vi "Main_V4.4.vi"() -> ()   [LabVIEW 2024]
uses:
  Facility_control_labview/Main_V3.0 Folder/Main_V3.0 Folder/C/Users/alexa/NewOrbit Dropbox/Alexander Schwertheim/PC (2)/Documents/Lab_hardware/Facility_control/Facility_control_labview/Controls/Turbo_Control_Mode.ctl
  Facility_control_labview/Main_V3.0 Folder/Main_V3.0 Folder/C/Users/alexa/NewOrbit Dropbox/Alexander Schwertheim/PC (2)/Documents/Lab_hardware/Facility_control/Facility_control_labview/Controls/Current_Facility_State.ctl
  Facility_control_labview/Main_V3.0 Folder/Main_V3.0 Folder/C/Users/alexa/NewOrbit Dropbox/Alexander Schwertheim/PC (2)/Documents/Lab_hardware/Facility_control/Facility_control_labview/Controls/Facility_State.ctl
  Facility_control_labview/Main_V3.0 Folder/Main_V3.0 Folder/C/Program Files/National Instruments/LabVIEW 2023/instr.lib/Pfeiffer Vacuum/Public/Turbopumps/PV Operating adjustment - Cluster.ctl
  Facility_control_labview/Main_V3.0 Folder/Main_V3.0 Folder/C/Program Files/National Instruments/LabVIEW 2023/instr.lib/Pfeiffer Vacuum/Public/Turbopumps/PV Miscellaneous - Cluster.ctl
  <vilib>/DAQmx/read.llb/DAQmx Read (Analog Wfm 1Chan 1Samp).vi
  <vilib>/DAQmx/read.llb/DAQmx Read (Digital Bool 1Line 1Point).vi
  <vilib>/DAQmx/read.llb/DAQmx Read (Analog 1D Wfm NChan NSamp).vi
  <vilib>/Analysis/baseanly.llb/Mean (DBL).vi
  <vilib>/DAQmx/read.llb/DAQmx Read (Digital 1D Bool NChan 1Samp 1Line).vi
  8e44a3b5-8466-4d68-80f5-cecf70b24b4a.vi
  <vilib>/DAQmx/write.llb/DAQmx Write (Digital Bool 1Line 1Point).vi
  <vilib>/DAQmx/write.llb/DAQmx Write (Digital 1D Bool NChan 1Samp 1Line).vi
  Program Files/National Instruments/LabVIEW 2023/instr.lib/U1250 Series Multimeter Device Driver/Public/Configure/Low Level/DC Voltage Configuration.vi
  <vilib>/DAQmx/create/channels.llb/DAQmx Create Channel (AI-Voltage-Basic).vi
  <vilib>/DAQmx/miscellaneous.llb/DAQmx Fill In Error Info.vi
  <vilib>/DAQmx/create/channels.llb/DAQmx Create Channel (DO-Digital Output).vi
  <vilib>/DAQmx/create/channels.llb/DAQmx Create Channel (DI-Digital Input).vi
  <vilib>/DAQmx/configure/timing.llb/DAQmx Timing (Sample Clock).vi
  Program Files/National Instruments/LabVIEW 2023/instr.lib/U1250 Series Multimeter Device Driver/Controls/Voltage Range.ctl
  Facility_control_labview/Main_V3.0 Folder/Main_V3.0 Folder/C/Program Files/National Instruments/LabVIEW 2023/instr.lib/Pfeiffer Vacuum/Pfeiffer Vacuum.lvlib
  <resource>/objmgr/daqmx.rc
  <vilib>/Analysis/NI_AALBase.lvlib
  Program Files/National Instruments/LabVIEW 2023/instr.lib/U1250 Series Multimeter Device Driver/U1250 Series Digital Multimeter.lvlib
panel:
  in  "Change to Auto":bool
  out "Turbo_Standby_Sys_Cmd":bool
  out "Measurement":dbl format="%#_8f"
  in  "ON/OFF":bool
  in  "DMM VISA resource name COM4":refnum<visa-resource-name>="COM4"
  in  "use DMM?":bool
  in  "samples per channel":i32=200
  in  "rate":dbl=1000.0 format="%#_13g"
  out "Com Potential (V)":dbl
  in  "Turbo on Threshold (torr) 2":dbl=0.25 format="%#_13g"
  out "Current Time/date":string
  out "String 3":string
  out "Vent Time (s) 2":dbl caption="Elapsed Time (s)"
  out "Numeric":dbl
  out "Elapsed Time (s)":dbl
  out "Turbo on Threshold (torr)":dbl=0.08
  out "Turbo Convectron":dbl=627.9033934565941 format="%_3e"
  out "Still Spinning?":bool
  out "Turbo Error Aknowleged 2":bool
  in  "Valve_Gate_User_Cmd":bool
  out "Tubro_Control_Mode":T1
  out "String":string
  out "Gate Valve Error?":bool
  out "Gate Valve":bool
  out "Valve_Gate_Sys_Cmd":bool
  out "Turbo Speed":string="0"
  out "Turbo bottom Temp":string="20"
  out "Turbo bearing Temp":string="21"
  out "Turbo Motor Temp":string="20"
  in  "Valve_Vent_User_Cmd":bool
  out "Vent Valve Error?":bool
  in  "Turbo_Error_Acknowlege_Cmd 2":bool
  in  "Valve_Bypass_User_Cmd":bool
  in  "Primary_User_Cmd":bool
  out "Primary Status":u32(colorbox)=12632256
  out "Bypass Valve Error?":bool
  in  "Turbo_Motor_User_Cmd":bool
  in  "Chiller_User_Cmd":bool
  out "Bypass Valve":bool
  out "Vent Valve":bool
  out "Primary Pump Status":string="Primary Pump is Off"
  out "Wide Range Gauge Pressure (Torr)":dbl=nan format="%_3e"
  out "Foreline Convectron":dbl=627.9033934565941 format="%_3e"
  out "Chiller Status":string="Chiller is Off"
  out "Turbo Status":string="Turbo Off"
  out "Turbo Error Aknowleged":bool
  out "Chiller Status 2":u32(colorbox)=12632256
  out "Turbo Status Color":u32(colorbox)=12632256
  in  "stop":bool
  out "error out":errorcluster
  out "Control Level":enum32{"Admin", "Debug", "Automatic"}(tab)=enum."Automatic"
  in  "Fake_Chiller_Read":bool
  in  "Fake_Convec_2_Pressure_Torr":dbl=0.0001 format="%_3e"
  in  "Fake_Primary_Pump_Read":bool
  in  "Fake_Valve_Turbo_Read":bool
  in  "Fake_Valve_Bypass_Read":bool
  in  "Fake_Valve_Vent_Read":bool
  in  "Use fake values?":bool=TRUE
  in  "Fake_Convec_1_Pressure_Torr":dbl=0.001 format="%_3e"
  in  "Fake Turbo Motor Read":bool
  in  "Fake Turbo Speed Read (%)":dbl=0.0001 format="%#.3f"
  in  "Fake Turbo Error Read":bool
  in  "Fake_Valve_Gate_Read":bool
  in  "Fake_WRG_Pressure_Torr":dbl=1e-05 format="%_3e"
  in  "Turbo Engage time":timestamp=timestamp(3765222000 s since 1904-01-01)
  out "Current Facility State":T2=enum."Pumping to Rough"
  out "Target Facility State":T2=enum."Pumping to Rough"
  out "Tab Control":T3(tab)
  in  "Pump to High Vac":bool
  in  "Pump to Rough":bool
  in  "Overnight Pump":bool
  in  "Vent":bool
  in  "Skip Primary Warm":bool
  in  "Vent 2":bool
  in  "Shut Off":bool
  in  "Overnight Pump 3":bool
  in  "Pump to Rough Only":bool
  in  "Pump to High":bool
  in  "Vent 4":bool
  in  "Pump to Rough 3":bool
  in  "Pump to High Vac 3":bool
  in  "Vent 5":bool
  in  "Shutdown":bool
  in  "Pump to Rough 4":bool
  in  "Overnight Pump 2":bool
  in  "Vent and shutdonw":bool
  in  "Shut Off":bool
  in  "Pump to Hi vac":bool
  in  "Overnight Pump 5":bool
  in  "Pump to Rough 5":bool
  in  "Pump to High Vac 2":bool
  in  "change_to_admin_mode":bool
  in  "Clear error?":bool
  out "Running":bool
  out "Waveform Chart 2":waveform(dbl)[](graph)=[{"t0"=timestamp(3754409348.7178025 s since 1904-01-01), "dt"=0.1, "Y"=array[1789 elements]}, {"t0"=timestamp(3754409348.7178025 s since 1904-01-01), "dt"=0.1, "Y"=array[1789 elements]}, {"t0"=timestamp(3754409348.7178025 s since 1904-01-01), "dt"=0.1, "Y"=array[1789 elements]}, {"t0"=timestamp(3754409348.7178025 s since 1904-01-01), "dt"=0.1, "Y"=array[1789 elements]}, {"t0"=timestamp(3754409348.7178025 s since 1904-01-01), "dt"=0.1, "Y"=array[1789 elements]}, {"t0"=timestamp(3754409348.7178025 s since 1904-01-01), "dt"=0.1, "Y"=array[1789 elements]}, {"t0"=timestamp(3754409348.7178025 s since 1904-01-01), "dt"=0.1, "Y"=array[1789 elements]}, {"t0"=timestamp(3754409348.7178025 s since 1904-01-01), "dt"=0.1, "Y"=array[1789 elements]}]
  out "Turbo Motor Read":bool
  out "Primary_Pump_Read":bool
  in  "Valve_Turbo_User_Cmd":bool
  out "Turbo Valve Error?":bool
  out "Turbo_Error_Acknowlege_Cmd":bool
  out "Turbo_Motor_Sys_Cmd":bool
  out "HP2300 RS485\nAddress":u16=2 min=1 max=999 step=1
  out "Chiller_Sys_Cmd":bool
  out "Valve_Vent_Sys_Cmd":bool
  out "Valve_Bypass_Sys_Cmd":bool
  out "Valve_Turbo_Sys_Cmd":bool
  out "Use_real_Values?":bool=TRUE
  out "Primary_Sys_Cmd":bool
  out "DAQ_Name":string="cDAQ1"
  out "Turbo Valve":bool
  out "String 4":string
  # "Torr"
  # "Pressure (Torr)"
  # "Speed (%):"
  # "Torr"
  # "On"
  # "Status"
  # "Torr"
  # "Off"
  # "Admin Mode Enabled"
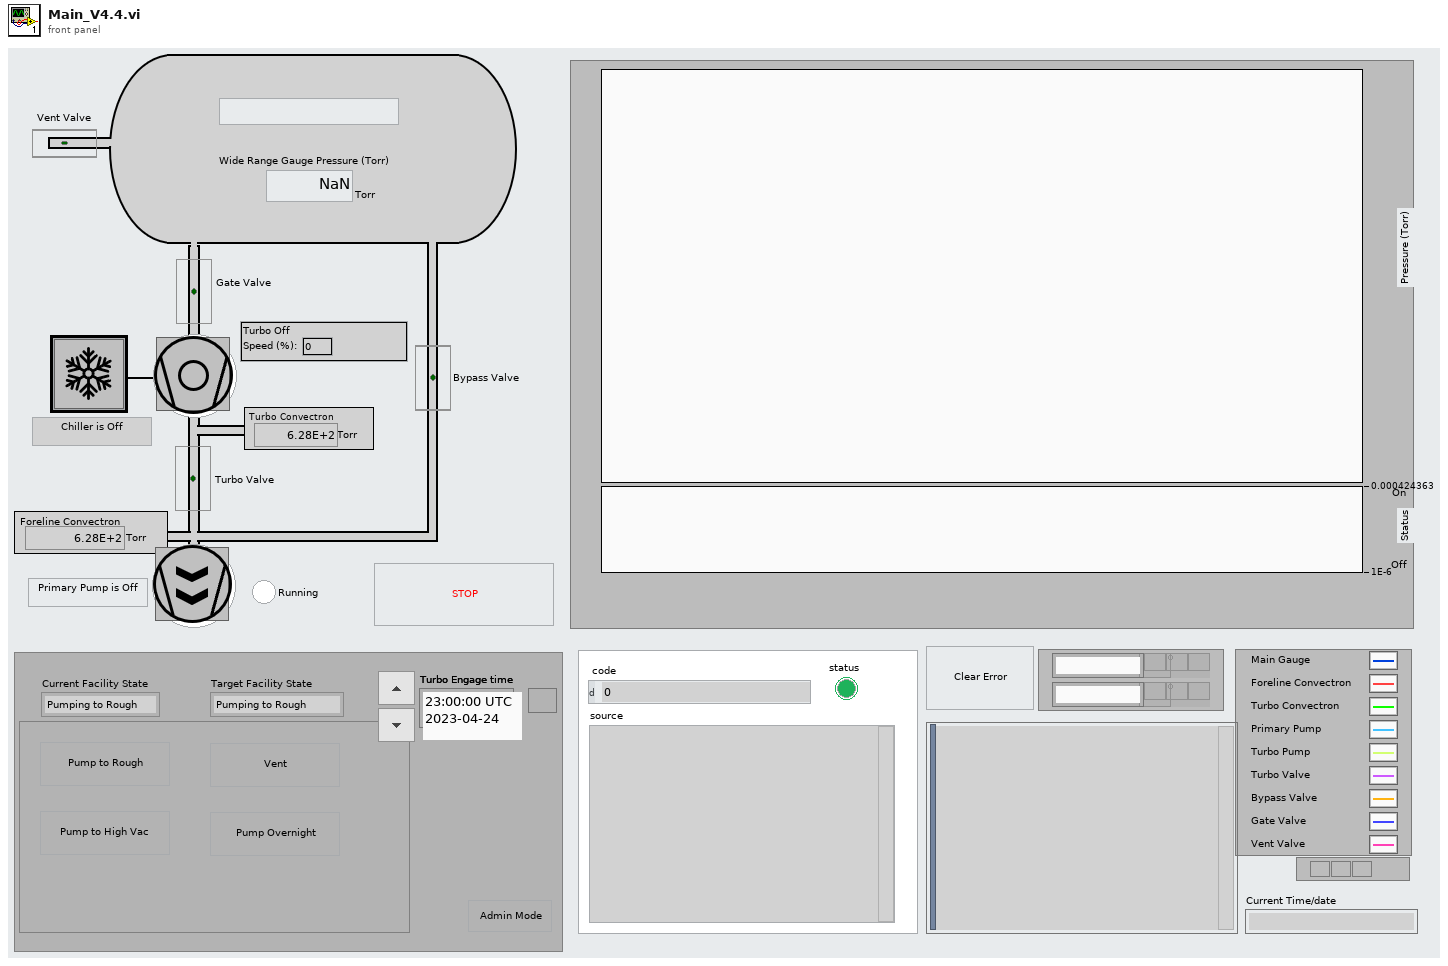
[diagram p1: front panel]
types:
  T1 = typedef "Turbo_Control_Mode.ctl" = enum16{"HP700_Turbo_DSUB25_Control", "HP700_Turbo_RS485_Control", "BigRed_Turbo_DSUB_15_Control", "BigRed_Turbo_RS485_Control", ""}
  T2 = typedef "Current_Facility_State.ctl" = enum16{"Facility Off", "Pumping to Rough", "Overnight Pump", "Engage Turbo", "Pumping to High Vac", "Disengage Turbo", "Vent and Shutdown", "Turbo slowing", "Venting"}
  T3 = enum32{"Facility Off", "Pumping to Rough", "Holding at Rough", "Overnight Pump", "Engaging Turbo", "Pumping to Hig Vac", "Closing Gate", "Venting", "Turbo Slowing"}
  T4 = typedef "Facility_State.ctl" = enum16{"Intialize", "Admin", "Manual", "Auto"}
  T5 = typedef "U1250 Series Digital Multimeter.lvlib/Voltage Range.ctl" = enum16{"5V", "50V", "500V", "1000V", "Auto"}
  T6 = typedef "Pfeiffer Vacuum.lvlib/PV Operating adjustment - Cluster.ctl" = cluster{"Parameter":u16, "Parameter\nread only<->describe":bool, "off<->on":bool, "Rotation speed set value\nin rot. speed setting\noperations [%]":dbl, "Preset rotation Speed\nat Standby mode (%)":dbl, "maximum power\nsetpoint [%]":i32, "Gas mode":u16}
  T7 = enum16{"temperature inverter [°C] (324)", "temperature electronic [°C] (326)", "temperature pump bottom [°C] (330)", "temperature bearing [°C] (342)", "temperature motor [°C] (346)", "temperature rotor [°C] (384)"}
  T8 = typedef "Pfeiffer Vacuum.lvlib/PV Miscellaneous - Cluster.ctl" = cluster{"Parameter":enum16{" Preselection brake", " Remote operations mode", " Actual error code (read only)", " Software version electronic drive unit  (read only)", " Software version display and control unit  (read only)", " Parameter set", " Contens of service line (TCM 1601 only)", " Unit adress", " Unit type electronic drive unit", " Error acknowledgement (write only)", " Keyboard interlock (008)", " Seal gas enable (050)"}, "Parameter\nread only<->describe":bool, "off<->on   ":bool, "Unit adress":i16, "Contens of service\nline; # of the 2nd\n parameter":i16}
  T9 = enum16{"Off", "Spinning Up", "Speed Reached", "Spinning Down", "Turbo in Standby", "Error"}
  T10 = enum16{"Off", "Spinning Up", "Speed Reached", "Spinning Down", "Turbo In Standby", "Error"}
  T11 = enum16{"Left Button", "Center Button", "Right Button", "Window Close"}
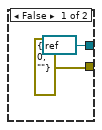
[diagram p3: hidden frame]
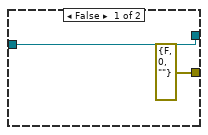
[diagram p4: hidden frame]
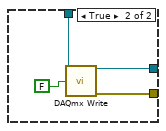
[diagram p5: hidden frame]
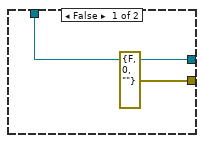
[diagram p6: hidden frame]
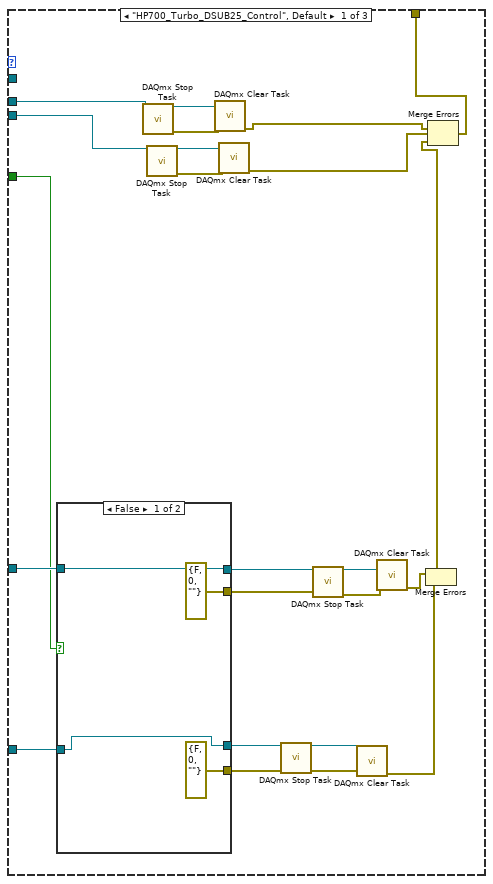
[diagram p7: hidden frame]
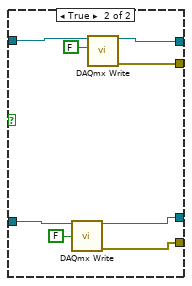
[diagram p8: hidden frame]
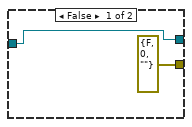
[diagram p9: hidden frame]
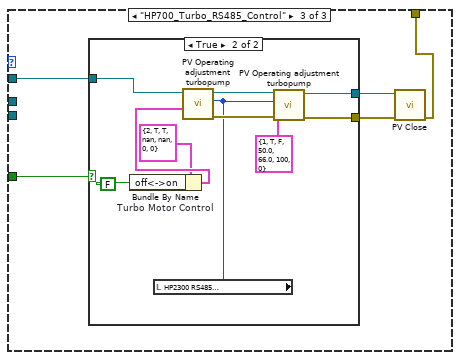
[diagram p10: hidden frame]
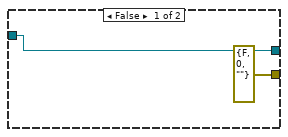
[diagram p11: hidden frame]
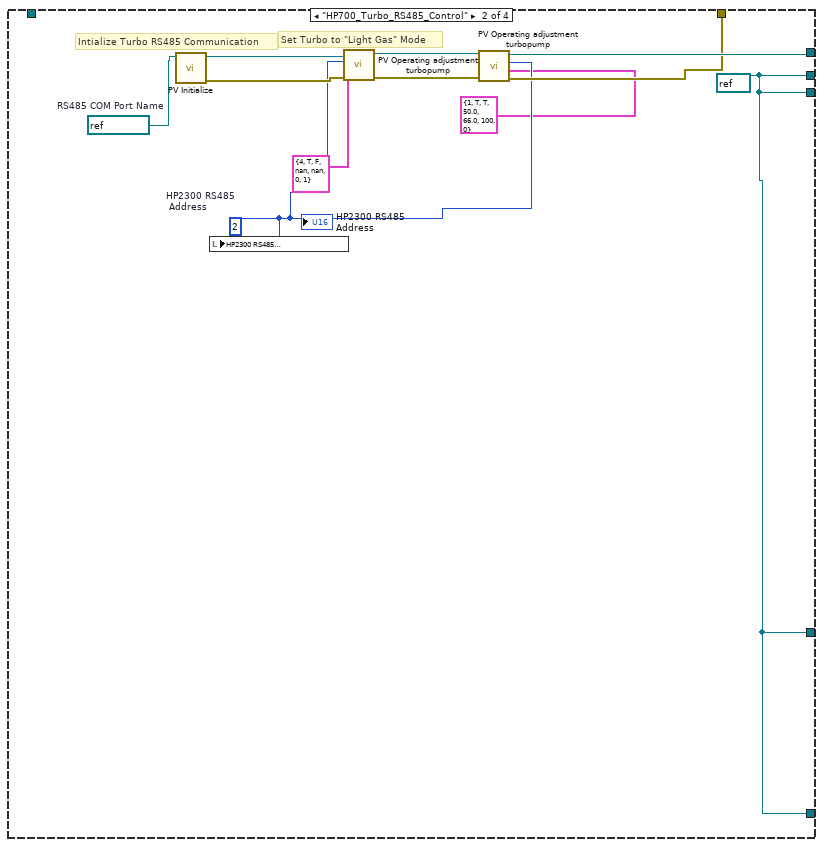
[diagram p12: hidden frame]
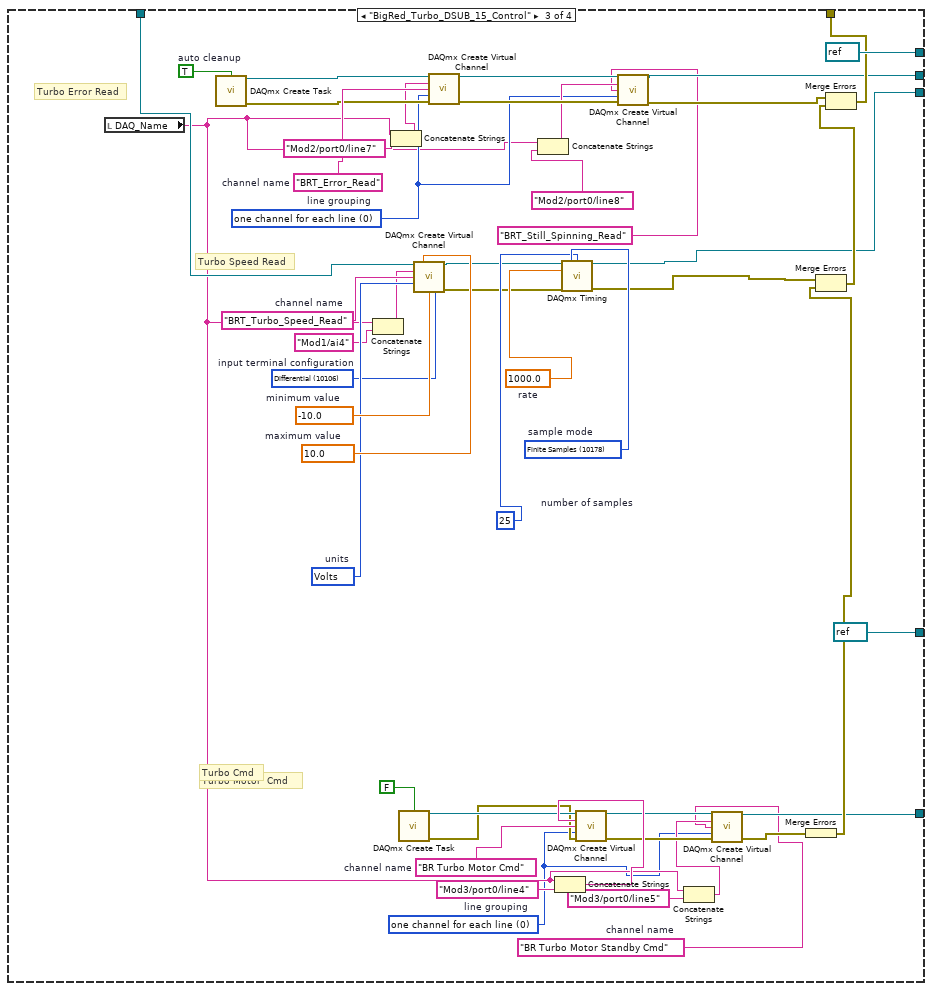
[diagram p13: hidden frame]
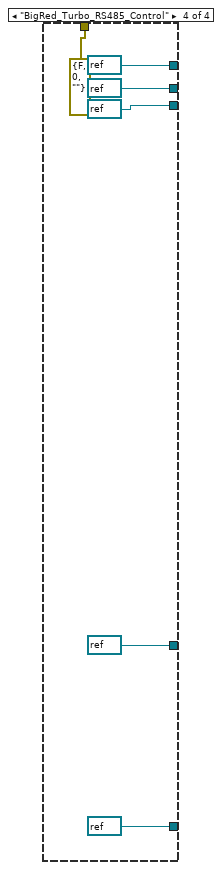
[diagram p14: hidden frame]
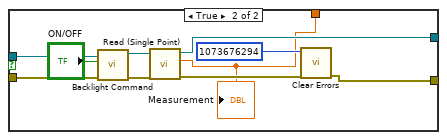
[diagram p15: hidden frame]
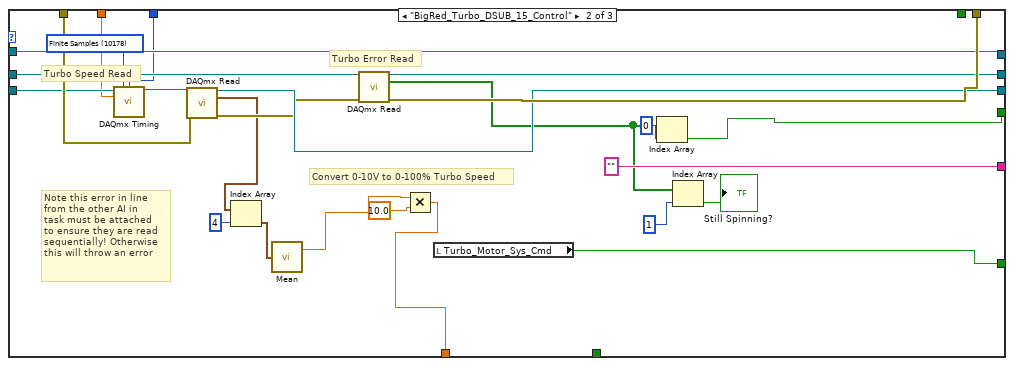
[diagram p16: hidden frame]
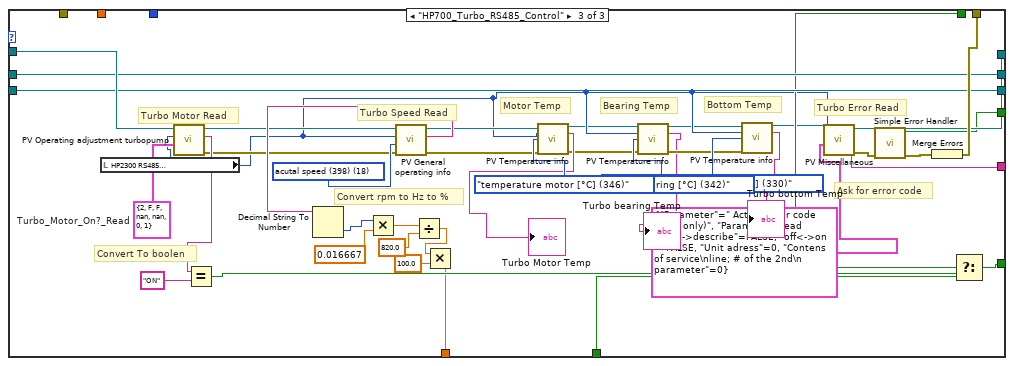
[diagram p17: hidden frame]
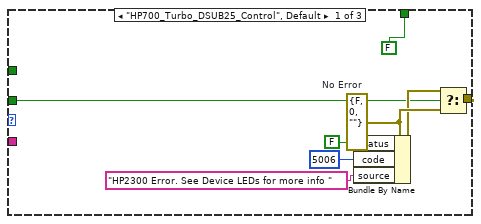
[diagram p18: hidden frame]
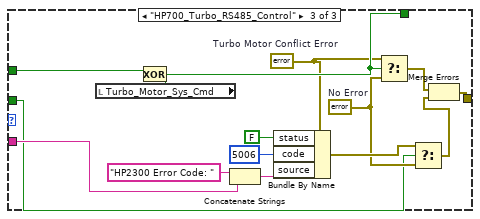
[diagram p19: hidden frame]
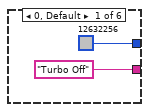
[diagram p20: hidden frame]
diagram:
  w3 = "cDAQ2Mod1/ai7"  # physical channel
  w12 = 10106 items=["Default"=-1, "RSE"=10083, "NRSE"=10078, "Differential"=10106, "Pseudodifferential"=12529] ("input terminal configuration")
  w13 = FALSE
  w21 = 4 items=["verify"=2, "reserve"=4, "commit"=3, "unreserve"=5, "abort"=6] ("action")
  w25 = 10178 items=["Finite Samples"=10178, "Continuous Samples"=10123, "Hardware Timed Single Point"=12522] ("sample mode")
  w37 = "Com Potential"  # channel name
  w38 = "Mod1/ai6"  # physical channel
  w39 = FALSE ("stop")
  w40 = 0  # Sub_state_iteration
  w41 = Current_Facility_State."Facility Off"  # Target Facility State
  w42 = Current_Facility_State."Facility Off"  # Current Facility State
  w47 = "Valve_Gate_Read"  # channel name
  w55 = Turbo_Control_Mode."BigRed_Turbo_DSUB_15_Control" ("Tubro_Control_Mode")
  w58 = "Valve_Gate_Cmd"  # channel name
  w66 = TRUE
  w5 = FALSE ("stop")
  w67 = 10.0  # Sample Freq (Hz)
  w73 = FALSE  # invert line
  w57 = FALSE
  (unwired) Facility_State."Intialize"
  w112 = 0 items=["one channel for each line", "one channel for all lines"]  # line grouping
  w107 = "Chiller_Cmd"  # channel name
  w110 = TRUE  # auto cleanup
  w120 = 0 items=["one channel for each line", "one channel for all lines"]  # line grouping
  w119 = "Chiller_Read"  # channel name
  w122 = TRUE  # auto cleanup
  w151 = "Convectron_2_Read"  # channel name
  w136 = "Mod1/ai2"  # physical channel
  w149 = "Convectron_1_Read"  # channel name
  w137 = "Mod1/ai1"  # physical channel
  w34 = 10106 items=["default"=-1, "RSE"=10083, "NRSE"=10078, "Differential"=10106, "Pseudodifferential"=12529]  # input terminal configuration
  w32 = 10348 items=["Volts"=10348, "From Custom Scale"=10065]  # units
  w146 = "Wide Range_Gauge_Read"  # channel name
  w35 = 0.0  # minimum value
  w33 = 10.0  # maximum value
  w140 = "Mod1/ai5"  # physical channel
  w143 = TRUE  # auto cleanup
  w182 = "Valve_Vent_Cmd"  # channel name
  w179 = "Valve_Bypass_Cmd"  # channel name
  w141 = 0 items=["one channel for each line", "one channel for all lines"]  # line grouping
  w176 = "Valve_Turbo_Cmd"  # channel name
  w174 = TRUE  # auto cleanup
  w203 = "Valve_Vent_Read"  # channel name
  w200 = "Valve_Bypass_Read"  # channel name
  w46 = 0 items=["one channel for each line", "one channel for all lines"]  # line grouping
  w197 = "Valve_Turbo_Read"  # channel name
  w195 = TRUE  # auto cleanup
  w204 = FALSE  # auto cleanup
  w217 = 0 items=["one channel for each line", "one channel for all lines"]  # line grouping
  w70 = "Primary_Pump_Read"  # channel name
  w215 = TRUE  # auto cleanup
  w223 = TRUE  # Real_DAQ?
  # "Turbo Standby ctrl"
  # "Force Stop on exit?"
  # "Init Chiller Cmd"
  # "Init Chiller Read"
  # "Init Gauge Read"
  # "Init Primary Pump Cmd"
  # "Init Valve Cmd"
  # "Init Valve Read"
  # "Init Primary Pump Read"
  n1 = Select(t="cDAQ1", s=w223, f="cDAQ2") -> (s? t:f=w224:string)
  "DAQ_Name" <- w224
  n2 = local write "Skip Primary Warm"(w5) -> ()
  n3 = local write "Valve_Turbo_Sys_Cmd"(w39) -> ()
  n4 = local write "Valve_Bypass_Sys_Cmd"(w39) -> ()
  n5 = local write "Valve_Vent_Sys_Cmd"(w39) -> ()
  n6 = local write "Valve_Gate_Sys_Cmd"(w39) -> ()
  n7 = local write "Primary_Sys_Cmd"(w39) -> ()
  n8 = local write "Chiller_Sys_Cmd"(w39) -> ()
  n9 = local write "Turbo_Motor_Sys_Cmd"(w39) -> ()
  n10 = local write "DAQ_Name"(w224) -> ()
  n11 = local write "stop"(w5) -> ()
  n12 = local write "Use_real_Values?"("Use fake values?") -> ()
  n13 = call <vilib>:"Clear Errors.vi"() -> ("error out"=w85:errorcluster)  [unwired: 6 in, 1 out]
  n14 = case shown="True" w13 {
    tunnel: [refnum<visa-resource-name> refnum ("VISA resource name out") w231] -> w17
    tunnel: [errorcluster {"status"=FALSE, "code"=0, "source"=""} ("error out") w230] -> w16
    frame False {
    }
    frame True {
      n15 = call "Initialize.vi"("Reset (True)"=TRUE, "ID Query (True)"=TRUE, "VISA resource name"="DMM VISA resource name COM4") -> ("error out"=w237:errorcluster, "VISA resource name out"=w239:refnum<visa-resource-name>)  [unwired: 7 in]
      n16 = call-poly "Measurement Configuration.vi"("error in (no error)"=w237, "Voltage Range"=Voltage_Range."50V", "VISA resource name"=w239) -> ("error out"=w234:errorcluster, "VISA resource name out"=w235:refnum<visa-resource-name>)  [unwired: 7 in]
      n17 = call "Backlight Command.vi"("error in (no error)"=w234, "ON/OFF"=TRUE, "VISA resource name"=w235) -> ("error out"=w230:errorcluster, "VISA resource name out"=w231:refnum<visa-resource-name>)  [unwired: 7 in]
    }
  }
  n18 = call <vilib>:"DAQmx Create Task.vi"("auto cleanup"=w174) -> ("task out"=w175:refnum<k21>, "error out"=w173:errorcluster)  [unwired: 13 in]
  n19 = call <vilib>:"DAQmx Create Task.vi"("auto cleanup"=w195, "error in"=w85) -> ("task out"=w196:refnum<k21>, "error out"=w194:errorcluster)  [unwired: 12 in]
  n20 = local read "DAQ_Name"() -> (w45:string)
  n21 = call <vilib>:"DAQmx Create Task.vi"("auto cleanup"=w143) -> ("task out"=w144:refnum<k21>, "error out"=w142:errorcluster)  [unwired: 13 in]
  n22 = local read "DAQ_Name"() -> (w60:string)
  n23 = local read "DAQ_Name"() -> (w31:string)
  n24 = Concatenate Strings(w60, "Mod4/port0/line0" ("lines")) -> (w166:string)
  n25 = Concatenate Strings(w45, "Mod2/port0/line2" ("lines")) -> (w192:string)
  n26 = Concatenate Strings(w31, w140) -> (w139:string)
  n27 = call-poly <vilib>:"DAQmx Create Virtual Channel.vi"("task in"=w196, "lines"=w192, "name to assign"=w197, "line grouping"=w46, "error in"=w194) -> ("task out"=w199:refnum<k21>, "error out"=w198:errorcluster)  [unwired: 9 in]
  n28 = call-poly <vilib>:"DAQmx Create Virtual Channel.vi"("task in"=w175, "lines"=w166, "name to assign"=w176, "line grouping"=w141, "error in"=w173) -> ("task out"=w178:refnum<k21>, "error out"=w177:errorcluster)  [unwired: 9 in]
  n29 = call-poly <vilib>:"DAQmx Create Virtual Channel.vi"("task in"=w144, "maximum value"=w33, "minimum value"=w35, "input terminal configuration"=w34, "physical channels"=w139, "name to assign"=w146, "units"=w32, "error in"=w142) -> ("task out"=w147:refnum<k21>, "error out"=w145:errorcluster)  [unwired: 6 in]
  n30 = Concatenate Strings(w45, "Mod2/port0/line3" ("lines")) -> (w189:string)
  n31 = Concatenate Strings(w60, "Mod4/port0/line1" ("lines")) -> (w168:string)
  n32 = call-poly <vilib>:"DAQmx Create Virtual Channel.vi"("task in"=w199, "lines"=w189, "name to assign"=w200, "line grouping"=w46, "error in"=w198) -> ("task out"=w202:refnum<k21>, "error out"=w201:errorcluster)  [unwired: 9 in]
  n33 = Concatenate Strings(w31, w137) -> (w138:string)
  n34 = call-poly <vilib>:"DAQmx Create Virtual Channel.vi"("task in"=w178, "lines"=w168, "name to assign"=w179, "line grouping"=w141, "error in"=w177) -> ("task out"=w181:refnum<k21>, "error out"=w180:errorcluster)  [unwired: 9 in]
  n35 = local write "Tubro_Control_Mode"(w55) -> ()
  n36 = call-poly <vilib>:"DAQmx Create Virtual Channel.vi"("task in"=w147, "maximum value"=w33, "minimum value"=w35, "input terminal configuration"=w34, "physical channels"=w138, "name to assign"=w149, "units"=w32, "error in"=w145) -> ("task out"=w150:refnum<k21>, "error out"=w148:errorcluster)  [unwired: 6 in]
  n37 = Concatenate Strings(w45, "Mod2/port0/line4" ("lines")) -> (w188:string)
  n38 = Concatenate Strings(w60, "Mod4/port0/line2" ("lines")) -> (w169:string)
  n39 = call <vilib>:"DAQmx Create Task.vi"("auto cleanup"=w215) -> ("task out"=w216:refnum<k21>, "error out"=w214:errorcluster)  [unwired: 13 in]
  n40 = Concatenate Strings(w31, w136) -> (w135:string)
  n41 = call <vilib>:"DAQmx Create Task.vi"("auto cleanup"=w122) -> ("task out"=w121:refnum<k21>, "error out"=w123:errorcluster)  [unwired: 13 in]
  n42 = call-poly <vilib>:"DAQmx Create Virtual Channel.vi"("task in"=w202, "lines"=w188, "name to assign"=w203, "line grouping"=w46, "error in"=w201) -> ("task out"=w52:refnum<k21>, "error out"=w50:errorcluster)  [unwired: 9 in]
  n43 = call <vilib>:"DAQmx Create Task.vi"("auto cleanup"=w110) -> ("task out"=w111:refnum<k21>, "error out"=w109:errorcluster)  [unwired: 13 in]
  n44 = call-poly <vilib>:"DAQmx Create Virtual Channel.vi"("task in"=w181, "lines"=w169, "name to assign"=w182, "line grouping"=w141, "error in"=w180) -> ("task out"=w64:refnum<k21>, "error out"=w62:errorcluster)  [unwired: 9 in]
  n45 = call <vilib>:"DAQmx Create Task.vi"("auto cleanup"=w204) -> ("task out"=w206:refnum<k21>, "error out"=w205:errorcluster)  [unwired: 13 in]
  n46 = call-poly <vilib>:"DAQmx Create Virtual Channel.vi"("task in"=w150, "maximum value"=w33, "minimum value"=w35, "input terminal configuration"=w34, "physical channels"=w135, "name to assign"=w151, "units"=w32, "error in"=w148) -> ("task out"=w36:refnum<k21>, "error out"=w29:errorcluster)  [unwired: 6 in]
  n47 = local read "DAQ_Name"() -> (w213:string)
  n48 = local read "DAQ_Name"() -> (w104:string)
  n49 = local read "DAQ_Name"() -> (w124:string)
  n50 = Concatenate Strings(w60, "Mod4/port0/line3" ("lines")) -> (w59:string)
  n51 = local read "DAQ_Name"() -> (w222:string)
  n52 = Concatenate Strings(w45, "Mod2/port0/line5" ("lines")) -> (w48:string)
  n53 = call-poly <vilib>:"DAQmx Create Virtual Channel.vi"("task in"=w64, "lines"=w59, "name to assign"=w58, "error in"=w62) -> ("task out"=w63:refnum<k21>, "error out"=w61:errorcluster)  [unwired: 10 in]
  n54 = Concatenate Strings(w213, "Mod2/port0/line0" ("lines")) -> (w211:string)
  n55 = call-poly <vilib>:"DAQmx Create Virtual Channel.vi"("task in"=w52, "lines"=w48, "name to assign"=w47, "line grouping"=w46, "error in"=w50) -> ("task out"=w51:refnum<k21>, "error out"=w49:errorcluster)  [unwired: 9 in]
  n56 = Concatenate Strings(w124, "Mod2/port0/line1" ("lines")) -> (w126:string)
  n57 = Concatenate Strings(w31, w38) -> (w30:string)
  n58 = Concatenate Strings(w104, "Mod3/port0/line1" ("lines")) -> (w105:string)
  n59 = Concatenate Strings(w222, "Mod3/port0/line0" ("lines")) -> (w220:string)
  n60 = call-poly <vilib>:"DAQmx Create Virtual Channel.vi"("task in"=w36, "maximum value"=w33, "minimum value"=w35, "input terminal configuration"=w34, "physical channels"=w30, "name to assign"=w37, "units"=w32, "error in"=w29) -> ("task out"=w28:refnum<k21>, "error out"=w27:errorcluster)  [unwired: 6 in]
  n61 = call-poly <vilib>:"DAQmx Create Virtual Channel.vi"("task in"=w216, "lines"=w211, "name to assign"=w70, "line grouping"=w217, "error in"=w214) -> ("task out"=w72:refnum<k21>, "error out"=w172:errorcluster)  [unwired: 9 in]
  n62 = property class="DAQmx Channel"(reference=w72, "Active Channels (if subset)"=w70, "Digital Input:Invert Lines"=w73) -> (reference out=w71:refnum<k21>)  [unwired: 1 in, 1 out]
  n63 = call-poly <vilib>:"DAQmx Create Virtual Channel.vi"("task in"=w121, "lines"=w126, "name to assign"=w119, "line grouping"=w120, "error in"=w123) -> ("task out"=w118:refnum<k21>, "error out"=w103:errorcluster)  [unwired: 9 in]
  n64 = call-poly <vilib>:"DAQmx Create Virtual Channel.vi"("task in"=w206, "lines"=w220, "name to assign"="Primary_Pump_Cmd", "error in"=w205) -> ("task out"=w219:refnum<k21>, "error out"=w134:errorcluster)  [unwired: 10 in]
  n65 = call-poly <vilib>:"DAQmx Create Virtual Channel.vi"("task in"=w111, "lines"=w105, "name to assign"=w107, "line grouping"=w112, "error in"=w109) -> ("task out"=w108:refnum<k21>, "error out"=w101:errorcluster)  [unwired: 9 in]
  n66 = call-poly <vilib>:"DAQmx Timing.vi"("task/channels in"=w28, "sample mode"=w25, "samples per channel"=25, "rate"=1000.0, "error in"=w27) -> ("task out"=w22:refnum<k21>, "error out"=w20:errorcluster)  [unwired: 9 in]
  n67 = call <vilib>:"DAQmx Control Task.vi"("task/channels in"=w22, "action"=w21, "error in"=w20) -> ("task out"=w18:refnum<k21>, "error out"=w19:errorcluster)  [unwired: 11 in]
  n68 = case shown="\"HP700_Turbo_DSUB25_Control\", Default" w55 {
    tunnel: [w277 w289 w339 errorcluster {"status"=FALSE, "code"=0, "source"=""} ("error out")] -> w97
    tunnel: [refnum<visa-resource-name> refnum ("dup VISA session") w291 refnum<visa-resource-name> refnum ("dup VISA session") refnum<visa-resource-name> refnum ("dup VISA session")] -> w84
    tunnel: [w280 w293 w314 refnum<k21> refnum ("task out")] -> w83
    tunnel: [w244 w293 w298 refnum<k21> refnum ("task out")] -> w4
    tunnel: [w249 w293 refnum<k21> refnum ("task out") refnum<k21> refnum ("task out")] -> w80
    tunnel: [w248 w293 w305 refnum<k21> refnum ("task out")] -> w78
    tunnel: w18 -> [w240 _ w307 _]
    frame "HP700_Turbo_DSUB25_Control", Default {
      w247 = 10178 items=["Finite Samples"=10178, "Continuous Samples"=10123, "Hardware Timed Single Point"=12522]  # sample mode
      w246 = 50  # number of samples
      w245 = 4000.0  # rate
      w260 = 1 items=["one channel for each line", "one channel for all lines"]  # line grouping
      w259 = "HP700 Motor Cmd"  # channel name
      w266 = "Turbo Error Acknowledged Cmd"  # channel name
      w272 = 10106 items=["default"=-1, "RSE"=10083, "NRSE"=10078, "Differential"=10106, "Pseudodifferential"=12529]  # input terminal configuration
      w273 = 10348 items=["Volts"=10348, "From Custom Scale"=10065]  # units
      w274 = "Turbo_Speed_Read"  # channel name
      w275 = 0.0  # minimum value
      w276 = 10.0  # maximum value
      w285 = 0 items=["one channel for each line", "one channel for all lines"]  # line grouping
      w286 = "HP700_Error_Read"  # channel name
      w267 = TRUE  # auto cleanup
      # "Turbo Motor  Cmd"
      # "Turbo Error Acknoledged  Cmd"
      # "Turbo Cmd"
      # "Turbo Speed Read"
      # "Turbo Error Read"
      n69 = local read "DAQ_Name"() -> (w256:string)
      n70 = Concatenate Strings(w256, "Mod1/ai3" ("physical channel")) -> (w270:string)
      n71 = call <vilib>:"DAQmx Create Task.vi"("auto cleanup"=w267) -> ("task out"=w284:refnum<k21>, "error out"=w283:errorcluster)  [unwired: 13 in]
      n72 = call <vilib>:"DAQmx Create Task.vi"("auto cleanup"=FALSE) -> ("task out"=w258:refnum<k21>, "error out"=w257:errorcluster)  [unwired: 13 in]
      n73 = call <vilib>:"DAQmx Create Task.vi"("auto cleanup"=FALSE) -> ("task out"=w254:refnum<k21>, "error out"=w253:errorcluster)  [unwired: 13 in]
      n74 = call-poly <vilib>:"DAQmx Create Virtual Channel.vi"("task in"=w240, "maximum value"=w276, "minimum value"=w275, "input terminal configuration"=w272, "physical channels"=w270, "name to assign"=w274, "units"=w273) -> ("task out"=w243:refnum<k21>, "error out"=w242:errorcluster)  [unwired: 7 in]
      n75 = Concatenate Strings(w256, "Mod2/port0/line6" ("lines")) -> (w281:string)
      n76 = Concatenate Strings(w256, "Mod3/port0/line2" ("lines")) -> (w262:string)
      n77 = Concatenate Strings(w256, "Mod3/port0/line3" ("lines")) -> (w265:string)
      n78 = call-poly <vilib>:"DAQmx Timing.vi"("task/channels in"=w243, "sample mode"=w247, "samples per channel"=w246, "rate"=w245, "error in"=w242) -> ("task out"=w244:refnum<k21>, "error out"=w241:errorcluster)  [unwired: 9 in]
      n79 = call-poly <vilib>:"DAQmx Create Virtual Channel.vi"("task in"=w258, "lines"=w262, "name to assign"=w259, "line grouping"=w260, "error in"=w257) -> ("task out"=w248:refnum<k21>, "error out"=w252:errorcluster)  [unwired: 9 in]
      n80 = call-poly <vilib>:"DAQmx Create Virtual Channel.vi"("task in"=w254, "lines"=w265, "name to assign"=w266, "error in"=w253) -> ("task out"=w249:refnum<k21>, "error out"=w251:errorcluster)  [unwired: 10 in]
      n81 = call-poly <vilib>:"DAQmx Create Virtual Channel.vi"("task in"=w284, "lines"=w281, "name to assign"=w286, "line grouping"=w285, "error in"=w283) -> ("task out"=w280:refnum<k21>, "error out"=w278:errorcluster)  [unwired: 9 in]
      n82 = Merge Errors(w252) -> (w250:errorcluster)
      n83 = Merge Errors(w251, w250) -> (w268:errorcluster)
      n84 = Merge Errors(w241, w268) -> (w269:errorcluster)
      n85 = Merge Errors(w278, w269) -> (w277:errorcluster)
    }
    frame "HP700_Turbo_RS485_Control" {
      w293 = refnum<k21> refnum ("task out")
      w288 = u16 2  # HP2300 RS485  Address
      w297 = refnum<visa-resource-name> "COM4"  # RS485 COM Port Name
      # "Intialize Turbo RS485 Communication"
      # "Set Turbo to \"Light Gas\" Mode"
      n86 = call "PV Initialize.vi"("VISA session in"=w297) -> ("error out"=w295:errorcluster, "VISA session out"=w296:refnum<visa-resource-name>)  [unwired: 9 in]
      n87 = local write "HP2300 RS485\nAddress"(w288) -> ()
      n88 = call "PV Operating adjustment turbopump.vi"("error in (no error)"=w295, "Operating adjustment - Cluster"=T6 {"Parameter"=4, "Parameter\nread only<->describe"=TRUE, "off<->on"=FALSE, "Rotation speed set value\nin rot. speed setting\noperations [%]"=nan, "Preset rotation Speed\nat Standby mode (%)"=nan, "maximum power\nsetpoint [%]"=0, "Gas mode"=1}, "Adress of unit"=w288, "VISA session"=w296) -> ("error out"=w290:errorcluster, "dup VISA session"=w292:refnum<visa-resource-name>)  [unwired: 5 in, 1 out]
      n89 = call "PV Operating adjustment turbopump.vi"("error in (no error)"=w290, "Operating adjustment - Cluster"=T6 {"Parameter"=1, "Parameter\nread only<->describe"=TRUE, "off<->on"=TRUE, "Rotation speed set value\nin rot. speed setting\noperations [%]"=50.0, "Preset rotation Speed\nat Standby mode (%)"=66.0, "maximum power\nsetpoint [%]"=100, "Gas mode"=0}, "Adress of unit"=w288, "VISA session"=w292) -> ("error out"=w289:errorcluster, "dup VISA session"=w291:refnum<visa-resource-name>)  [unwired: 5 in, 1 out]
      "HP2300 RS485\nAddress" <- w288
    }
    frame "BigRed_Turbo_DSUB_15_Control" {
      w301 = "BR Turbo Motor Standby Cmd"  # channel name
      w322 = 10178 items=["Finite Samples"=10178, "Continuous Samples"=10123, "Hardware Timed Single Point"=12522]  # sample mode
      w321 = 25  # number of samples
      w320 = 1000.0  # rate
      w300 = 0 items=["one channel for each line", "one channel for all lines"]  # line grouping
      w326 = "BR Turbo Motor Cmd"  # channel name
      w334 = 10106 items=["default"=-1, "RSE"=10083, "NRSE"=10078, "Differential"=10106, "Pseudodifferential"=12529]  # input terminal configuration
      w335 = 10348 items=["Volts"=10348, "From Custom Scale"=10065]  # units
      w336 = "BRT_Turbo_Speed_Read"  # channel name
      w337 = -10.0  # minimum value
      w338 = 10.0  # maximum value
      w310 = 0 items=["one channel for each line", "one channel for all lines"]  # line grouping
      w345 = "BRT_Error_Read"  # channel name
      w330 = TRUE  # auto cleanup
      # "Turbo Motor  Cmd"
      # "Turbo Cmd"
      # "Turbo Speed Read"
      # "Turbo Error Read"
      n90 = local read "DAQ_Name"() -> (w303:string)
      n91 = call <vilib>:"DAQmx Create Task.vi"("auto cleanup"=w330) -> ("task out"=w344:refnum<k21>, "error out"=w343:errorcluster)  [unwired: 13 in]
      n92 = Concatenate Strings(w303, "Mod1/ai4" ("physical channel")) -> (w332:string)
      n93 = Concatenate Strings(w303, "Mod2/port0/line7" ("lines")) -> (w341:string)
      n94 = call <vilib>:"DAQmx Create Task.vi"("auto cleanup"=FALSE) -> ("task out"=w325:refnum<k21>, "error out"=w324:errorcluster)  [unwired: 13 in]
      n95 = call-poly <vilib>:"DAQmx Create Virtual Channel.vi"("task in"=w307, "maximum value"=w338, "minimum value"=w337, "input terminal configuration"=w334, "physical channels"=w332, "name to assign"=w336, "units"=w335) -> ("task out"=w319:refnum<k21>, "error out"=w318:errorcluster)  [unwired: 7 in]
      n96 = call-poly <vilib>:"DAQmx Create Virtual Channel.vi"("task in"=w344, "lines"=w341, "name to assign"=w345, "line grouping"=w310, "error in"=w343) -> ("task out"=w315:refnum<k21>, "error out"=w312:errorcluster)  [unwired: 9 in]
      n97 = Concatenate Strings(w303, "Mod2/port0/line8" ("lines")) -> (w311:string)
      n98 = Concatenate Strings(w303, "Mod3/port0/line4" ("lines")) -> (w328:string)
      n99 = call-poly <vilib>:"DAQmx Timing.vi"("task/channels in"=w319, "sample mode"=w322, "samples per channel"=w321, "rate"=w320, "error in"=w318) -> ("task out"=w298:refnum<k21>, "error out"=w299:errorcluster)  [unwired: 9 in]
      n100 = call-poly <vilib>:"DAQmx Create Virtual Channel.vi"("task in"=w325, "lines"=w328, "name to assign"=w326, "line grouping"=w300, "error in"=w324) -> ("task out"=w306:refnum<k21>, "error out"=w323:errorcluster)  [unwired: 9 in]
      n101 = call-poly <vilib>:"DAQmx Create Virtual Channel.vi"("task in"=w315, "lines"=w311, "name to assign"="BRT_Still_Spinning_Read" ("string"), "line grouping"=w310, "error in"=w312) -> ("task out"=w314:refnum<k21>, "error out"=w313:errorcluster)  [unwired: 9 in]
      n102 = Concatenate Strings(w303, "Mod3/port0/line5" ("lines")) -> (w302:string)
      n103 = call-poly <vilib>:"DAQmx Create Virtual Channel.vi"("task in"=w306, "lines"=w302, "name to assign"=w301, "line grouping"=w300) -> ("task out"=w305:refnum<k21>)  [unwired: 10 in, 1 out]
      n104 = Merge Errors(w323) -> (w317:errorcluster)
      n105 = Merge Errors(w299, w317) -> (w331:errorcluster)
      n106 = Merge Errors(w313, w331) -> (w339:errorcluster)
    }
    frame "BigRed_Turbo_RS485_Control" {
    }
  }
  n107 = Merge Errors(w61, w172) -> (w171:errorcluster)
  n108 = Merge Errors(w49, w171) -> (w210:errorcluster)
  n109 = Merge Errors(w97) -> (w98:errorcluster)
  n110 = Merge Errors(w101, w98) -> (w100:errorcluster)
  n111 = Merge Errors(w103, w100) -> (w102:errorcluster)
  n112 = Merge Errors(w19, w102) -> (w23:errorcluster)
  n113 = Merge Errors(w134, w23) -> (w133:errorcluster)
  n114 = Merge Errors(w172, w133) -> ()  [unwired: 1 out]
  n115 = call-poly <vilib>:"DAQmx Create Virtual Channel.vi"("input terminal configuration"=w12, "physical channels"=w3, "name to assign"="Dummy Variable to get nice time data") -> ("task out"=w2:refnum<k21>, "error out"=w1:errorcluster)  [unwired: 11 in]
  n116 = Divide(x=1.0, y=w67) -> (x/y=w69:dbl)
  n117 = while {
    shift-right: [w580] -> _
    shift-left: w210 -> [w583]
    tunnel: w71 -> [w584]
    tunnel: w219 -> [w564]
    tunnel: [w574] -> w159
    tunnel: w51 -> [w573]
    tunnel: [w572] -> _
    tunnel: [w566] -> w185
    tunnel: [w556] -> w184
    tunnel: w63 -> [w555]
    tunnel: [w551] -> w162
    tunnel: w18 -> [w545]
    tunnel: [w537] -> w132
    tunnel: w118 -> [w535]
    tunnel: [w530] -> w115
    tunnel: w108 -> [w527]
    tunnel: [w517] -> w99
    tunnel: [w501] -> w96
    tunnel: w84 -> [w498]
    tunnel: w83 -> [w497]
    tunnel: [w491] -> w82
    tunnel: w4 -> [w490]
    tunnel: [w484] -> w81
    tunnel: w80 -> [w482]
    tunnel: [w478] -> w44
    shift-right: [w475] -> _
    shift-left: FALSE -> [w476]
    tunnel: w78 -> [w473]
    tunnel: [w468] -> w77
    shift-right: [w463] -> _
    shift-left: FALSE -> [w465]
    shift-right: [w457] -> _
    shift-left: FALSE -> [w459]
    shift-right: [w452] -> _
    shift-left: w57 -> [w454]
    shift-right: [w415] -> _
    shift-left: w57 -> [w443]
    shift-right: [w445] -> _
    shift-left: w57 -> [w444]
    shift-right: [w439] -> _
    shift-left: FALSE -> [w381]
    shift-right: [w414] -> _
    shift-left: w57 -> [w410]
    shift-right: [w407] -> _
    shift-left: "" -> [w406]
    shift-right: [w396] -> _
    shift-left: Facility_State."Intialize" -> [w399]
    shift-right: [w393] -> _
    shift-left: w42 -> [w391]
    shift-right: [w382] -> _
    shift-left: w41 -> [w392]
    shift-right: [w374] -> _
    shift-left: w40 -> [w380]
    tunnel: w13 -> [w373]
    tunnel: w17 -> [w372]
    tunnel: w16 -> [w371]
    tunnel: [w360] -> w15
    tunnel: [w359] -> w14
    shift-right: [w356] -> _
    shift-left: FALSE -> [w355]
    stop <- "stop" stop-if-true
    n118 = flat-sequence {
      tunnel: w584 -> [w687]
      tunnel: w583 -> [w686]
      tunnel: [w685] -> w579
      tunnel: [w625] -> w577
      tunnel: w573 -> [w683]
      tunnel: [w682] -> w572
      tunnel: [w679] -> w571
      tunnel: [w675] -> w570
      tunnel: [w674] -> w565
      tunnel: w564 -> [w674]
      tunnel: [w673] -> w560
      tunnel: w555 -> [w672]
      tunnel: [w672] -> w552
      tunnel: w545 -> [w608]
      tunnel: [w664] -> w544
      tunnel: [w661] -> w543
      tunnel: [w609] -> w541
      tunnel: [w667] -> w536
      tunnel: w535 -> [w657]
      tunnel: [w656] -> w533
      tunnel: [w652] -> w529
      tunnel: [w649] -> w528
      tunnel: w527 -> [w649]
      tunnel: [w643] -> w519
      tunnel: [w626] -> w514
      tunnel: [w646] -> w513
      tunnel: [w638] -> w512
      tunnel: [w645] -> w502
      tunnel: w498 -> [w644]
      tunnel: w497 -> [w642]
      tunnel: [w641] -> w496
      tunnel: w490 -> [w640]
      tunnel: [w639] -> w489
      tunnel: [w636] -> w483
      tunnel: w482 -> [w636]
      tunnel: [w635] -> w474
      tunnel: w473 -> [w635]
      tunnel: w465 -> [w634]
      tunnel: [w634] -> w466
      tunnel: [w633] -> w460
      tunnel: w459 -> [w633]
      tunnel: [w632] -> w455
      tunnel: w454 -> [w632]
      tunnel: [w631] -> w449
      tunnel: [w630] -> w448
      tunnel: w444 -> [w631]
      tunnel: w443 -> [w630]
      tunnel: [w629] -> w441
      tunnel: w381 -> [w629]
      tunnel: w410 -> [w621]
      tunnel: [w621] -> w411
      tunnel: w406 -> [w619]
      tunnel: [w619] -> w405
      tunnel: w392 -> [w614]
      tunnel: w391 -> [w615]
      tunnel: [w615] -> w390
      tunnel: [w614] -> w387
      tunnel: w380 -> [w613]
      tunnel: [w613] -> w379
      tunnel: w373 -> [w587]
      tunnel: w372 -> [w593]
      tunnel: w371 -> [w592]
      tunnel: [w591] -> w370
      tunnel: [w590] -> w369
      tunnel: w355 -> [w585]
      tunnel: [w585] -> w354
      tunnel: w579 -> [w900]
      tunnel: [w901] -> w578
      tunnel: w577 -> [w839]
      tunnel: w571 -> [w831]
      tunnel: w570 -> [w896]
      tunnel: [w896] -> w569
      tunnel: w565 -> [w895]
      tunnel: [w895] -> w563
      tunnel: w560 -> [w894]
      tunnel: [w894] -> w557
      tunnel: [w891] -> w553
      tunnel: w552 -> [w891]
      tunnel: w544 -> [w821]
      tunnel: w543 -> [w834]
      tunnel: [w877] -> w542
      tunnel: w541 -> [w877]
      tunnel: w536 -> [w795]
      tunnel: [w876] -> w534
      tunnel: w533 -> [w876]
      tunnel: w529 -> [w841]
      tunnel: w528 -> [w869]
      tunnel: [w869] -> w526
      tunnel: [w867] -> w520
      tunnel: w519 -> [w867]
      tunnel: w514 -> [w838]
      tunnel: w513 -> [w840]
      tunnel: w512 -> [w816]
      tunnel: w502 -> [w855]
      tunnel: w496 -> [w854]
      tunnel: [w854] -> w495
      tunnel: w489 -> [w853]
      tunnel: [w853] -> w488
      tunnel: w483 -> [w852]
      tunnel: [w852] -> w481
      tunnel: w474 -> [w849]
      tunnel: [w849] -> w472
      tunnel: [w848] -> w467
      tunnel: w466 -> [w848]
      tunnel: [w847] -> w461
      tunnel: w460 -> [w847]
      tunnel: [w846] -> w456
      tunnel: w455 -> [w846]
      tunnel: [w844] -> w451
      tunnel: [w845] -> w450
      tunnel: w449 -> [w845]
      tunnel: w448 -> [w844]
      tunnel: [w843] -> w442
      tunnel: w441 -> [w843]
      tunnel: [w837] -> w437
      tunnel: [w836] -> w436
      tunnel: [w835] -> w434
      tunnel: [w839] -> w432
      tunnel: [w795] -> w429
      tunnel: [w821] -> w427
      tunnel: [w834] -> w425
      tunnel: [w841] -> w423
      tunnel: [w840] -> w421
      tunnel: [w838] -> w420
      tunnel: [w832] -> w412
      tunnel: w411 -> [w832]
      tunnel: [w824] -> w409
      tunnel: w405 -> [w823]
      tunnel: [w823] -> w404
      tunnel: w390 -> [w820]
      tunnel: [w820] -> w389
      tunnel: w387 -> [w819]
      tunnel: [w819] -> w386
      tunnel: w379 -> [w814]
      tunnel: [w814] -> w378
      tunnel: w370 -> [w805]
      tunnel: w369 -> [w804]
      tunnel: [w805] -> w368
      tunnel: [w804] -> w367
      tunnel: w354 -> [w801]
      tunnel: [w801] -> w353
      tunnel: w578 -> [w973]
      tunnel: [w977] -> w582
      tunnel: [w972] -> w581
      tunnel: w569 -> [w1004]
      tunnel: [w1004] -> w568
      tunnel: w563 -> [w1003]
      tunnel: [w1003] -> w562
      tunnel: [w1002] -> w558
      tunnel: w557 -> [w1002]
      tunnel: [w1001] -> w554
      tunnel: w553 -> [w1001]
      tunnel: [w980] -> w550
      tunnel: [w978] -> w549
      tunnel: w542 -> [w1000]
      tunnel: [w1000] -> w539
      tunnel: w534 -> [w999]
      tunnel: [w999] -> w531
      tunnel: w526 -> [w998]
      tunnel: [w998] -> w525
      tunnel: [w976] -> w523
      tunnel: [w997] -> w521
      tunnel: w520 -> [w997]
      tunnel: [w975] -> w516
      tunnel: ["Turbo_Error_Acknowlege_Cmd 2"] -> w500
      tunnel: w495 -> [w995]
      tunnel: [w995] -> w494
      tunnel: w488 -> [w994]
      tunnel: [w994] -> w487
      tunnel: w481 -> [w993]
      tunnel: [w993] -> w480
      tunnel: w472 -> [w992]
      tunnel: [w992] -> w471
      tunnel: w467 -> [w977]
      tunnel: w461 -> [w976]
      tunnel: w456 -> [w980]
      tunnel: w451 -> [w978]
      tunnel: w450 -> [w979]
      tunnel: w442 -> [w975]
      tunnel: [w990] -> w438
      tunnel: w437 -> [w990]
      tunnel: w436 -> [w989]
      tunnel: [w989] -> w435
      tunnel: w434 -> [w988]
      tunnel: [w988] -> w433
      tunnel: w432 -> [w987]
      tunnel: [w987] -> w431
      tunnel: [w986] -> w430
      tunnel: w429 -> [w986]
      tunnel: [w985] -> w428
      tunnel: w427 -> [w985]
      tunnel: [w984] -> w426
      tunnel: w425 -> [w984]
      tunnel: [w983] -> w424
      tunnel: w423 -> [w983]
      tunnel: [w982] -> w422
      tunnel: w421 -> [w982]
      tunnel: w420 -> [w981]
      tunnel: [w981] -> w419
      tunnel: [w979] -> w418
      tunnel: [w971] -> w413
      tunnel: w412 -> [w971]
      tunnel: w409 -> [w970]
      tunnel: [w970] -> w408
      tunnel: w404 -> [w969]
      tunnel: [w969] -> w403
      tunnel: w389 -> [w968]
      tunnel: [w968] -> w388
      tunnel: w386 -> [w967]
      tunnel: [w967] -> w385
      tunnel: w378 -> [w966]
      tunnel: [w966] -> w377
      tunnel: w368 -> [w965]
      tunnel: w367 -> [w964]
      tunnel: [w965] -> w366
      tunnel: [w964] -> w365
      tunnel: w353 -> [w963]
      tunnel: [w963] -> w352
      tunnel: w582 -> [w1079]
      tunnel: w581 -> [w1078]
      tunnel: [w1077] -> w576
      tunnel: [w1076] -> w575
      tunnel: w568 -> [w1069]
      tunnel: [w1069] -> w567
      tunnel: w562 -> [w1070]
      tunnel: [w1070] -> w561
      tunnel: [w1068] -> w559
      tunnel: w558 -> [w1068]
      tunnel: w554 -> [w1071]
      tunnel: w550 -> [w1075]
      tunnel: w549 -> [w1073]
      tunnel: [w1032] -> w548
      tunnel: [w1072] -> w547
      tunnel: [w1031] -> w546
      tunnel: [w1071] -> w540
      tunnel: w539 -> [w1067]
      tunnel: [w1067] -> w538
      tunnel: [w1066] -> w532
      tunnel: w531 -> [w1066]
      tunnel: w525 -> [w1065]
      tunnel: [w1065] -> w524
      tunnel: w523 -> [w1064]
      tunnel: [w1063] -> w522
      tunnel: w521 -> [w1062]
      tunnel: [w1062] -> w518
      tunnel: w516 -> [w1061]
      tunnel: [w1033] -> w515
      tunnel: w500 -> [w1060]
      tunnel: [w1059] -> w499
      tunnel: w494 -> [w1058]
      tunnel: [w1058] -> w493
      tunnel: w487 -> [w1057]
      tunnel: [w1057] -> w486
      tunnel: w480 -> [w1056]
      tunnel: [w1056] -> w479
      tunnel: w471 -> [w1055]
      tunnel: [w1055] -> w470
      tunnel: w438 -> [w1054]
      tunnel: w435 -> [w1053]
      tunnel: w433 -> [w1052]
      tunnel: w431 -> [w1051]
      tunnel: w430 -> [w1050]
      tunnel: w428 -> [w1049]
      tunnel: w426 -> [w1036]
      tunnel: w424 -> [w1048]
      tunnel: w422 -> [w1047]
      tunnel: w419 -> [w1046]
      tunnel: w418 -> [w1074]
      tunnel: [w1045] -> w417
      tunnel: w413 -> [w1044]
      tunnel: w408 -> [w1043]
      tunnel: w403 -> [w1042]
      tunnel: [w1041] -> w402
      tunnel: w399 -> [w1014]
      tunnel: [w1027] -> w398
      tunnel: [w1040] -> w395
      tunnel: w388 -> [w1039]
      tunnel: w385 -> [w1038]
      tunnel: [w1037] -> w384
      tunnel: w377 -> [w1035]
      tunnel: [w1034] -> w376
      tunnel: w366 -> [w1012]
      tunnel: w365 -> [w1011]
      tunnel: [w1012] -> w364
      tunnel: [w1011] -> w363
      tunnel: [w1010] -> w358
      tunnel: w352 -> [w1009]
      tunnel: w576 -> [w2184]
      tunnel: w575 -> [w2244]
      tunnel: w567 -> [w2242]
      tunnel: w561 -> [w2241]
      tunnel: w559 -> [w2240]
      tunnel: w548 -> [w2202]
      tunnel: w547 -> [w2212]
      tunnel: w546 -> [w2213]
      tunnel: w540 -> [w2236]
      tunnel: w538 -> [w2235]
      tunnel: w532 -> [w2234]
      tunnel: w524 -> [w2233]
      tunnel: w522 -> [w2205]
      tunnel: w518 -> [w2227]
      tunnel: w515 -> [w2225]
      tunnel: [w2243] -> w511
      tunnel: [w2245] -> w510
      tunnel: [w2242] -> w509
      tunnel: [w2240] -> w508
      tunnel: [w2239] -> w507
      tunnel: [w2235] -> w506
      tunnel: [w2234] -> w505
      tunnel: [w2232] -> w504
      tunnel: [w2226] -> w503
      tunnel: w499 -> [w2224]
      tunnel: w493 -> [w2221]
      tunnel: [w2220] -> w492
      tunnel: w486 -> [w2219]
      tunnel: [w2218] -> w485
      tunnel: w479 -> [w2216]
      tunnel: [w2217] -> w477
      tunnel: w470 -> [w2215]
      tunnel: [w2214] -> w469
      tunnel: [w2184] -> w464
      tunnel: [w2205] -> w458
      tunnel: [w2202] -> w453
      tunnel: [w2213] -> w447
      tunnel: [w2212] -> w446
      tunnel: [w2211] -> w440
      tunnel: w417 -> [w2195]
      tunnel: [w2195] -> w416
      tunnel: w402 -> [w2203]
      tunnel: [w2203] -> w401
      tunnel: [w2202] -> w400
      tunnel: w398 -> [w2194]
      tunnel: [w2194] -> w397
      tunnel: w395 -> [w2193]
      tunnel: [w2193] -> w394
      tunnel: w384 -> [w2192]
      tunnel: [w2192] -> w383
      tunnel: w376 -> [w2191]
      tunnel: [w2191] -> w375
      tunnel: w364 -> [w2190]
      tunnel: w363 -> [w2189]
      tunnel: [w2190] -> w362
      tunnel: [w2189] -> w361
      tunnel: w358 -> [w2188]
      tunnel: [w2187] -> w357
      tunnel: [w2380] -> w517
      tunnel: [w2381] -> w501
      tunnel: [w2382] -> w530
      tunnel: [w2383] -> w537
      tunnel: [w2384] -> w551
      tunnel: [w2385] -> w556
      tunnel: [w2386] -> w566
      tunnel: [w2387] -> w574
      tunnel: [w2388] -> w580
      tunnel: w511 -> [w2388]
      tunnel: w510 -> [w2387]
      tunnel: w509 -> [w2386]
      tunnel: w508 -> [w2385]
      tunnel: w507 -> [w2384]
      tunnel: w506 -> [w2383]
      tunnel: w505 -> [w2382]
      tunnel: w504 -> [w2381]
      tunnel: w503 -> [w2380]
      tunnel: w492 -> [w2378]
      tunnel: [w2378] -> w491
      tunnel: w485 -> [w2377]
      tunnel: [w2377] -> w484
      tunnel: [w2376] -> w478
      tunnel: w477 -> [w2376]
      tunnel: w469 -> [w2375]
      tunnel: [w2375] -> w468
      tunnel: w464 -> [w2340]
      tunnel: [w2340] -> w463
      tunnel: w458 -> [w2334]
      tunnel: [w2334] -> w457
      tunnel: w453 -> [w2374]
      tunnel: [w2374] -> w452
      tunnel: [w2347] -> w415
      tunnel: w447 -> [w2347]
      tunnel: [w2370] -> w445
      tunnel: w446 -> [w2370]
      tunnel: w440 -> [w2328]
      tunnel: [w2328] -> w439
      tunnel: w416 -> [w2358]
      tunnel: [w2358] -> w414
      tunnel: [w2327] -> w407
      tunnel: w401 -> [w2346]
      tunnel: w400 -> [w2348]
      tunnel: w397 -> [w2323]
      tunnel: [w2323] -> w396
      tunnel: w394 -> [w2322]
      tunnel: [w2322] -> w393
      tunnel: w383 -> [w2321]
      tunnel: [w2321] -> w382
      tunnel: w375 -> [w2320]
      tunnel: [w2320] -> w374
      tunnel: w362 -> [w2318]
      tunnel: w361 -> [w2319]
      tunnel: [w2319] -> w360
      tunnel: [w2318] -> w359
      tunnel: w357 -> [w2317]
      tunnel: [w2317] -> w356
      frame #0 {
        w606 = 10178 items=["Finite Samples"=10178, "Continuous Samples"=10123, "Hardware Timed Single Point"=12522] ("sample mode")
        (unwired) 0.01 ("y")
        # "Turbo Read"
        # "Chiller Read"
        # "Gauge Read"
        # "Valve Read"
        # "Read Current Status"
        # "Primary Pump Read"
        n119 = call-poly <vilib>:"DAQmx Timing.vi"("task/channels in"=w608, "sample mode"=w606, "samples per channel"="samples per channel", "rate"="rate") -> ("task out"=w595:refnum<k21>, "error out"=w594:errorcluster)  [unwired: 10 in]
        n120 = call-poly <vilib>:"DAQmx Read.vi"("task/channels in"=w683) -> ("task out"=w673:refnum<k21>, "data"=w681:bool[], "error out"=w682:errorcluster)  [unwired: 12 in]
        n121 = call-poly <vilib>:"DAQmx Read.vi"("task/channels in"=w657) -> ("task out"=w656:refnum<k21>, "data"=w651:bool, "error out"=w654:errorcluster)  [unwired: 12 in]
        n122 = call-poly <vilib>:"DAQmx Read.vi"("task/channels in"=w687) -> ("task out"=w675:refnum<k21>, "data"=w671:bool, "error out"=w659:errorcluster)  [unwired: 12 in]
        n123 = case shown="False" w587 {
          tunnel: w593 -> [w690 w700]
          tunnel: w592 -> [w689 w699]
          tunnel: [w689 w693] -> w591
          tunnel: [w690 w692] -> w590
          tunnel: [0.0 ("Measurement") w691] -> w586
          frame False {
          }
          frame True {
            n124 = call "Backlight Command.vi"("error in (no error)"=w699, "ON/OFF"="ON/OFF", "VISA resource name"=w700) -> ("error out"=w696:errorcluster, "VISA resource name out"=w697:refnum<visa-resource-name>)  [unwired: 7 in]
            n125 = call "Read (Single Point).vi"("error in (no error)"=w696, "VISA resource name"=w697) -> ("error out"=w694:errorcluster, "Measurement"=w691:dbl, "VISA resource name out"=w692:refnum<visa-resource-name>)  [unwired: 7 in]
            "Measurement" <- w691
            n126 = call <vilib>:"Clear Errors.vi"("error in (no error)"=w694, "specific error code to clear (0: all)"=1073676294) -> ("error out"=w693:errorcluster)  [unwired: 4 in, 1 out]
          }
        }
        n127 = Build Array("Fake_Valve_Turbo_Read", "Fake_Valve_Bypass_Read", "Fake_Valve_Vent_Read", "Fake_Valve_Gate_Read") -> (w680:bool[])
        n128 = call-poly <vilib>:"DAQmx Read.vi"("task/channels in"=w595, "number of samples per channel"="samples per channel", "error in"=w594) -> ("task out"=w609:refnum<k21>, "data"=w612:waveform(dbl)[], "error out"=w610:errorcluster)  [unwired: 10 in]
        n129 = Index Array(array=w612, index=3) -> (element=w599:waveform(dbl))
        n130 = Index Array(array=w612, index=0) -> (element=w605:waveform(dbl))
        n131 = Index Array(array=w612, index=2) -> (element=w602:waveform(dbl))
        n132 = Index Array(array=w612, index=1) -> (element=w604:waveform(dbl))
        n133 = call-poly <vilib>:"Mean.vi"("X"=w599) -> ("mean"=→"Com Potential (V)":dbl)  [unwired: 1 out]
        n134 = call-poly <vilib>:"Mean.vi"("X"=w602) -> ("mean"=w601:dbl)  [unwired: 1 out]
        n135 = call-poly <vilib>:"Mean.vi"("X"=w605) -> ("mean"=w589:dbl)  [unwired: 1 out]
        n136 = Select(t=w586, s=w587, f=w589) -> (s? t:f=w588:dbl)
        n137 = call-poly <vilib>:"Mean.vi"("X"=w604) -> ("mean"=w603:dbl)  [unwired: 1 out]
        n138 = formula code="P_Conve_Torr = (10**V*1E-4);" "Convectron 2 Pressure calculation (Torr)"("V"=w601) -> ("P_Conve_Torr"=w663:dbl)
        n139 = formula code="P_Conve_Torr = (10**V*1E-4);" "Convectron 1 Pressure calculation (Torr)"("V"=w603) -> ("P_Conve_Torr"=w665:dbl)
        n140 = formula code="P_WRG_Torr = 10**(1.667*V-11.46);" "Ion gauge Pressure calculation (Torr)"("V"=w588) -> ("P_WRG_Torr"=w617:dbl)
        n141 = local read "Tubro_Control_Mode"() -> (w618:T1)
        n142 = local read "Use_real_Values?"() -> (w627:bool)
        n143 = case shown="\"HP700_Turbo_DSUB25_Control\", Default" w618 {
          tunnel: [w722 w747 w776] -> w648
          tunnel: [w715 w725 w750] -> w637
          tunnel: ["" ("response (data)") "" ("response (data)") w775] -> w645
          tunnel: w644 -> [w720 w745 w774]
          tunnel: [w720 w745 w773] -> w643
          tunnel: w642 -> [w723 w748 w772]
          tunnel: [w721 w746 w772] -> w641
          tunnel: w640 -> [w707 w732 w771]
          tunnel: [w718 w743 w771] -> w639
          tunnel: w610 -> [w706 w741 _]
          tunnel: "Fake Turbo Motor Read" -> [_ _ w770]
          tunnel: w627 -> [_ _ w769]
          tunnel: [w716 w740 w767] -> w626
          tunnel: [w709 w735 w751] -> w622
          tunnel: 4000.0 ("rate") -> [w703 w730 _]
          tunnel: 2000 ("samples per channel") -> [w701 w729 _]
          frame "HP700_Turbo_DSUB25_Control", Default {
            w702 = 10178 items=["Finite Samples"=10178, "Continuous Samples"=10123, "Hardware Timed Single Point"=12522] ("sample mode")
            # "Note this error in line\nfrom the other AI in \ntask must be attached\nto ensure they are read \nsequentially! Otherwise \nthis will throw an error"
            # "Convert 0-10V to 0-100% Turbo Speed"
            # "Turbo Speed Read"
            # "Turbo Error Read"
            n144 = call-poly <vilib>:"DAQmx Timing.vi"("task/channels in"=w707, "sample mode"=w702, "samples per channel"=w701, "rate"=w703, "error in"=w706) -> ("task out"=w704:refnum<k21>, "error out"=w705:errorcluster)  [unwired: 9 in]
            n145 = call-poly <vilib>:"DAQmx Read.vi"("task/channels in"=w704, "error in"=w705) -> ("task out"=w718:refnum<k21>, "data"=w711:waveform(dbl)[], "error out"=w717:errorcluster)  [unwired: 11 in]
            n146 = Index Array(array=w711, index=4) -> (element=w713:waveform(dbl))
            n147 = Unbundle By Name(w713) -> ("Y"=w712:dbl[])
            n148 = call-poly <vilib>:"Mean.vi"("X"=w712) -> ("mean"=w710:dbl)  [unwired: 1 out]
            n149 = call-poly <vilib>:"DAQmx Read.vi"("task/channels in"=w723, "error in"=w717) -> ("task out"=w721:refnum<k21>, "data"=w708:bool, "error out"=w722:errorcluster)  [unwired: 11 in]
            n150 = Multiply(x=w710, y=10.0) -> (x*y=w709:dbl)
            n151 = local read "Turbo_Motor_Sys_Cmd"() -> (w716:bool)
            n152 = Not(x=w708) -> (.not. x?=w715:bool)
          }
          frame "BigRed_Turbo_DSUB_15_Control" {
            w728 = 10178 items=["Finite Samples"=10178, "Continuous Samples"=10123, "Hardware Timed Single Point"=12522] ("sample mode")
            # "Note this error in line\nfrom the other AI in \ntask must be attached\nto ensure they are read \nsequentially! Otherwise \nthis will throw an error"
            # "Convert 0-10V to 0-100% Turbo Speed"
            # "Turbo Speed Read"
            # "Turbo Error Read"
            n153 = call-poly <vilib>:"DAQmx Timing.vi"("task/channels in"=w732, "sample mode"=w728, "samples per channel"=w729, "rate"=w730) -> ("task out"=w731:refnum<k21>)  [unwired: 10 in, 1 out]
            n154 = call-poly <vilib>:"DAQmx Read.vi"("task/channels in"=w731, "error in"=w741) -> ("task out"=w743:refnum<k21>, "data"=w734:waveform(dbl)[], "error out"=w742:errorcluster)  [unwired: 11 in]
            n155 = Index Array(array=w734, index=4) -> (element=w727:waveform(dbl))
            n156 = call-poly <vilib>:"Mean.vi"("X"=w727) -> ("mean"=w726:dbl)  [unwired: 1 out]
            n157 = call-poly <vilib>:"DAQmx Read.vi"("task/channels in"=w748, "error in"=w742) -> ("task out"=w746:refnum<k21>, "data"=w737:bool[], "error out"=w747:errorcluster)  [unwired: 11 in]
            n158 = Multiply(x=w726, y=10.0) -> (x*y=w735:dbl)
            n159 = local read "Turbo_Motor_Sys_Cmd"() -> (w740:bool)
            n160 = Index Array(array=w737, index=0) -> (element=w725:bool)
            n161 = Index Array(array=w737, index=1) -> (element=→"Still Spinning?":bool)
          }
          frame "HP700_Turbo_RS485_Control" {
            w789 = T6 {"Parameter"=2, "Parameter\nread only<->describe"=FALSE, "off<->on"=FALSE, "Rotation speed set value\nin rot. speed setting\noperations [%]"=nan, "Preset rotation Speed\nat Standby mode (%)"=nan, "maximum power\nsetpoint [%]"=0, "Gas mode"=1}  # Turbo_Motor_On?_Read
            w791 = u16 18 items=["nominal speed [Hz] (default) (315)", "intermediate circut current [A] (310)", "motor voltage [V] (313)", "actual power [W] (316)", "operating hours pump [h] (311)", "operating hours drive [h] (314)", "pump cycles (read only) (319)", "status oil sensor (read only) (301)", "speed switchpoint attained (read only) (302)", "overtemperature drive (read only) (304)", "overtemperature pump (read only) (305)", "target speed attained (read only) (306)", "pump accelerates (read only) (307) ", "controlled by remote (300)", "motor phase current [A] (317)", "acceleration / deceleration [rm/s] (336)", "hardware version controller (354)", "target speed (397)", "acutal speed (398)", "nominal speed (399)", "software version control unit (read only) (352)"] ("Parameter")
            # "Bottom Temp"
            # "Bearing Temp"
            # "Motor Temp"
            # "Ask for error code"
            # "Turbo Error Read"
            # "Convert To boolen"
            # "Turbo Motor Read"
            # "Turbo Speed Read"
            # "Convert rpm to Hz to %"
            n162 = local read "HP2300 RS485\nAddress"() -> (w759:u16)
            n163 = call "PV Operating adjustment turbopump.vi"("Operating adjustment - Cluster"=w789, "Adress of unit"=w759, "VISA session"=w774) -> ("error out"=w780:errorcluster, "response (data)"=w788:string, "dup VISA session"=w781:refnum<visa-resource-name>)  [unwired: 6 in]
            n164 = Equal?(x=w788, y="ON" ("Data")) -> (x = y?=w768:bool)
            n165 = call "PV General operating info.vi"("error in (no error)"=w780, "Parameter"=w791, "Adress of unit"=w759, "VISA session"=w781) -> ("error out"=w764:errorcluster, "response (data)"=w790:string, "dup VISA session"=w765:refnum<visa-resource-name>)  [unwired: 5 in]
            n166 = Decimal String To Number(string=w790) -> (number=w762:i32)  [unwired: 2 in, 1 out]
            n167 = Multiply(x=w762, y=0.016667) -> (x*y=w785:dbl)
            n168 = Divide(x=w785, y=820.0) -> (x/y=w783:dbl)
            n169 = Multiply(x=w783, y=100.0) -> (x*y=w751:dbl)
            n170 = call "PV Temperature info.vi"("VISA session"=w765, "Adress of unit"=w759, "Parameter"=T7."temperature motor [°C] (346)", "error in (no error)"=w764) -> ("dup VISA session"=w758:refnum<visa-resource-name>, "response (data)"=→"Turbo Motor Temp":string, "error out"=w755:errorcluster)  [unwired: 9 in]
            n171 = call "PV Temperature info.vi"("VISA session"=w758, "Adress of unit"=w759, "Parameter"=T7."temperature bearing [°C] (342)", "error in (no error)"=w755) -> ("dup VISA session"=w757:refnum<visa-resource-name>, "response (data)"=→"Turbo bearing Temp":string, "error out"=w754:errorcluster)  [unwired: 9 in]
            n172 = call "PV Temperature info.vi"("VISA session"=w757, "Adress of unit"=w759, "Parameter"=T7."temperature pump bottom [°C] (330)", "error in (no error)"=w754) -> ("dup VISA session"=w756:refnum<visa-resource-name>, "response (data)"=→"Turbo bottom Temp":string)  [unwired: 9 in, 1 out]
            n173 = call "PV Miscellaneous.vi"("PV Miscellaneous - Cluster"=T8 {"Parameter"=enum." Actual error code (read only)", "Parameter\nread only<->describe"=FALSE, "off<->on   "=FALSE, "Unit adress"=0, "Contens of service\nline; # of the 2nd\n parameter"=0}, "Adress of unit"=w759, "VISA session"=w756) -> ("error out"=w778:errorcluster, "response (data)"=w775:string, "dup VISA session"=w773:refnum<visa-resource-name>)  [unwired: 6 in]
            n174 = call <vilib>:"Simple Error Handler.vi"("error in (no error)"=w778) -> ("error?"=w750:bool, "error out"=w777:errorcluster)  [unwired: 4 in, 3 out]
            n175 = Merge Errors(w777) -> (w776:errorcluster)
            n176 = Select(t=w768, s=w769, f=w770) -> (s? t:f=w767:bool)
          }
        }
        "Numeric" <- w622
        n177 = Merge Errors(w654, w648) -> (w653:errorcluster)
        n178 = Number To Decimal String(number=w622, width (-)=i16 0) -> (decimal integer string=→"Turbo Speed":string)
        n179 = Merge Errors(w610, w653) -> (w655:errorcluster)
        n180 = Merge Errors(w659, w655) -> (w658:errorcluster)
        n181 = Select(t=w671, s=w627, f="Fake_Primary_Pump_Read") -> (s? t:f=w625:bool)
        n182 = Select(t=w651, s=w627, f="Fake_Chiller_Read") -> (s? t:f=w652:bool)
        n183 = Merge Errors(w686, w658) -> (w685:errorcluster)
        n184 = Select(t=w681, s=w627, f=w680) -> (s? t:f=w679:bool[])
        n185 = Select(t=w665, s=w627, f="Fake_Convec_1_Pressure_Torr") -> (s? t:f=w664:dbl)
        n186 = Select(t=w663, s=w627, f="Fake_Convec_2_Pressure_Torr") -> (s? t:f=w661:dbl)
        n187 = Select(t=w637, s=w627, f="Fake Turbo Error Read") -> (s? t:f=w638:bool)
        n188 = Select(t=w617, s=w627, f="Fake_WRG_Pressure_Torr") -> (s? t:f=w667:dbl)
        n189 = Select(t=w622, s=w627, f="Fake Turbo Speed Read (%)") -> (s? t:f=w646:dbl)
      }
      frame #1 {
        w793 = FALSE
        w825 = errorcluster {"status"=FALSE, "code"=5010, "source"="Conflict between Gate Valve command and read!"}  # Valve Gate Error
        w860 = 5.0  # Turbo Slow Speed  Threshold
        w859 = 95.0  # Turbo Speed Reached  Threshold
        w812 = errorcluster {"status"=FALSE, "code"=5004, "source"="Conflict between Chiller command and read!"}  # Chiller Error
        w810 = errorcluster {"status"=FALSE, "code"=0, "source"=""}  # No Error
        w881 = errorcluster {"status"=FALSE, "code"=5003, "source"="Conflict between Vent Valve command and read!"}  # Valve Vent Error
        w885 = errorcluster {"status"=FALSE, "code"=5002, "source"="Conflict between Bypass Valve command and read!"}  # Valve Bypass Error
        w826 = errorcluster {"status"=FALSE, "code"=0, "source"=""}  # No Error
        w889 = errorcluster {"status"=FALSE, "code"=5001, "source"="Conflict between turbo valve command and read!"}  # Valve Turbo Error
        w892 = errorcluster {"status"=FALSE, "code"=0, "source"=""}  # No Error
        w893 = errorcluster {"status"=FALSE, "code"=5000, "source"="Conflict between Primary pump command and read!"}  # Pump Error
        # "Ignore Turbo Error if chiller off"
        # "Check For Turbo Errors and Display Status"
        # "Check For Chiller Errors and Display Status"
        # "Display Gauge"
        # "Check For Primary Pump Errors and Display Status"
        # "Check For Valve Errors and Display Status"
        # "Check Status for error, and display status"
        n190 = local read "Chiller_Sys_Cmd"() -> (w817:bool)
        n191 = local write "Turbo Motor Read"(w838) -> ()
        n192 = Select(t=w816, s=w817, f=FALSE) -> (s? t:f=w818:bool)
        n193 = local read "Chiller_Sys_Cmd"() -> (w872:bool)
        n194 = local read "Primary_Sys_Cmd"() -> (w792:bool)
        n195 = local read "Valve_Gate_Sys_Cmd"() -> (w829:bool)
        n196 = local read "Valve_Bypass_Sys_Cmd"() -> (w884:bool)
        n197 = local read "Valve_Vent_Sys_Cmd"() -> (w883:bool)
        n198 = local read "Valve_Turbo_Sys_Cmd"() -> (w890:bool)
        n199 = Index Array(array=w831, index=1) -> (element=w836:bool)
        "Bypass Valve" <- w836
        n200 = Index Array(array=w831, index=3) -> (element=w824:bool)
        "Gate Valve" <- w824
        n201 = Index Array(array=w831, index=2) -> (element=w835:bool)
        "Vent Valve" <- w835
        n202 = Index Array(array=w831, index=0) -> (element=w837:bool)
        "Turbo Valve" <- w837
        n203 = Select(t=enum16{"Off", "On", "Error"}."On", s=w792, f=enum16{"Off", "On", "Error"}."Off") -> (s? t:f=w906:enum16{"Off", "On", "Error"})
        n204 = Greater?(x=w840, y=w859) -> (0:w863:bool)
        n205 = Select(t=enum16{"Off", "On", "Error"}."On", s=w841, f=enum16{"Off", "On", "Error"}."Off") -> (s? t:f=w871:enum16{"Off", "On", "Error"})
        n206 = Exclusive Or(1:w839, 2:w792) -> ()  [unwired: 1 out]
        n207 = Exclusive Or(1:w841, 2:w872) -> (0:w811:bool)
        n208 = local write "Vent Valve"(w835) -> ()
        n209 = local write "Bypass Valve"(w836) -> ()
        n210 = local write "Turbo Valve"(w837) -> ()
        n211 = Select(t=enum16{"Off", "On", "Error"}."Error", s=w793, f=w906) -> (s? t:f=w907:enum16{"Off", "On", "Error"})
        n212 = Select(t=enum16{"Off", "On", "Error"}."Error", s=w811, f=w871) -> (s? t:f=w870:enum16{"Off", "On", "Error"})
        n213 = local write "Gate Valve"(w824) -> ()
        n214 = Select(t=T10."Speed Reached", s=w863, f=T9."Spinning Up") -> (s? t:f=w803:u16)
        n215 = case shown="\"On\"" w870 {
          tunnel: [u32 12632256 ("Color") u32 6618880 ("Color") u32 16711680 ("Color")] -> w842
          tunnel: ["Chiller is Off" "Chiller is On" "Chiller error"] -> w856
          frame "Off", Default {
          }
          frame "On" {
          }
          frame "Error" {
          }
        }
        "Chiller Status" <- w856
        "Chiller Status 2" <- w842
        n216 = Greater?(x=w840, y=w860) -> (0:w864:bool)
        n217 = local read "Tubro_Control_Mode"() -> (w822:T1)
        n218 = case shown="\"BigRed_Turbo_DSUB_15_Control\"" w822 {
          tunnel: w855 -> [_ _ w935]
          tunnel: [FALSE FALSE w933] -> w851
          tunnel: w838 -> [_ _ w932]
          tunnel: [w911 w919 w925] -> w850
          tunnel: w818 -> [w908 w916 w924]
          frame "HP700_Turbo_DSUB25_Control", Default {
            w912 = errorcluster {"status"=FALSE, "code"=0, "source"=""}  # No Error
            n219 = Bundle By Name(cluster=w912, "status"=FALSE, "code"=5006, "source"="HP2300 Error. See Device LEDs for more info " ("string")) -> (w910:errorcluster)
            n220 = Select(t=w910, s=w908, f=w912) -> (s? t:f=w911:errorcluster)
          }
          frame "BigRed_Turbo_DSUB_15_Control" {
            w920 = errorcluster {"status"=FALSE, "code"=0, "source"=""}  # No Error
            n221 = Bundle By Name(cluster=w920, "status"=FALSE, "code"=5007, "source"="BRT Error. See Device LEDs for more info " ("string")) -> (w918:errorcluster)
            n222 = Select(t=w918, s=w916, f=w920) -> (s? t:f=w919:errorcluster)
          }
          frame "HP700_Turbo_RS485_Control" {
            w929 = errorcluster {"status"=FALSE, "code"=0, "source"=""}  # No Error
            w928 = errorcluster {"status"=TRUE, "code"=5005, "source"="Conflict between Turbo Motor command and read!"}  # Turbo Motor Conflict Error
            n223 = local read "Turbo_Motor_Sys_Cmd"() -> (w931:bool)
            n224 = Exclusive Or(1:w931, 2:w932) -> (0:w933:bool)
            n225 = Concatenate Strings("HP2300 Error Code: " ("string"), w935) -> (w934:string)
            n226 = Bundle By Name(cluster=w928, "status"=FALSE, "code"=5006, "source"=w934) -> (w930:errorcluster)
            n227 = Select(t=w928, s=w933, f=w929) -> (s? t:f=w927:errorcluster)
            n228 = Select(t=w930, s=w924, f=w929) -> (s? t:f=w926:errorcluster)
            n229 = Merge Errors(w927, w926) -> (w925:errorcluster)
          }
        }
        n230 = Select(t=T10."Turbo In Standby", s=w801, f=w803) -> (s? t:f=w802:u16)
        n231 = Select(t=w812, s=w811, f=w810) -> (s? t:f=w813:errorcluster)
        n232 = Exclusive Or(1:w829, 2:w824) -> (0:w806:bool)
        "Gate Valve Error?" <- w806
        n233 = Exclusive Or(1:w884, 2:w836) -> (0:w808:bool)
        "Bypass Valve Error?" <- w808
        n234 = Select(t=T9."Spinning Down", s=w864, f=T9."Off") -> (s? t:f=w865:T9)
        n235 = Exclusive Or(1:w883, 2:w835) -> (0:w807:bool)
        "Vent Valve Error?" <- w807
        n236 = Exclusive Or(1:w890, 2:w837) -> (0:w809:bool)
        "Turbo Valve Error?" <- w809
        n237 = case shown="\"Off\", Default" w907 {
          tunnel: [u32 12632256 ("Color") u32 6618880 ("Color") u32 16711680 ("Color")] -> w905
          tunnel: ["is Off" "is On" "Error"] -> w879
          frame "Off", Default {
          }
          frame "On" {
          }
          frame "Error" {
          }
        }
        "Primary Status" <- w905
        n238 = Select(t=w802, s=w838, f=w865) -> (s? t:f=w866:u16)
        n239 = Select(t=w889, s=w809, f=w826) -> (s? t:f=w888:errorcluster)
        n240 = Select(t=T10."Error", s=w818, f=w866) -> (s? t:f=w862:u16)
        n241 = Or(x=w818, y=w851) -> ()  [unwired: 1 out]
        n242 = case shown="4" w862 {
          tunnel: [u32 12632256 ("Color") u32 3381759 ("Color") u32 6618880 ("Color") u32 10650795 ("Color") u32 16757266 ("Color") u32 16711680 ("Color")] -> w861
          tunnel: ["Turbo Off" "Turbo Spinning Up" "Turbo Speed Reached" "Turbo Spinning Down" "Turbo In Standby" "Turbo Error"] -> w833
          frame 0, Default {
          }
          frame 1 {
          }
          frame 2 {
          }
          frame 3 {
          }
          frame 4 {
          }
          frame 5 {
          }
        }
        "Turbo Status Color" <- w861
        "Turbo Status" <- w833
        n243 = Select(t=w825, s=w806, f=w826) -> (s? t:f=w827:errorcluster)
        n244 = Select(t=w881, s=w807, f=w826) -> (s? t:f=w882:errorcluster)
        n245 = Select(t=w885, s=w808, f=w826) -> (s? t:f=w886:errorcluster)
        n246 = Select(t=w893, s=w793, f=w892) -> (s? t:f=w868:errorcluster)
        n247 = Concatenate Strings("Primary Pump " ("string"), w879) -> (→"Primary Pump Status":string)
        n248 = Merge Errors(w850) -> (w857:errorcluster)
        n249 = Merge Errors(w813, w857) -> (w794:errorcluster)
        n250 = Merge Errors(w868, w794) -> (w828:errorcluster)
        n251 = Merge Errors(w888, w886, w882, w827, w828) -> (w887:errorcluster)
        n252 = Merge Errors(w900, w887) -> (w901:errorcluster)
        "error out" <- w900
        "Wide Range Gauge Pressure (Torr)" <- w795
        "Foreline Convectron" <- w834
        "Primary_Pump_Read" <- w839
        "Turbo Motor Read" <- w838
        "Turbo Convectron" <- w821
      }
      frame #2 {
        # "Clear Errors?"
        # "Poll User Turbo Commands"
        # "Poll User Chiller Commands"
        # "Poll User Primary Pump Commands"
        # "Poll User Valve Commands"
        n253 = case shown="False" "Clear error?" {
          tunnel: [w1005 w1006] -> w972
          tunnel: w973 -> [w1005 _]
          frame False {
          }
          frame True {
            n254 = call <vilib>:"Clear Errors.vi"() -> ("error out"=w1006:errorcluster)  [unwired: 6 in, 1 out]
          }
        }
        n255 = Wait (ms)(milliseconds to wait=u32 10) -> ()  [unwired: 1 out]
      }
      frame #3 {
        # "Turbo Standby"
        # "Turbo Standby\ncmd"
        # "Gate Valve\nRead"
        # "Turbo Motor\nRead"
        # "Turbo Speed\n(%)"
        # "Turbo Motor\nCmd"
        # "Turbo Error\nAckn Cmd"
        # "Chiller \nCmd"
        # "Chiller \nRead"
        # "Foreline\nConvectron\n(Torr)"
        # "Turbo\nConvectron\n(Torr)"
        # "WRG Pressure (Torr)"
        # "Primary Pump\nCmd"
        # "Primary Pump\nRead"
        # "Vent Valve\nCmd"
        # "Bypass Valve\nCmd"
        # "Turbo_Valve\nCmd"
        # "Vent Valve\nRead"
        # "Bypass Valve\nRead"
        # "Turbo_Valve\nRead"
        # "Asses User Demands"
        n256 = Select(t=Facility_State."Admin", s="change_to_admin_mode", f=w1014) -> (s? t:f=w1015:T4)
        n257 = case shown="\"Auto\"" w1015 {
          selector: w1015 -> [w1100 w1431 _ w1684]
          tunnel: [w1098 w1440 FALSE ("Primary_User_Cmd") w1667] -> w1077
          tunnel: w1079 -> [w1114 w1454 _ w1675]
          tunnel: w1078 -> [w1108 w1444 _ w1645]
          tunnel: [w1108 w1444 errorcluster {"status"=FALSE, "code"=0, "source"=""} ("error out") w1645] -> w1076
          tunnel: w1075 -> [w1121 w1456 _ w1680]
          tunnel: w1074 -> [w1119 w1455 _ w1679]
          tunnel: w1073 -> [w1117 w1452 _ w1678]
          tunnel: [w1099 w1443 FALSE ("Valve_Turbo_User_Cmd") w1671] -> w1032
          tunnel: [w1080 w1442 FALSE ("Valve_Bypass_User_Cmd") w1670] -> w1072
          tunnel: [w1092 w1441 FALSE ("Valve_Vent_User_Cmd") w1669] -> w1031
          tunnel: w1064 -> [w1112 w1451 _ w1673]
          tunnel: [w1111 w1439 FALSE ("Chiller_User_Cmd") w1666] -> w1063
          tunnel: w1061 -> [w1109 w1445 _ w1664]
          tunnel: [w1097 w1438 FALSE ("Turbo_Motor_User_Cmd") w1653] -> w1033
          tunnel: w1060 -> [w1122 w1437 _ _]
          tunnel: [w1122 w1437 FALSE ("Turbo_Error_Acknowlege_Cmd") FALSE ("Turbo_Error_Acknowlege_Cmd")] -> w1059
          tunnel: w1054 -> [_ w1447 _ w1632]
          tunnel: w1053 -> [_ w1449 _ w1683]
          tunnel: w1052 -> [_ w1450 _ w1682]
          tunnel: w1051 -> [_ w1448 _ w1676]
          tunnel: w1050 -> [_ _ _ w1661]
          tunnel: w1049 -> [_ w1436 _ w1662]
          tunnel: w1048 -> [_ w1446 _ w1674]
          tunnel: w1047 -> [w1096 w1453 _ w1665]
          tunnel: w1046 -> [_ w1435 _ w1672]
          tunnel: [TRUE ("Visible") FALSE ("Visible") FALSE ("Visible") FALSE ("Visible")] -> w1008
          tunnel: [w1093 FALSE ("T button?") FALSE ("T button?") w1668] -> w1045
          tunnel: w1044 -> [w1105 _ _ w1677]
          tunnel: w1043 -> [_ _ _ w1681]
          tunnel: w1042 -> [w1104 w1432 w1620 w1647]
          tunnel: [w1104 w1432 w1620 w1636] -> w1041
          tunnel: [w1082 w1431 w1619 w1684] -> w1027
          tunnel: [w1085 Current_Facility_State."Pumping to Rough" Current_Facility_State."Facility Off" w1659] -> w1040
          tunnel: w1039 -> [_ _ _ w1652]
          tunnel: w1038 -> [_ _ _ w1650]
          tunnel: [w1087 Current_Facility_State."Pumping to Rough" ("Facility Target State") Current_Facility_State."Facility Off" ("Facility Target State") w1658] -> w1037
          tunnel: w1036 -> [_ w1428 _ w1660]
          tunnel: w1035 -> [_ _ _ w1657]
          tunnel: [w1090 0 ("f") 0 ("f") w1656] -> w1034
          tunnel: [w1103 FALSE ("Turbo_Error_Acknowlege_Cmd") FALSE w1635] -> w1010
          tunnel: w1009 -> [w1102 _ _ w1634]
          frame "Admin" {
            # "Turbo on?"
            # "go right into substate 2, if and only if you are going\n to primary pump down and bypass is open"
            # "Bypass"
            # "Turbo Valve"
            # "Vent"
            # "Gate"
            # "Enable Switches?"
            # "Read User Commands"
            n258 = Greater?(x=w1096, y=15.0) -> (0:w1094:bool)
            n259 = case shown="True" "Turbo_Motor_User_Cmd" {
              tunnel: [w1323 w1327] -> w1097
              tunnel: w1109 -> [w1323 w1326]
              tunnel: [w1322 w1325] -> w1103
              tunnel: w1102 -> [w1322 w1324]
              frame False {
              }
              frame True {
                n260 = case shown="False" w1326 {
                  tunnel: [w1332 w1335] -> w1327
                  tunnel: [FALSE w1334] -> w1325
                  tunnel: w1324 -> [_ w1333]
                  frame False {
                    n261 = Two Button Dialog(message="Start Turbo Pump?", 1:"No" ("F button name (\"Cancel\")"), 2:"Yes" ("T button name (\"OK\")")) -> (T button?=w1332:bool)
                  }
                  frame True {
                    n262 = case shown="True" w1333 {
                      tunnel: [w1337 w1352] -> w1335
                      tunnel: [w1336 w1351] -> w1334
                      frame False {
                        n263 = call <vilib>:"Three Button Dialog.vi"("Right Button Text (\"Cancel\")"=" Activate Standby" ("Right Button Text (\"Cancel\")"), "Center Button Text (\"No\")"="No" ("Center Button Text (\"No\")"), "Left Button Text (\"Yes\")"="Yes" ("Left Button Text (\"Yes\")"), "message"="Stop Turbo Pump?") -> ("Which Button?"=w1338:T11)  [unwired: 7 in]
                        n264 = case shown="\"Window Close\"" w1338 {
                          tunnel: [FALSE TRUE TRUE TRUE] -> w1337
                          tunnel: [FALSE FALSE TRUE FALSE] -> w1336
                          frame "Left Button" {
                          }
                          frame "Center Button", Default {
                          }
                          frame "Right Button" {
                          }
                          frame "Window Close" {
                          }
                        }
                      }
                      frame True {
                        n265 = call <vilib>:"Three Button Dialog.vi"("Right Button Text (\"Cancel\")"=" Yes, Spin Down" ("Right Button Text (\"Cancel\")"), "Center Button Text (\"No\")"="No" ("Center Button Text (\"No\")"), "Left Button Text (\"Yes\")"="Yes, Spin Up" ("Left Button Text (\"Yes\")"), "message"=" Exit Turbo Standby Mode?") -> ("Which Button?"=w1353:T11)  [unwired: 7 in]
                        n266 = case shown="\"Window Close\"" w1353 {
                          tunnel: [TRUE TRUE FALSE TRUE] -> w1352
                          tunnel: [FALSE TRUE FALSE TRUE] -> w1351
                          frame "Left Button" {
                          }
                          frame "Center Button", Default {
                          }
                          frame "Right Button" {
                          }
                          frame "Window Close" {
                          }
                        }
                      }
                    }
                  }
                }
              }
            }
            n267 = case shown="True" "Valve_Bypass_User_Cmd" {
              tunnel: [w1402 w1404] -> w1080
              tunnel: w1119 -> [w1402 w1403]
              frame False {
              }
              frame True {
                n268 = case shown="False" w1403 {
                  tunnel: [w1408 w1409] -> w1404
                  frame False {
                    n269 = Two Button Dialog(message="Open Bypass Valve?", 1:"No" ("F button name (\"Cancel\")"), 2:"Yes" ("T button name (\"OK\")")) -> (T button?=w1408:bool)
                  }
                  frame True {
                    n270 = Two Button Dialog(message="Close Bypass Valve?", 1:"No" ("F button name (\"Cancel\")"), 2:"Yes" ("T button name (\"OK\")")) -> (T button?=w1410:bool)
                    n271 = Not(x=w1410) -> (.not. x?=w1409:bool)
                  }
                }
              }
            }
            n272 = case shown="True" "Valve_Vent_User_Cmd" {
              tunnel: [w1390 w1392] -> w1092
              tunnel: w1117 -> [w1390 w1391]
              frame False {
              }
              frame True {
                n273 = case shown="False" w1391 {
                  tunnel: [w1396 w1397] -> w1392
                  frame False {
                    n274 = Two Button Dialog(message="Open Vent Valve?", 1:"No" ("F button name (\"Cancel\")"), 2:"Yes" ("T button name (\"OK\")")) -> (T button?=w1396:bool)
                  }
                  frame True {
                    n275 = Two Button Dialog(message="Close Vent Valve?", 1:"No" ("F button name (\"Cancel\")"), 2:"Yes" ("T button name (\"OK\")")) -> (T button?=w1398:bool)
                    n276 = Not(x=w1398) -> (.not. x?=w1397:bool)
                  }
                }
              }
            }
            n277 = case shown="True" "Valve_Gate_User_Cmd" {
              tunnel: [w1310 w1312] -> w1093
              tunnel: w1105 -> [w1310 w1311]
              frame False {
              }
              frame True {
                n278 = case shown="True" w1311 {
                  tunnel: [w1316 w1317] -> w1312
                  frame False {
                    n279 = Two Button Dialog(message="Open Gate Valve?", 1:"No" ("F button name (\"Cancel\")"), 2:"Yes" ("T button name (\"OK\")")) -> (T button?=w1316:bool)
                  }
                  frame True {
                    n280 = Two Button Dialog(message="Close Gate Valve?", 1:"No" ("F button name (\"Cancel\")"), 2:"Yes" ("T button name (\"OK\")")) -> (T button?=w1318:bool)
                    n281 = Not(x=w1318) -> (.not. x?=w1317:bool)
                  }
                }
              }
            }
            n282 = case shown="True" "Valve_Turbo_User_Cmd" {
              tunnel: [w1414 w1416] -> w1099
              tunnel: w1121 -> [w1414 w1415]
              frame False {
              }
              frame True {
                n283 = case shown="False" w1415 {
                  tunnel: [w1420 w1421] -> w1416
                  frame False {
                    n284 = Two Button Dialog(message="Open Turbo Valve?", 1:"No" ("F button name (\"Cancel\")"), 2:"Yes" ("T button name (\"OK\")")) -> (T button?=w1420:bool)
                  }
                  frame True {
                    n285 = Two Button Dialog(message="Close Turbo Valve?", 1:"No" ("F button name (\"Cancel\")"), 2:"Yes" ("T button name (\"OK\")")) -> (T button?=w1422:bool)
                    n286 = Not(x=w1422) -> (.not. x?=w1421:bool)
                  }
                }
              }
            }
            n287 = case shown="True" "Primary_User_Cmd" {
              tunnel: [w1378 w1380] -> w1098
              tunnel: w1114 -> [w1378 w1379]
              frame False {
              }
              frame True {
                n288 = case shown="True" w1379 {
                  tunnel: [w1384 w1385] -> w1380
                  frame False {
                    n289 = Two Button Dialog(message="Turn on Primary Pump?", 1:"No" ("F button name (\"Cancel\")"), 2:"Yes" ("T button name (\"OK\")")) -> (T button?=w1384:bool)
                  }
                  frame True {
                    n290 = Two Button Dialog(message="Turn Off Primary Pump?", 1:"No" ("F button name (\"Cancel\")"), 2:"Yes" ("T button name (\"OK\")")) -> (T button?=w1386:bool)
                    n291 = Not(x=w1386) -> (.not. x?=w1385:bool)
                  }
                }
              }
            }
            n292 = case shown="True" "Chiller_User_Cmd" {
              tunnel: [w1366 w1368] -> w1111
              tunnel: w1112 -> [w1366 w1367]
              frame False {
              }
              frame True {
                n293 = case shown="True" w1367 {
                  tunnel: [w1372 w1373] -> w1368
                  frame False {
                    n294 = Two Button Dialog(message="Turn on Chiller?", 1:"No" ("F button name (\"Cancel\")"), 2:"Yes" ("T button name (\"OK\")")) -> (T button?=w1372:bool)
                  }
                  frame True {
                    n295 = Two Button Dialog(message="Turn Off Chiller?", 1:"No" ("F button name (\"Cancel\")"), 2:"Yes" ("T button name (\"OK\")")) -> (T button?=w1374:bool)
                    n296 = Not(x=w1374) -> (.not. x?=w1373:bool)
                  }
                }
              }
            }
            n297 = case shown="True" "Change to Auto" {
              tunnel: w1098 -> [_ w1145]
              tunnel: w1100 -> [w1125 _]
              tunnel: [w1125 w1134] -> w1082
              tunnel: [Current_Facility_State."Facility Off" w1136] -> w1085
              tunnel: [Current_Facility_State."Facility Off" w1138] -> w1087
              tunnel: w1097 -> [_ w1144]
              tunnel: w1094 -> [_ w1143]
              tunnel: w1099 -> [_ w1142]
              tunnel: w1093 -> [_ w1141]
              tunnel: w1092 -> [_ w1140]
              tunnel: w1080 -> [_ w1128]
              frame False {
                (unwired) FALSE ("Keep Primary On While venting?")
              }
              frame True {
                # "Ask to Switch?"
                # "Primary on?"
                n298 = case shown="True" w1145 {
                  tunnel: w1144 -> [w1186 w1208]
                  tunnel: w1143 -> [_ _]
                  tunnel: [w1199 w1215] -> w1137
                  tunnel: [w1198 w1214] -> w1127
                  tunnel: [w1197 w1213] -> w1139
                  tunnel: w1142 -> [w1196 w1210]
                  tunnel: w1141 -> [w1194 w1216]
                  tunnel: w1140 -> [w1193 w1212]
                  tunnel: [w1195 w1211] -> w1129
                  tunnel: w1128 -> [w1192 w1209]
                  frame False {
                    # "Must be facility off, lets check"
                    n299 = Not(x=w1196) -> (.not. x?=w1191:bool)
                    n300 = Not(x=w1193) -> (.not. x?=w1189:bool)
                    n301 = Not(x=w1194) -> (.not. x?=w1190:bool)
                    n302 = Not(x=w1192) -> (.not. x?=w1188:bool)
                    n303 = Not(x=w1186) -> (.not. x?=w1185:bool)
                    n304 = Compound Arithmetic op=AND(w1185, w1191, w1190, w1189, w1188) -> (w1187:bool)
                    n305 = case shown="True" w1187 {
                      tunnel: [Current_Facility_State."Facility Off" Current_Facility_State."Facility Off"] -> w1199
                      tunnel: [Current_Facility_State."Facility Off" Current_Facility_State."Facility Off"] -> w1198
                      tunnel: ["" "Facility off"] -> w1197
                      tunnel: [FALSE TRUE] -> w1195
                      frame False {
                      }
                      frame True {
                      }
                    }
                  }
                  frame True {
                    # "Gate open?"
                    n306 = case shown="False" w1216 {
                      selector: w1216 -> [w1220 w1295]
                      tunnel: [w1225 w1301] -> w1215
                      tunnel: [w1224 w1300] -> w1214
                      tunnel: [w1223 w1299] -> w1213
                      tunnel: w1212 -> [w1217 w1294]
                      tunnel: [w1222 w1298] -> w1211
                      tunnel: w1210 -> [w1221 w1296]
                      tunnel: w1209 -> [w1219 w1292]
                      tunnel: w1208 -> [w1218 _]
                      frame False {
                        # "Turbo On?"
                        n307 = case shown="False" w1218 {
                          selector: w1218 -> [w1229 _]
                          tunnel: [w1236 w1252] -> w1225
                          tunnel: [w1235 w1251] -> w1224
                          tunnel: [w1234 w1250] -> w1223
                          tunnel: [w1233 w1249] -> w1222
                          tunnel: w1221 -> [w1227 w1247]
                          tunnel: w1220 -> [w1231 w1246]
                          tunnel: w1219 -> [_ w1248]
                          tunnel: w1217 -> [_ w1245]
                          frame False {
                            # "Must be Pumping to rough,\nlets check:"
                            n308 = Not(x=w1229) -> (.not. x?=w1228:bool)
                            n309 = Not(x=w1231) -> (.not. x?=w1230:bool)
                            n310 = Not(x=w1227) -> (.not. x?=w1226:bool)
                            n311 = Compound Arithmetic op=AND(w1226, w1230, w1228) -> (w1232:bool)
                            n312 = case shown="True" w1232 {
                              tunnel: [Current_Facility_State."Facility Off" Current_Facility_State."Pumping to Rough"] -> w1236
                              tunnel: [Current_Facility_State."Facility Off" Current_Facility_State."Pumping to High Vac"] -> w1235
                              tunnel: ["" "Pumping to Rough"] -> w1234
                              tunnel: [FALSE ("Keep Primary On While venting?") TRUE ("Keep Primary On While venting?")] -> w1233
                              frame False {
                              }
                              frame True {
                                # "If bypass open, skip warm up"
                              }
                            }
                          }
                          frame True {
                            # "Is the bypass open?"
                            n313 = case shown="True" w1248 {
                              selector: w1248 -> [w1255 w1273]
                              tunnel: [w1262 w1282] -> w1252
                              tunnel: [w1261 w1281] -> w1251
                              tunnel: [w1260 w1280] -> w1250
                              tunnel: [w1259 w1279] -> w1249
                              tunnel: w1247 -> [w1258 w1272]
                              tunnel: w1246 -> [w1257 w1277]
                              tunnel: w1245 -> [_ w1275]
                              frame False {
                                # "Must be venting, Lets Check:"
                                n314 = Not(x=w1257) -> (.not. x?=w1254:bool)
                                n315 = Not(x=w1255) -> (.not. x?=w1253:bool)
                                n316 = Compound Arithmetic op=AND(w1258, w1254, w1253) -> (w1256:bool)
                                n317 = case shown="True" w1256 {
                                tunnel: [Current_Facility_State."Facility Off" Current_Facility_State."Venting"] -> w1262
                                tunnel: [Current_Facility_State."Facility Off" Current_Facility_State."Venting"] -> w1261
                                tunnel: ["0" "Venting"] -> w1260
                                tunnel: [FALSE ("Keep Primary On While venting?") TRUE ("Keep Primary On While venting?")] -> w1259
                                frame False {
                                }
                                frame True {
                                }
                                }
                              }
                              frame True {
                                # "Must be pumping to Rough,\n Lets check:"
                                n318 = Not(x=w1277) -> (.not. x?=w1276:bool)
                                n319 = Not(x=w1272) -> (.not. x?=w1271:bool)
                                n320 = Not(x=w1275) -> (.not. x?=w1274:bool)
                                n321 = Compound Arithmetic op=AND(w1271, w1276, w1274, w1273) -> (w1278:bool)
                                n322 = case shown="False" w1278 {
                                tunnel: [Current_Facility_State."Facility Off" Current_Facility_State."Pumping to Rough"] -> w1282
                                tunnel: [Current_Facility_State."Facility Off" Current_Facility_State."Pumping to High Vac"] -> w1281
                                tunnel: ["" "Pumping to Rough"] -> w1280
                                tunnel: [FALSE ("Keep Primary On While venting?") TRUE ("Keep Primary On While venting?")] -> w1279
                                frame False {
                                }
                                frame True {
                                }
                                }
                              }
                            }
                          }
                        }
                      }
                      frame True {
                        # "Must be Hi Vac, lets check:"
                        n323 = Not(x=w1294) -> (.not. x?=w1293:bool)
                        n324 = Not(x=w1292) -> (.not. x?=w1291:bool)
                        n325 = Compound Arithmetic op=AND(w1296, w1295, w1293, w1291) -> (w1297:bool)
                        n326 = case shown="False" w1297 {
                          tunnel: [Current_Facility_State."Facility Off" Current_Facility_State."Pumping to High Vac"] -> w1301
                          tunnel: [Current_Facility_State."Facility Off" Current_Facility_State."Pumping to High Vac"] -> w1300
                          tunnel: ["" "Pumping to High Vac"] -> w1299
                          tunnel: [FALSE ("Keep Primary On While venting?") TRUE ("Keep Primary On While venting?")] -> w1298
                          frame False {
                          }
                          frame True {
                          }
                        }
                      }
                    }
                  }
                }
                n327 = case shown="True" w1129 {
                  tunnel: w1139 -> [_ w1150]
                  tunnel: [Current_Facility_State."Facility Off" ("f") Current_Facility_State."Facility Off" ("f")] -> w1131
                  tunnel: [FALSE ("T button?") w1155] -> w1130
                  tunnel: w1127 -> [w1146 w1152]
                  tunnel: [w1146 w1151] -> w1126
                  frame False {
                    n328 = call "Display Message to User"("Message"="Target State Not Recognised! " ("string")) -> ()  [unwired: 9 in, 2 out]
                  }
                  frame True {
                    n329 = Equal?(x=w1150, y="Pumping to Rough") -> (x = y?=w1153:bool)
                    n330 = case shown="True" w1153 {
                      tunnel: [w1159 w1168] -> w1155
                      tunnel: w1152 -> [w1158 _]
                      tunnel: [w1158 w1169] -> w1151
                      tunnel: w1150 -> [w1157 w1175]
                      frame False {
                        n331 = Concatenate Strings("Go to State: " ("string"), "\r", "\"" ("string"), w1157, "\"?" ("string")) -> (w1166:string)
                        n332 = Two Button Dialog(message=w1166, 1:"No" ("F button name (\"Cancel\")"), 2:"Yes" ("T button name (\"OK\")")) -> (T button?=w1159:bool)
                      }
                      frame True {
                        n333 = Concatenate Strings("Go to State: " ("string"), "\r", "\"" ("string"), w1175, "\"?" ("string")) -> (w1174:string)
                        n334 = call <vilib>:"Three Button Dialog.vi"("Right Button Text (\"Cancel\")"="No" ("Right Button Text (\"Cancel\")"), "Center Button Text (\"No\")"="Yes, Target Low Vac" ("Center Button Text (\"No\")"), "Left Button Text (\"Yes\")"="Yes, Target High Vac" ("Left Button Text (\"Yes\")"), "message"=w1174) -> ("Which Button?"=w1173:T11)  [unwired: 7 in]
                        n335 = case shown="\"Right Button\"" w1173 {
                          tunnel: [Current_Facility_State."Pumping to High Vac" Current_Facility_State."Pumping to Rough" Current_Facility_State."Facility Off"] -> w1169
                          tunnel: [TRUE ("T button?") TRUE ("T button?") FALSE ("T button?")] -> w1168
                          frame "Left Button", Default {
                          }
                          frame "Center Button" {
                          }
                          frame "Right Button" {
                          }
                        }
                      }
                    }
                  }
                }
                n336 = Select(t=w1137, s=w1130, f=Current_Facility_State."Facility Off") -> (s? t:f=w1136:T2)
                n337 = Select(t=w1126, s=w1130, f=w1131) -> (s? t:f=w1138:T2)
                n338 = Select(t=Facility_State."Auto", s=w1130, f=Facility_State."Admin") -> (s? t:f=w1134:T4)
              }
            }
            n339 = Equal?(x=w1085, y=Current_Facility_State."Pumping to Rough") -> (x = y?=w1084:bool)
            n340 = Equal?(x=w1082, y=Facility_State."Auto") -> (x = y?=w1083:bool)
            n341 = Compound Arithmetic op=AND(w1083, w1084, w1080) -> (w1088:bool)
            n342 = Select(t=2, s=w1088, f=0) -> (s? t:f=w1090:i32)
          }
          frame "Manual" {
            # "Enable Switches?"
            # "Turn On Turbo Motor?"
            # "Turn On Chiller?"
            # "Open Vent Valve?"
            # "Turn on Primary Pump?"
            # "Open Bypass Valve?"
            # "Open Turbo Valve?"
            n343 = case shown="True" w1452 {
              tunnel: [FALSE w1524] -> w1441
              tunnel: w1449 -> [_ w1523]
              tunnel: w1447 -> [_ w1521]
              tunnel: w1453 -> [_ w1519]
              tunnel: w1448 -> [_ w1522]
              tunnel: w1435 -> [_ w1520]
              frame False {
              }
              frame True {
                # "Primary Pump On?"
                n344 = case shown="False" w1522 {
                  tunnel: [w1528 FALSE] -> w1524
                  tunnel: w1523 -> [w1529 _]
                  tunnel: w1521 -> [w1527 _]
                  tunnel: w1520 -> [w1526 _]
                  tunnel: w1519 -> [w1525 _]
                  frame False {
                    # "Bypass Valve Open?"
                    n345 = case shown="False" w1529 {
                      tunnel: [w1532 FALSE] -> w1528
                      tunnel: w1527 -> [w1533 _]
                      tunnel: w1526 -> [w1531 _]
                      tunnel: w1525 -> [w1530 _]
                      frame False {
                        # "Turbo Valve Open?"
                        n346 = case shown="False" w1533 {
                          tunnel: [w1535 FALSE] -> w1532
                          tunnel: w1531 -> [w1536 _]
                          tunnel: w1530 -> [w1534 _]
                          frame False {
                            # "Turbo Motor On?"
                            n347 = case shown="False" w1536 {
                              tunnel: [w1537 FALSE] -> w1535
                              tunnel: w1534 -> [w1539 _]
                              frame False {
                                # "Turbo Still Spinning?"
                                n348 = Greater?(x=w1539, y=5.0) -> (0:w1538:bool)
                                n349 = case shown="False" w1538 {
                                tunnel: [TRUE FALSE] -> w1537
                                frame False {
                                # "Ok, open vent valve"
                                }
                                frame True {
                                n350 = One Button Dialog(message="Please wait for Turbo to slow down first") -> ()  [unwired: 1 in, 1 out]
                                }
                                }
                              }
                              frame True {
                                n351 = One Button Dialog(message="Please Turn Turbo off First") -> ()  [unwired: 1 in, 1 out]
                              }
                            }
                          }
                          frame True {
                            n352 = One Button Dialog(message="Please Close Turbo Valve First") -> ()  [unwired: 1 in, 1 out]
                          }
                        }
                      }
                      frame True {
                        n353 = One Button Dialog(message="Please Close Bypass Valve first") -> ()  [unwired: 1 in, 1 out]
                      }
                    }
                  }
                  frame True {
                    n354 = One Button Dialog(message="Please Stop Primary Pump First") -> ()  [unwired: 1 in, 1 out]
                  }
                }
              }
            }
            n355 = case shown="True" w1456 {
              tunnel: w1450 -> [_ w1602]
              tunnel: [w1589 w1601] -> w1443
              tunnel: w1449 -> [_ w1600]
              tunnel: w1435 -> [w1590 _]
              tunnel: w1453 -> [w1588 _]
              frame False {
                # "Turbo Motor On?"
                n356 = case shown="False" w1590 {
                  tunnel: [w1592 TRUE] -> w1589
                  tunnel: w1588 -> [w1591 _]
                  frame False {
                    # "Turbo Still Spinning?"
                    n357 = Greater?(x=w1591, y=5.0) -> (0:w1594:bool)
                    n358 = case shown="False" w1594 {
                      tunnel: [FALSE TRUE] -> w1592
                      frame False {
                        # "Ok, close tubro Valve"
                      }
                      frame True {
                        n359 = One Button Dialog(message="Please wait for Turbo to slow down first") -> ()  [unwired: 1 in, 1 out]
                      }
                    }
                  }
                  frame True {
                    n360 = One Button Dialog(message="Please Turn Turbo Off First") -> ()  [unwired: 1 in, 1 out]
                  }
                }
              }
              frame True {
                # "Vent Valve Open?"
                n361 = case shown="False" w1602 {
                  tunnel: [w1603 FALSE] -> w1601
                  tunnel: w1600 -> [w1604 _]
                  frame False {
                    # "Bypass Valve Open?"
                    n362 = case shown="True" w1604 {
                      tunnel: [TRUE FALSE] -> w1603
                      frame False {
                        # "Yes, Open Turbo Valve"
                      }
                      frame True {
                        n363 = One Button Dialog(message="Please Close Bypass Valve first") -> ()  [unwired: 1 in, 1 out]
                      }
                    }
                  }
                  frame True {
                    n364 = One Button Dialog(message="Please Close Vent Valve first") -> ()  [unwired: 1 in, 1 out]
                  }
                }
              }
            }
            n365 = case shown="True" w1445 {
              tunnel: [FALSE w1464] -> w1438
              tunnel: w1450 -> [_ w1465]
              tunnel: w1449 -> [_ w1463]
              tunnel: w1448 -> [_ w1462]
              tunnel: w1447 -> [_ w1461]
              tunnel: w1446 -> [_ w1460]
              tunnel: w1436 -> [_ w1459]
              tunnel: w1428 -> [_ w1458]
              frame False {
              }
              frame True {
                # "Vent Valve Open?"
                n366 = case shown="False" w1465 {
                  tunnel: [w1471 FALSE] -> w1464
                  tunnel: w1463 -> [w1472 _]
                  tunnel: w1462 -> [w1470 _]
                  tunnel: w1461 -> [w1469 _]
                  tunnel: w1460 -> [w1468 _]
                  tunnel: w1459 -> [w1467 _]
                  tunnel: w1458 -> [w1466 _]
                  frame False {
                    # "Primary Pump On?"
                    n367 = case shown="True" w1470 {
                      tunnel: w1472 -> [_ w1480]
                      tunnel: [FALSE w1479] -> w1471
                      tunnel: w1469 -> [_ w1478]
                      tunnel: w1468 -> [_ w1477]
                      tunnel: w1467 -> [_ w1476]
                      tunnel: w1466 -> [_ w1475]
                      frame False {
                        n368 = One Button Dialog(message="Please Turn Primary Pump On first") -> ()  [unwired: 1 in, 1 out]
                      }
                      frame True {
                        # "Bypass Valve Open?"
                        n369 = case shown="False" w1480 {
                          tunnel: [w1484 FALSE] -> w1479
                          tunnel: w1478 -> [w1485 _]
                          tunnel: w1477 -> [w1483 _]
                          tunnel: w1476 -> [w1482 _]
                          tunnel: w1475 -> [w1481 _]
                          frame False {
                            # "Turbo Valve Open?"
                            n370 = case shown="True" w1485 {
                              tunnel: [FALSE w1490] -> w1484
                              tunnel: w1483 -> [_ w1491]
                              tunnel: w1482 -> [_ w1489]
                              tunnel: w1481 -> [_ w1488]
                              frame False {
                                n371 = One Button Dialog(message="Please Open Turbo Valve first") -> ()  [unwired: 1 in, 1 out]
                              }
                              frame True {
                                # "Chiller On?"
                                n372 = case shown="True" w1491 {
                                tunnel: [FALSE w1496] -> w1490
                                tunnel: w1489 -> [_ w1495]
                                tunnel: w1488 -> [_ w1494]
                                frame False {
                                n373 = One Button Dialog(message="Please Turn Chiller On First") -> ()  [unwired: 1 in, 1 out]
                                }
                                frame True {
                                # "Main Facility Pressure Low Enough?"
                                n374 = Less?(x=w1495, y=0.01) -> (x < y?=w1497:bool)
                                n375 = case shown="True" w1497 {
                                tunnel: [FALSE w1502] -> w1496
                                tunnel: w1494 -> [_ w1501]
                                frame False {
                                n376 = One Button Dialog(message="Main Facility Pressure Too High") -> ()  [unwired: 1 in, 1 out]
                                }
                                frame True {
                                # "Foreline Pressure Low Enough?"
                                n377 = Less?(x=w1501, y=1.6) -> (x < y?=w1503:bool)
                                n378 = case shown="True" w1503 {
                                tunnel: [FALSE TRUE] -> w1502
                                frame False {
                                n379 = One Button Dialog(message="Foreline Pressure Too High") -> ()  [unwired: 1 in, 1 out]
                                }
                                frame True {
                                # "Ok. Turn on Turbo"
                                }
                                }
                                }
                                }
                                }
                                }
                              }
                            }
                          }
                          frame True {
                            n380 = One Button Dialog(message="Please Close Bypass Valve first") -> ()  [unwired: 1 in, 1 out]
                          }
                        }
                      }
                    }
                  }
                  frame True {
                    n381 = One Button Dialog(message="Please Close Vent Valve first") -> ()  [unwired: 1 in, 1 out]
                  }
                }
              }
            }
            n382 = case shown="False" w1451 {
              tunnel: [w1512 TRUE ("Chiller_User_Cmd")] -> w1439
              tunnel: w1435 -> [w1513 _]
              frame False {
                # "Turbo Motor On?"
                n383 = case shown="True" w1513 {
                  tunnel: [FALSE TRUE] -> w1512
                  frame False {
                    # "Ok, Turn Chiller Off."
                  }
                  frame True {
                    n384 = One Button Dialog(message="Please Turn Turbo Pump Off First") -> ()  [unwired: 1 in, 1 out]
                  }
                }
              }
              frame True {
              }
            }
            n385 = case shown="True" w1455 {
              tunnel: [FALSE w1573] -> w1442
              tunnel: w1450 -> [_ w1572]
              tunnel: w1435 -> [_ w1571]
              tunnel: w1453 -> [_ w1570]
              frame False {
              }
              frame True {
                # "Vent Valve Open?"
                n386 = case shown="True" w1572 {
                  tunnel: [w1575 FALSE] -> w1573
                  tunnel: w1571 -> [w1576 _]
                  tunnel: w1570 -> [w1574 _]
                  frame False {
                    # "Turbo Motor On?"
                    n387 = case shown="False" w1576 {
                      tunnel: [w1577 FALSE] -> w1575
                      tunnel: w1574 -> [w1578 _]
                      frame False {
                        # "Turbo Still Spinning?"
                        n388 = Greater?(x=w1578, y=5.0) -> (0:w1579:bool)
                        n389 = case shown="True" w1579 {
                          tunnel: [TRUE FALSE] -> w1577
                          frame False {
                            # "Ok. Open bypass valve"
                          }
                          frame True {
                            n390 = One Button Dialog(message="Please wait for Turbo to slow down first") -> ()  [unwired: 1 in, 1 out]
                          }
                        }
                      }
                      frame True {
                        n391 = One Button Dialog(message="Please Turn Turbo off First") -> ()  [unwired: 1 in, 1 out]
                      }
                    }
                  }
                  frame True {
                    n392 = One Button Dialog(message="Please Close Vent Valve first") -> ()  [unwired: 1 in, 1 out]
                  }
                }
              }
            }
            n393 = case shown="False" w1454 {
              tunnel: w1454 -> [_ _]
              tunnel: [w1553 w1564] -> w1440
              tunnel: w1450 -> [_ w1565]
              tunnel: w1435 -> [w1554 _]
              tunnel: w1453 -> [w1552 _]
              frame False {
                # "Turbo Motor On?"
                n394 = case shown="True" w1554 {
                  tunnel: [w1555 TRUE] -> w1553
                  tunnel: w1552 -> [w1557 _]
                  frame False {
                    # "Turbo Still Spinning?"
                    n395 = Greater?(x=w1557, y=5.0) -> (0:w1558:bool)
                    n396 = case shown="False" w1558 {
                      tunnel: [FALSE TRUE] -> w1555
                      frame False {
                        # "Ok, turn off Primary"
                      }
                      frame True {
                        n397 = One Button Dialog(message="Please wait for Turbo to slow down first") -> ()  [unwired: 1 in, 1 out]
                      }
                    }
                  }
                  frame True {
                    n398 = One Button Dialog(message="Please Turn Turbo Pump Off First") -> ()  [unwired: 1 in, 1 out]
                  }
                }
              }
              frame True {
                # "Is Vent Valve Open?"
                n399 = case shown="False" w1565 {
                  tunnel: [TRUE FALSE] -> w1564
                  frame False {
                    # "Ok, Turn On Primary"
                  }
                  frame True {
                    n400 = One Button Dialog(message="Please Close Vent Valve First") -> ()  [unwired: 1 in, 1 out]
                  }
                }
              }
            }
          }
          frame "Intialize" {
            # "Enable Switches?"
            n401 = Two Button Dialog(message="Select Control Mode", 1:"Admin" ("Center Button Text (\"No\")"), 2:"Auto" ("Right Button Text (\"Cancel\")")) -> (T button?=w1613:bool)
            n402 = case shown="True" w1613 {
              tunnel: [Facility_State."Admin" Facility_State."Auto"] -> w1619
              frame False {
              }
              frame True {
              }
            }
          }
          frame "Auto" {
            w1648 = Current_Facility_State."Facility Off" ("t")
            # "Sub_state_iteration"
            # "Turbo valve control"
            # "Bypass control"
            # "Vent control"
            # "Gate control"
            # "Command Primary"
            # "Command Turbo"
            # "Command Chiller"
            # "Enable Switches?"
            n403 = call <vilib>:"Simple Error Handler.vi"("error in (no error)"=w1645) -> ("code out"=w1642:i32)  [unwired: 4 in, 4 out]
            n404 = Greater Or Equal?(x=w1642, y=5000) -> (x >= y?=w1643:bool)
            n405 = Less Or Equal?(x=w1642, y=5010) -> (x <= y?=w1640:bool)
            n406 = And(x=w1643, y=w1640) -> (x .and. y?=w1639:bool)
            n407 = call <vilib>:"Simple Error Handler.vi"("error in (no error)"=w1645) -> ("error?"=w1638:bool)  [unwired: 4 in, 4 out]
            n408 = Or(x=w1639, y=w1638) -> (x .or. y?=w1633:bool)
            n409 = case shown="True" w1633 {
              tunnel: w1647 -> [w1686 w1692]
              tunnel: [w1686 w1691] -> w1646
              frame False {
              }
              frame True {
                n410 = Get Date/Time String(want seconds? (F)=TRUE) -> (time string=w1687:string)  [unwired: 2 in, 1 out]
                n411 = Concatenate Strings(w1692, "\r", "Shutt down due to error at " ("string"), w1687) -> (w1691:string)
              }
            }
            n412 = Select(t=w1648, s=w1633, f=w1650) -> (s? t:f=w1649:T2)
            n413 = Select(t=w1648, s=w1633, f=w1652) -> (s? t:f=w1651:T2)
            n414 = case shown="\"Pumping to Rough\"" w1651 {
              tunnel: w1632 -> [_ _ _ _ _ _ _ _]
              tunnel: w1683 -> [_ _ _ _ _ _ _ _]
              tunnel: w1682 -> [_ _ _ _ _ _ _ _]
              tunnel: w1681 -> [_ _ _ _ _ _ _ _]
              tunnel: w1680 -> [_ w1754 _ _ _ _ _ _]
              tunnel: w1679 -> [_ w1766 _ _ _ _ _ _]
              tunnel: w1678 -> [_ _ _ _ _ _ _ w2158]
              tunnel: w1677 -> [_ _ _ _ _ _ _ _]
              tunnel: w1676 -> [_ w1756 _ _ _ _ _ _]
              tunnel: w1675 -> [_ _ _ _ _ _ _ _]
              tunnel: w1674 -> [_ _ _ _ _ _ _ _]
              tunnel: w1673 -> [_ _ _ _ _ _ _ _]
              tunnel: w1672 -> [_ _ _ _ _ _ _ _]
              tunnel: [FALSE ("Valve_Turbo_User_Cmd") w1747 FALSE ("Valve_Turbo_User_Cmd") TRUE ("Valve_Turbo_User_Cmd") TRUE ("Valve_Turbo_User_Cmd") w2027 w2104 w2162] -> w1671
              tunnel: [FALSE ("Valve_Bypass_User_Cmd") w1751 FALSE ("Valve_Bypass_User_Cmd") w1902 FALSE ("Valve_Bypass_User_Cmd") w2022 FALSE ("Valve_Bypass_User_Cmd") FALSE ("Valve_Bypass_User_Cmd")] -> w1670
              tunnel: [FALSE ("Valve_Vent_User_Cmd") FALSE ("Valve_Vent_User_Cmd") FALSE ("Valve_Vent_User_Cmd") FALSE ("Valve_Vent_User_Cmd") FALSE ("Valve_Vent_User_Cmd") FALSE ("Valve_Vent_User_Cmd") w2115 w2156] -> w1669
              tunnel: [FALSE ("T button?") FALSE ("T button?") FALSE ("T button?") w1900 TRUE ("T button?") w2028 FALSE ("T button?") FALSE ("T button?")] -> w1668
              tunnel: [FALSE ("Primary_User_Cmd") TRUE ("Primary_User_Cmd") FALSE ("Primary_User_Cmd") TRUE ("Primary_User_Cmd") TRUE ("Primary_User_Cmd") TRUE ("Primary_User_Cmd") w2091 TRUE ("Primary_User_Cmd")] -> w1667
              tunnel: [FALSE ("Chiller_User_Cmd") w1799 w1841 TRUE ("Chiller_User_Cmd") TRUE ("Chiller_User_Cmd") TRUE ("Chiller_User_Cmd") w2091 TRUE ("Chiller_User_Cmd")] -> w1666
              tunnel: [w1715 w1771 w1868 w1896 w1985 w2025 w2118 w2169] -> w1659
              tunnel: w1649 -> [w1727 w1762 w1856 _ w2005 w2024 w2130 _]
              tunnel: [w1709 w1773 w1863 w1889 w1987 w2023 w2124 w2167] -> w1658
              tunnel: w1665 -> [_ w1801 w1846 w1888 _ _ w2144 w2183]
              tunnel: w1664 -> [_ w1798 _ w1887 _ w2034 w2145 _]
              tunnel: [FALSE ("Turbo_Error_Acknowlege_Cmd") w1798 FALSE ("Turbo_Error_Acknowlege_Cmd") w1897 w1990 w2020 w2145 w2160] -> w1654
              tunnel: w1662 -> [_ w1764 _ w1894 _ _ _ _]
              tunnel: w1661 -> [_ w1765 _ w1895 _ _ _ _]
              tunnel: w1660 -> [_ _ _ w1893 _ _ _ _]
              tunnel: w1657 -> [_ w1780 _ w1903 _ w2030 w2101 _]
              tunnel: [0 ("Sub_state_iteration") w1769 0 ("Sub_state_iteration") w1892 0 ("f") w2029 w2120 0 ("Sub_state_iteration")] -> w1656
              tunnel: w1646 -> [w1712 w1787 w1851 w1891 w2011 w2026 w2135 w2173]
              tunnel: [w1712 w1787 w1850 w1890 w2011 w2026 w2135 w2173] -> w1637
              tunnel: [T3."Facility Off" ("Tab Control") T3."Pumping to Rough" ("Tab Control") T3."Overnight Pump" ("Tab Control") T3."Engaging Turbo" ("Tab Control") T3."Pumping to Hig Vac" ("Tab Control") T3."Closing Gate" ("Tab Control") T3."Venting" ("Tab Control") T3."Turbo Slowing" ("Tab Control")] -> w1655
              tunnel: [FALSE w1768 FALSE ("Turbo_Error_Acknowlege_Cmd") FALSE ("Turbo_Error_Acknowlege_Cmd") w1979 w2018 w2105 FALSE ("Turbo_Error_Acknowlege_Cmd")] -> w1635
              tunnel: w1634 -> [_ w1768 _ _ w1979 w2019 w2105 _]
              frame "Facility Off", Default {
                n415 = Select(t=Current_Facility_State."Pumping to Rough", s="Pump to Rough", f=w1727) -> (s? t:f=w1724:T2)
                n416 = Select(t=Current_Facility_State."Pumping to High Vac", s="Pump to High Vac", f=w1724) -> (s? t:f=w1719:T2)
                n417 = Select(t=Current_Facility_State."Overnight Pump", s="Overnight Pump", f=w1719) -> (s? t:f=w1710:T2)
                n418 = Compound Arithmetic op=OR("Pump to Rough", "Pump to High Vac", "Overnight Pump") -> (w1728:bool)
                n419 = Select(t=Current_Facility_State."Pumping to Rough", s=w1728, f=Current_Facility_State."Facility Off") -> (s? t:f=w1716:T2)
                n420 = Select(t=Current_Facility_State."Venting", s="Vent", f=w1716) -> (s? t:f=w1715:T2)
                n421 = Select(t=Current_Facility_State."Vent and Shutdown", s="Vent", f=w1710) -> (s? t:f=w1709:T2)
              }
              frame "Pumping to Rough" {
                # "Time long enough"
                # "Open if lower, then keep open"
                # "For 10 mins"
                # "Turbo spinning?"
                # "Turn on Chiller?"
                n422 = Greater?(x=w1801, y=15.0) -> (0:w1763:bool)
                n423 = Equal?(x=0, y=w1780) -> (x = y?=w1757:bool)
                n424 = Multiply(x=60.0, y=1.0) -> (x*y=w1779:dbl)
                n425 = Equal?(x=Current_Facility_State."Overnight Pump", y=w1762) -> (x = y?=w1795:bool)
                n426 = Compound Arithmetic op=OR(w1763, w1757) -> (w1774:bool)
                n427 = call "Elapsed Time"("Time Target (s)"=w1779, "Reset"=w1757, "Auto Reset"=FALSE) -> ("Time has Elapsed"=w1759:bool)  [unwired: 9 in, 7 out]
                n428 = And(x=w1757, y=w1756) -> (x .and. y?=w1755:bool)
                n429 = Compound Arithmetic op=OR(w1759, TRUE, w1755) -> (w1758:bool)
                n430 = case shown="1" w1780 {
                  tunnel: [1 ("Sub_state_iteration") w1817 2] -> w1770
                  tunnel: w1758 -> [_ w1814 _]
                  tunnel: [w1807 w1814 TRUE] -> w1750
                  tunnel: w1765 -> [_ _ w1818]
                  tunnel: [FALSE ("Time has Elapsed") FALSE ("Time has Elapsed") w1826] -> w1752
                  tunnel: w1755 -> [w1810 _ _]
                  frame 0, Default {
                    n431 = Select(t=TRUE ("Skip Primary Warm"), s=w1810, f=FALSE ("Skip Primary Warm")) -> (s? t:f=w1807:bool)
                    n432 = local write "Skip Primary Warm"(w1807) -> ()
                  }
                  frame 1 {
                    n433 = Select(t=2, s=w1814, f=1 ("Sub_state_iteration")) -> (s? t:f=w1817:i32)
                  }
                  frame 2 {
                    w1819 = 1e-08  # Gauge Error Threshold
                    w1827 = 30.0  # Min time below threshhold (s)
                    # "And turbo valve open"
                    # "Drop below threshold long enough"
                    # "Foreline Pressure Reached?"
                    # "WRG Pressure reached?"
                    n434 = Greater?(x=w1818, y=w1819) -> (0:w1820:bool)
                    n435 = Less?(x=w1818, y="Turbo on Threshold (torr) 2") -> (x < y?=w1821:bool)
                    n436 = And(x=w1821, y=w1820) -> (x .and. y?=w1822:bool)
                    n437 = local write "Skip Primary Warm"(FALSE ("Skip Primary Warm")) -> ()
                    n438 = call "Is Value Changed.vim"("value"=w1822) -> ("changed or first call?"=w1829:bool)
                    n439 = case shown="True" w1822 {
                      tunnel: w1829 -> [_ w1837]
                      tunnel: [FALSE ("Time has Elapsed") w1835] -> w1826
                      tunnel: [0.0 ("Elapsed Time (s)") w1833] -> w1828
                      tunnel: w1827 -> [_ w1834]
                      frame False {
                      }
                      frame True {
                        n440 = call "Elapsed Time3"("Time Target (s)"=w1834, "Reset"=w1837, "Auto Reset"=FALSE) -> ("Elapsed Time (s)"=w1833:dbl, "Time has Elapsed"=w1835:bool)  [unwired: 9 in, 6 out]
                      }
                    }
                    "Elapsed Time (s)" <- w1828
                    "Turbo on Threshold (torr)" <- "Turbo on Threshold (torr) 2"
                  }
                }
                n441 = And(x=w1752, y=w1795) -> (x .and. y?=w1794:bool)
                n442 = Select(t=Current_Facility_State."Overnight Pump" ("x"), s=w1794, f=Current_Facility_State."Pumping to Rough") -> (s? t:f=w1790:T2)
                n443 = Equal?(x=Current_Facility_State."Pumping to High Vac" ("y"), y=w1762) -> (x = y?=w1775:bool)
                n444 = Or(x=w1775, y=w1774) -> (x .or. y?=w1799:bool)
                n445 = And(x=w1752, y=w1775) -> (x .and. y?=w1791:bool)
                n446 = Select(t=Current_Facility_State."Engage Turbo" ("x"), s=w1791, f=w1790) -> (s? t:f=w1784:T2)
                n447 = Select(t=Current_Facility_State."Overnight Pump", s="Overnight Pump 3", f=w1762) -> (s? t:f=w1744:T2)
                n448 = Select(t=Current_Facility_State."Pumping to Rough", s="Pump to Rough Only", f=w1744) -> (s? t:f=w1741:T2)
                n449 = Select(t=Current_Facility_State."Pumping to High Vac", s="Pump to High", f=w1741) -> (s? t:f=w1740:T2)
                n450 = Select(t=Current_Facility_State."Facility Off", s="Shut Off", f=w1784) -> (s? t:f=w1796:T2)
                n451 = Select(t=Current_Facility_State."Venting", s="Vent 2", f=w1740) -> (s? t:f=w1773:T2)
                n452 = Less?(x=w1765, y=w1764) -> (x < y?=w1767:bool)
                n453 = And(x=w1767, y=w1766) -> ()  [unwired: 1 out]
                n454 = Select(t=Current_Facility_State."Venting", s="Vent 2", f=w1796) -> (s? t:f=w1771:T2)
                n455 = Not Equal?(x=w1771, y=Current_Facility_State."Pumping to Rough") -> (x != y?=w1781:bool)
                n456 = case shown="False" w1781 {
                  tunnel: w1770 -> [w1838 _]
                  tunnel: [w1838 0 ("t")] -> w1769
                  frame False {
                  }
                  frame True {
                    n457 = local write "Skip Primary Warm"(FALSE ("Skip Primary Warm")) -> ()
                  }
                }
                n458 = Not Equal?(x=w1740, y=Current_Facility_State."Pumping to Rough") -> (x != y?=w1745:bool)
                n459 = Select(t=FALSE, s="Vent 2", f=w1750) -> (s? t:f=w1751:bool)
                n460 = Compound Arithmetic op=OR(FALSE, w1754, w1752) -> (w1753:bool)
                n461 = And(x=w1753, y=w1745) -> (x .and. y?=w1747:bool)
              }
              frame "Overnight Pump" {
                w1861 = Current_Facility_State."Pumping to Rough" ("t")
                w1866 = Current_Facility_State."Venting" ("t")
                # "Turbo spinning?"
                n462 = Greater?(x=w1846, y=10.0) -> (0:w1841:bool)
                n463 = Get Date/Time In Seconds() -> (seconds since 1Jan1904=w1849:timestamp)
                n464 = Greater?(x=w1849, y="Turbo Engage time") -> (0:w1844:bool)
                n465 = Select(t=Current_Facility_State."Pumping to High Vac", s=w1844, f=w1856) -> (s? t:f=w1855:T2)
                n466 = case shown="True" w1844 {
                  tunnel: w1851 -> [w1877 w1882]
                  tunnel: [w1877 w1881] -> w1850
                  frame False {
                  }
                  frame True {
                    n467 = Get Date/Time String(want seconds? (F)=TRUE) -> (time string=w1878:string)  [unwired: 2 in, 1 out]
                    n468 = Concatenate Strings(w1882, "\r", "Timestamp reached, turning on pumps at " ("string"), w1878) -> (w1881:string)
                  }
                }
                n469 = Select(t=Current_Facility_State."Pumping to Rough", s=w1844, f=Current_Facility_State."Overnight Pump") -> (s? t:f=w1853:T2)
                n470 = Select(t=w1866, s="Vent 4", f=w1853) -> (s? t:f=w1870:T2)
                n471 = Select(t=w1866, s="Vent 4", f=w1855) -> (s? t:f=w1865:T2)
                n472 = Select(t=w1861, s="Pump to Rough 3", f=w1870) -> (s? t:f=w1869:T2)
                n473 = Select(t=w1861, s="Pump to Rough 3", f=w1865) -> (s? t:f=w1864:T2)
                n474 = Select(t=Current_Facility_State."Pumping to High Vac", s="Pump to High Vac 3", f=w1864) -> (s? t:f=w1863:T2)
                n475 = Select(t=Current_Facility_State."Pumping to Rough", s="Pump to High Vac 3", f=w1869) -> (s? t:f=w1868:T2)
              }
              frame "Engage Turbo" {
                n476 = case shown="1" w1903 {
                  tunnel: [TRUE ("Valve_Bypass_User_Cmd") TRUE ("Valve_Bypass_User_Cmd") TRUE ("Valve_Bypass_User_Cmd") FALSE ("Valve_Bypass_User_Cmd") FALSE ("Valve_Bypass_User_Cmd") FALSE ("Valve_Bypass_User_Cmd")] -> w1902
                  tunnel: [FALSE ("T button?") FALSE ("T button?") FALSE ("T button?") FALSE ("T button?") TRUE ("T button?") TRUE ("T button?")] -> w1900
                  tunnel: [w1904 w1920 w1951 w1958 w1965 TRUE ("Turbo_Error_Acknowlege_Cmd")] -> w1897
                  tunnel: [Current_Facility_State."Engage Turbo" ("f") w1933 Current_Facility_State."Engage Turbo" ("f") Current_Facility_State."Engage Turbo" ("f") Current_Facility_State."Engage Turbo" ("f") Current_Facility_State."Pumping to High Vac" ("f")] -> w1896
                  tunnel: w1895 -> [_ w1913 _ _ _ _]
                  tunnel: w1894 -> [_ _ _ _ _ _]
                  tunnel: w1893 -> [_ w1936 _ _ _ _]
                  tunnel: [1 ("Sub_state_iteration") w1931 3 ("Sub_state_iteration") 4 ("f") 5 ("f") 0 ("f")] -> w1892
                  tunnel: w1891 -> [w1905 w1928 w1954 w1962 w1969 w1976]
                  tunnel: [w1905 w1927 w1954 w1962 w1969 w1976] -> w1890
                  tunnel: [Current_Facility_State."Pumping to High Vac" ("f") Current_Facility_State."Pumping to High Vac" ("Target Facility State") Current_Facility_State."Pumping to High Vac" ("f") Current_Facility_State."Pumping to High Vac" ("f") Current_Facility_State."Pumping to High Vac" ("f") Current_Facility_State."Pumping to High Vac" ("f")] -> w1889
                  tunnel: w1888 -> [_ w1922 _ _ _ _]
                  tunnel: w1887 -> [w1904 w1920 w1951 w1958 w1965 _]
                  frame 0, Default {
                    # "Init"
                  }
                  frame 1 {
                    w1912 = 1e-09  # WRG_Error_threshold
                    w1918 = 5.0  # Threshold_wiggle_room_multiplier
                    # "Foreline Pressuse"
                    # "WRG Pressuse"
                    # "Check safe to turn on turbo/open gate"
                    n477 = local read "Turbo on Threshold (torr)"() -> (w1919:dbl)
                    n478 = Multiply(x=w1919, y=w1918) -> (x*y=w1914:dbl)
                    n479 = Greater?(x=w1913, y=w1912) -> (0:w1911:bool)
                    n480 = Less?(x=w1913, y=w1914) -> (x < y?=w1916:bool)
                    n481 = Less?(x=w1936, y=w1914) -> (x < y?=w1935:bool)
                    n482 = And(x=w1911, y=w1916) -> (x .and. y?=w1915:bool)
                    n483 = Greater?(x=w1922, y=2.0) -> (0:w1921:bool)
                    n484 = And(x=w1915, y=w1935) -> (x .and. y?=w1924:bool)
                    n485 = Select(t=Current_Facility_State."Engage Turbo" ("f"), s=w1924, f=Current_Facility_State."Pumping to Rough") -> (s? t:f=w1933:T2)
                    n486 = Select(t=2, s=w1924, f=0 ("Sub_state_iteration")) -> (s? t:f=w1931:i32)
                    n487 = case shown="True" w1924 {
                      tunnel: w1928 -> [w1941 w1948]
                      tunnel: [w1942 w1949] -> w1927
                      tunnel: w1921 -> [w1940 w1947]
                      frame False {
                        n488 = Select(t="Pressure NOT low enough to open gate!" ("string"), s=w1940, f="Pressure NOT low enough to turn on turbo!" ("string")) -> (s? t:f=w1938:string)
                        n489 = Concatenate Strings(w1941, "\r", w1938) -> (w1942:string)
                      }
                      frame True {
                        n490 = Select(t="Pressure low enough to open gate" ("string"), s=w1947, f="Pressure low enough to turn on turbo" ("string")) -> (s? t:f=w1944:string)
                        n491 = Concatenate Strings(w1948, "\r", w1944) -> (w1949:string)
                      }
                    }
                  }
                  frame 2 {
                    # "Open turbo Valve"
                  }
                  frame 3 {
                    # "Close Bypass"
                  }
                  frame 4 {
                    # "Open Gate"
                  }
                  frame 5 {
                    # "Turn on Turbo"
                  }
                }
              }
              frame "Pumping to High Vac" {
                # "Keep Primary on?"
                # "Turn off Turbo?"
                n492 = Select(t=Current_Facility_State."Disengage Turbo", s="Shutdown", f=Current_Facility_State."Pumping to High Vac") -> (s? t:f=w2009:T2)
                n493 = Select(t=Current_Facility_State."Facility Off", s="Shutdown", f=w2005) -> (s? t:f=w2004:T2)
                n494 = Select(t=Current_Facility_State."Pumping to Rough", s="Pump to Rough 4", f=w2004) -> (s? t:f=w2003:T2)
                n495 = Select(t=Current_Facility_State."Disengage Turbo", s="Pump to Rough 4", f=w2009) -> (s? t:f=w2008:T2)
                n496 = Select(t=Current_Facility_State."Overnight Pump" ("f"), s="Overnight Pump 2", f=w2003) -> (s? t:f=w2002:T2)
                n497 = Select(t=Current_Facility_State."Disengage Turbo", s="Overnight Pump 2", f=w2008) -> (s? t:f=w2007:T2)
                n498 = Select(t=Current_Facility_State."Vent and Shutdown", s="Vent and shutdonw", f=w2002) -> (s? t:f=w1988:T2)
                n499 = Select(t=Current_Facility_State."Disengage Turbo", s="Vent and shutdonw", f=w2007) -> (s? t:f=w1986:T2)
                n500 = Compound Arithmetic op=OR("Shutdown", "Pump to Rough 4", "Overnight Pump 2", "Vent and shutdonw") -> (w1991:bool)
                n501 = Not(x=w1991) -> (.not. x?=w1990:bool)
                n502 = Select(t=Current_Facility_State."Disengage Turbo", s="Vent 5", f=w1986) -> (s? t:f=w1985:T2)
                n503 = Select(t=Current_Facility_State."Venting", s="Vent 5", f=w1988) -> (s? t:f=w1987:T2)
              }
              frame "Disengage Turbo" {
                n504 = case shown="2" w2030 {
                  tunnel: w2034 -> [w2041 w2055 w2082]
                  tunnel: [w2041 w2055 w2082] -> w2020
                  tunnel: [1 ("f") w2049 0 ("f")] -> w2029
                  tunnel: [FALSE ("T button?") FALSE ("T button?") FALSE ("T button?")] -> w2028
                  tunnel: [TRUE ("Valve_Turbo_User_Cmd") TRUE ("Valve_Turbo_User_Cmd") w2057] -> w2027
                  tunnel: [Current_Facility_State."Disengage Turbo" ("f") Current_Facility_State."Disengage Turbo" ("f") w2061] -> w2025
                  tunnel: w2024 -> [w2037 w2045 w2065]
                  tunnel: [w2037 w2045 w2065] -> w2023
                  tunnel: [FALSE FALSE w2071] -> w2022
                  tunnel: w2019 -> [w2035 w2043 w2060]
                  tunnel: [w2035 w2043 w2060] -> w2018
                  frame 0, Default {
                    # "Close gate"
                  }
                  frame 1 {
                    # "Wait 3 secs"
                    n505 = call "Elapsed Time2"("Time Target (s)"=1.0, "Auto Reset"=TRUE) -> ("Time has Elapsed"=w2051:bool)  [unwired: 10 in, 7 out]
                    n506 = Select(t=2 ("Sub_state_iteration"), s=w2051, f=1) -> (s? t:f=w2049:i32)
                  }
                  frame 2 {
                    # "Overnight pump"
                    # "Slowing down"
                    # "Close Turbo Valve"
                    n507 = Equal?(x=w2065, y=Current_Facility_State."Pumping to Rough" ("t")) -> (x = y?=w2071:bool)
                    n508 = Select(t=Current_Facility_State."Pumping to Rough", s=w2071, f=Current_Facility_State."Turbo slowing" ("y")) -> (s? t:f=w2067:T2)
                    n509 = Equal?(x=w2065, y=Current_Facility_State."Overnight Pump") -> (x = y?=w2069:bool)
                    n510 = Select(t=Current_Facility_State."Overnight Pump", s=w2069, f=w2067) -> (s? t:f=w2066:T2)
                    n511 = Equal?(x=w2065, y=Current_Facility_State."Vent and Shutdown") -> (x = y?=w2076:bool)
                    n512 = Equal?(x=w2065, y=Current_Facility_State."Venting") -> (x = y?=w2059:bool)
                    n513 = Or(x=w2076, y=w2059) -> (x .or. y?=w2075:bool)
                    n514 = Select(t=Current_Facility_State."Venting", s=w2075, f=w2066) -> (s? t:f=w2063:T2)
                    n515 = Equal?(x=w2065, y=Current_Facility_State."Facility Off") -> (x = y?=w2062:bool)
                    n516 = Select(t=Current_Facility_State."Turbo slowing", s=w2062, f=w2063) -> (s? t:f=w2061:T2)
                    n517 = Select(t=TRUE ("T button?"), s=w2059, f=FALSE ("T button?")) -> (s? t:f=w2057:bool)
                  }
                }
              }
              frame "Venting" {
                # "Close Turbo Vavle when \nventing is complete"
                # "For 10 mins"
                # "Open Vent valve"
                n518 = Greater?(x=w2144, y=15.0) -> (0:w2091:bool)
                n519 = Select(t=Current_Facility_State."Turbo slowing" ("y"), s=w2091, f=Current_Facility_State."Facility Off") -> (s? t:f=w2126:T2)
                n520 = Equal?(x=w2130, y=Current_Facility_State."Facility Off" ("t")) -> (x = y?=w2132:bool)
                n521 = Equal?(x=w2130, y=Current_Facility_State."Vent and Shutdown") -> (x = y?=w2114:bool)
                n522 = Or(x=w2114, y=w2132) -> (x .or. y?=w2131:bool)
                n523 = Select(t=w2126, s=w2131, f=Current_Facility_State."Venting") -> (s? t:f=w2137:T2)
                n524 = Equal?(x=w2101, y=0) -> (x = y?=w2106:bool)
                n525 = Select(t=Current_Facility_State."Facility Off", s=w2131, f=w2130) -> (s? t:f=w2097:T2)
                n526 = Multiply(x=10.0, y=60.0) -> (x*y=w2113:dbl)
                n527 = call "Elapsed Time4"("Time Target (s)"=w2113, "Reset"=w2106, "Auto Reset"=TRUE) -> ("Elapsed Time (s)"=→"Vent Time (s) 2":dbl, "Time has Elapsed"=w2108:bool)  [unwired: 9 in, 6 out]
                n528 = case shown="2" w2101 {
                  tunnel: [TRUE TRUE FALSE] -> w2116
                  tunnel: [1 ("Sub_state_iteration") w2151 2 ("Sub_state_iteration")] -> w2121
                  tunnel: w2108 -> [_ w2149 _]
                  frame 0, Default {
                  }
                  frame 1 {
                    n529 = Select(t=2, s=w2149, f=1 ("Sub_state_iteration")) -> (s? t:f=w2151:i32)
                  }
                  frame 2 {
                  }
                }
                n530 = Select(t=Current_Facility_State."Venting" ("f"), s=w2116, f=w2137) -> (s? t:f=w2100:T2)
                n531 = Select(t=Current_Facility_State."Pumping to Rough", s="Overnight Pump 5", f=w2100) -> (s? t:f=w2099:T2)
                n532 = Select(t=Current_Facility_State."Overnight Pump", s="Overnight Pump 5", f=w2097) -> (s? t:f=w2085:T2)
                n533 = Select(t=Current_Facility_State."Turbo slowing", s=w2091, f=Current_Facility_State."Facility Off") -> (s? t:f=w2092:T2)
                n534 = Select(t=w2092, s="Shut Off", f=w2099) -> (s? t:f=w2087:T2)
                n535 = Or(x=w2114, y=w2116) -> (x .or. y?=w2115:bool)
                n536 = Select(t=Current_Facility_State."Pumping to Rough", s="Pump to Rough 5", f=w2087) -> (s? t:f=w2086:T2)
                n537 = Select(t=Current_Facility_State."Pumping to Rough", s="Pump to Rough 5", f=w2085) -> (s? t:f=w2084:T2)
                n538 = Select(t=Current_Facility_State."Pumping to Rough", s="Pump to Hi vac", f=w2086) -> (s? t:f=w2118:T2)
                n539 = Select(t=Current_Facility_State."Pumping to High Vac", s="Pump to Hi vac", f=w2084) -> (s? t:f=w2124:T2)
                n540 = Not Equal?(x=w2118, y=Current_Facility_State."Venting") -> (x != y?=w2103:bool)
                n541 = Select(t=0, s=w2103, f=w2121) -> (s? t:f=w2120:i32)
                n542 = Select(t=FALSE, s=w2103, f=w2091) -> (s? t:f=w2104:bool)
              }
              frame "Turbo slowing" {
                n543 = Greater?(x=w2183, y=15.0) -> (0:w2181:bool)
                n544 = Select(t=Current_Facility_State."Turbo slowing" ("f"), s=w2181, f=Current_Facility_State."Facility Off") -> (s? t:f=w2170:T2)
                n545 = Select(t=Current_Facility_State."Pumping to Rough", s="Pump to High Vac 2", f=w2170) -> (s? t:f=w2169:T2)
                n546 = Select(t=Current_Facility_State."Pumping to High Vac", s="Pump to High Vac 2", f=Current_Facility_State."Facility Off" ("Target Facility State")) -> (s? t:f=w2167:T2)
                n547 = Select(t=TRUE, s="Pump to High Vac 2", f=FALSE ("Turbo_Error_Acknowlege_Cmd")) -> (s? t:f=w2160:bool)
                n548 = Select(t=FALSE, s="Pump to High Vac 2", f=TRUE ("Valve_Turbo_User_Cmd")) -> (s? t:f=w2162:bool)
                n549 = Select(t=FALSE, s="Pump to High Vac 2", f=w2158) -> (s? t:f=w2156:bool)
              }
            }
            "Tab Control" <- w1655
            n550 = case shown="True" w1654 {
              tunnel: [FALSE ("Turbo_Motor_User_Cmd") w1695] -> w1653
              tunnel: w1637 -> [w1693 w1697]
              tunnel: [w1693 w1696] -> w1636
              frame False {
              }
              frame True {
                n551 = local read "Turbo Convectron"() -> (w1699:dbl)
                n552 = Less?(x=w1699, y=5.0) -> (x < y?=w1695:bool)
                n553 = case shown="False" w1695 {
                  tunnel: w1697 -> [w1704 w1705]
                  tunnel: [w1703 w1705] -> w1696
                  frame False {
                    n554 = Get Date/Time String(want seconds? (F)=TRUE) -> (time string=w1701:string)  [unwired: 2 in, 1 out]
                    n555 = Concatenate Strings(w1704, "High pressure turbo shuttoff triggered at" ("string"), w1701) -> (w1703:string)
                  }
                  frame True {
                  }
                }
              }
            }
          }
        }
        n556 = Get Date/Time String(want seconds? (F)=TRUE) -> (date string=w1017:string, time string=w1018:string)  [unwired: 2 in]
        n557 = Concatenate Strings(w1018, "       " ("string"), w1017) -> (→"Current Time/date":string)
        n558 = Equal?(x=Facility_State."Auto", y=w1027) -> (x = y?=w1021:bool)
        n559 = Select(t="Auto Control Mode", s=w1021, f="Admin Control Mode") -> (s? t:f=→"String 3":string)
        n560 = Select(t=enum32{"Admin", "Debug", "Automatic"}."Automatic" ("Control Level"), s=w1021, f=enum32{"Admin", "Debug", "Automatic"}."Admin" ("Control Level")) -> (s? t:f=→"Control Level":enum32{"Admin", "Debug", "Automatic"})
        n561 = property on="Valve_Turbo_User_Cmd" class="Bool"("Visible"=w1008) -> ()  [unwired: 2 in, 2 out]
        n562 = property on="Turbo_Motor_User_Cmd" class="Bool"("Visible"=w1008) -> ()  [unwired: 2 in, 2 out]
        n563 = property on="Valve_Bypass_User_Cmd" class="Bool"("Visible"=w1008) -> ()  [unwired: 2 in, 2 out]
        n564 = property on="Valve_Gate_User_Cmd" class="Bool"("Visible"=w1008) -> ()  [unwired: 2 in, 2 out]
        n565 = property on="Valve_Vent_User_Cmd" class="Bool"("Visible"=w1008) -> ()  [unwired: 2 in, 2 out]
        n566 = property on="Chiller_User_Cmd" class="Bool"("Visible"=w1008) -> ()  [unwired: 2 in, 2 out]
        n567 = property on="Primary_User_Cmd" class="Bool"("Visible"=w1008) -> ()  [unwired: 2 in, 2 out]
        n568 = property on="Control Level" class="TabCtl (strict)"("Visible"=w1021) -> ()  [unwired: 2 in, 2 out]
        n569 = property on="Change to Auto" class="Bool"("Visible"=w1008) -> ()  [unwired: 2 in, 2 out]
        "String 4" <- "Admin Control Mode Enabled" ("String 4")
      }
      frame #4 {
        # "substate"
        # "Command Turbo"
        # "Command Chiller"
        # "Command Primary"
        # "Command"
        # "Command Valves"
        n570 = feedback #1() -> (w2206:bool)  [unwired: 1 in]
        n571 = Not Equal?(x=w2206, y=w2205) -> (x != y?=w2204:bool)
        n572 = feedback-in #1(w2205) -> ()
        n573 = local write "Valve_Gate_Sys_Cmd"(w2195) -> ()
        n574 = local write "Valve_Turbo_Sys_Cmd"(w2202) -> ()
        n575 = local write "Valve_Bypass_Sys_Cmd"(w2212) -> ()
        n576 = local write "Valve_Vent_Sys_Cmd"(w2213) -> ()
        n577 = local write "Turbo_Motor_Sys_Cmd"(w2225) -> ()
        n578 = feedback #2() -> (w2185:bool)  [unwired: 1 in]
        n579 = Not Equal?(x=w2185, y=w2184) -> (x != y?=w2186:bool)
        n580 = feedback-in #2(w2184) -> ()
        n581 = case shown="True" w2204 {
          frame False {
          }
          frame True {
            n582 = Wait (ms)(milliseconds to wait=u32 10000) -> ()  [unwired: 1 out]
          }
        }
        n583 = case shown="True" w2186 {
          frame False {
          }
          frame True {
            n584 = Wait (ms)(milliseconds to wait=u32 500) -> ()  [unwired: 1 out]
          }
        }
        n585 = local write "Primary_Sys_Cmd"(w2184) -> ()
        n586 = Build Array(w2202, w2212, w2213, w2195) -> (w2209:bool[])
        n587 = local write "Chiller_Sys_Cmd"(w2205) -> ()
        n588 = local read "Tubro_Control_Mode"() -> (w2201:T1)
        n589 = case shown="\"HP700_Turbo_RS485_Control\"" w2201 {
          tunnel: w2227 -> [w2255 w2284 w2316]
          tunnel: [w2257 w2284 w2316] -> w2226
          tunnel: w2225 -> [w2250 w2272 w2308]
          tunnel: w2224 -> [w2261 w2281 _]
          tunnel: [w2256 w2277 w2309] -> w2223
          tunnel: w2221 -> [w2254 w2283 w2315]
          tunnel: [w2254 w2283 w2315] -> w2220
          tunnel: w2219 -> [w2253 w2282 w2314]
          tunnel: [w2253 w2282 w2314] -> w2218
          tunnel: w2216 -> [w2252 w2280 w2310]
          tunnel: [w2252 w2279 w2310] -> w2217
          tunnel: [w2251 w2275 w2312] -> w2214
          tunnel: w2215 -> [w2251 w2276 w2313]
          tunnel: [w2250 w2272 w2308] -> w2211
          tunnel: w2188 -> [w2249 w2271 w2306]
          tunnel: [w2249 w2271 w2306] -> w2187
          frame "HP700_Turbo_RS485_Control" {
            # "Acknolege Errors?"
            n590 = local read "HP2300 RS485\nAddress"() -> (w2259:u16)
            n591 = Bundle By Name "Turbo Motor Control"(cluster=T6 {"Parameter"=2, "Parameter\nread only<->describe"=TRUE, "off<->on"=TRUE, "Rotation speed set value\nin rot. speed setting\noperations [%]"=nan, "Preset rotation Speed\nat Standby mode (%)"=nan, "maximum power\nsetpoint [%]"=0, "Gas mode"=0} ("Turn Turbo Motor On"), "off<->on"=w2250) -> (w2262:T6)
            n592 = call "PV Operating adjustment turbopump.vi"("Operating adjustment - Cluster"=w2262, "Adress of unit"=w2259, "VISA session"=w2255) -> ("error out"=w2260:errorcluster, "dup VISA session"=w2258:refnum<visa-resource-name>)  [unwired: 6 in, 1 out]
            n593 = case shown="True" w2261 {
              tunnel: w2260 -> [w2264 w2267]
              tunnel: w2259 -> [_ w2270]
              tunnel: w2258 -> [w2265 w2269]
              tunnel: [w2265 w2268] -> w2257
              tunnel: [w2264 w2266] -> w2256
              frame False {
              }
              frame True {
                n594 = call "PV Error Reset.vi"("Adress of unit"=w2270, "error in (no error)"=w2267, "VISA session"=w2269) -> ("error out"=w2266:errorcluster, "VISA resource out"=w2268:refnum<visa-resource-name>)  [unwired: 7 in]
              }
            }
          }
          frame "HP700_Turbo_DSUB25_Control", Default {
            # "Turbo Motor  Cmd"
            # "Turbo Error Acknoledged  Cmd"
            n595 = case shown="True" w2281 {
              tunnel: w2280 -> [w2286 w2293]
              tunnel: [w2286 w2290] -> w2279
              tunnel: [errorcluster {"status"=FALSE, "code"=0, "source"=""} ("error out") w2287] -> w2278
              frame False {
              }
              frame True {
                # "To acknowledge a turbo error, we must turn on this line for \n1 sec and off again"
                n596 = flat-sequence {
                  tunnel: w2293 -> [w2297]
                  tunnel: [w2296] -> w2292
                  tunnel: [w2295] -> w2288
                  tunnel: w2292 -> [w2300]
                  tunnel: [w2300] -> w2291
                  tunnel: [w2298] -> w2289
                  tunnel: w2288 -> [w2298]
                  tunnel: w2291 -> [w2305]
                  tunnel: [w2304] -> w2290
                  tunnel: w2289 -> [w2303]
                  tunnel: [w2302] -> w2287
                  frame #0 {
                    w2294 = TRUE ("element")
                    n597 = local write "Turbo Error Aknowleged"(w2294) -> ()
                    n598 = call-poly <vilib>:"DAQmx Write.vi"("task/channels in"=w2297, "data"=w2294) -> ("task out"=w2296:refnum<k21>, "error out"=w2295:errorcluster)  [unwired: 11 in, 1 out]
                  }
                  frame #1 {
                    n599 = Wait (ms)(milliseconds to wait=u32 1000) -> ()  [unwired: 1 out]
                  }
                  frame #2 {
                    w2301 = FALSE ("element")
                    n600 = local write "Turbo Error Aknowleged"(w2301) -> ()
                    n601 = call-poly <vilib>:"DAQmx Write.vi"("task/channels in"=w2305, "data"=w2301, "error in"=w2303) -> ("task out"=w2304:refnum<k21>, "error out"=w2302:errorcluster)  [unwired: 10 in, 1 out]
                  }
                }
              }
            }
            n602 = local read "Turbo Error Aknowleged"() -> (→"Turbo Error Aknowleged":bool)
            n603 = call-poly <vilib>:"DAQmx Write.vi"("task/channels in"=w2276, "data"=w2272) -> ("task out"=w2275:refnum<k21>, "error out"=w2274:errorcluster)  [unwired: 11 in, 1 out]
            n604 = Merge Errors(w2278, w2274) -> (w2277:errorcluster)
          }
          frame "BigRed_Turbo_DSUB_15_Control" {
            # "Turbo Motor  Cmd"
            n605 = local read "Turbo Error Aknowleged 2"() -> (→"Turbo Error Aknowleged 2":bool)
            n606 = Build Array(w2308, w2306) -> (w2307:bool[])
            n607 = call-poly <vilib>:"DAQmx Write.vi"("task/channels in"=w2313, "data"=w2307) -> ("task out"=w2312:refnum<k21>, "error out"=w2309:errorcluster)  [unwired: 11 in, 1 out]
          }
        }
        n608 = feedback #3() -> (w2199:bool)  [unwired: 1 in]
        n609 = Not Equal?(x=w2199, y=w2195) -> (x != y?=w2197:bool)
        n610 = feedback-in #3(w2195) -> ()
        n611 = feedback-in #4(w2209) -> ()
        n612 = feedback #4() -> (w2210:bool[])  [unwired: 1 in]
        n613 = Not Equal?(x=w2209, y=w2210) -> (x != y?=w2208:bool[])
        n614 = call-poly <vilib>:"DAQmx Write.vi"("task/channels in"=w2236, "data"=w2209) -> ("task out"=w2239:refnum<k21>, "error out"=w2238:errorcluster)  [unwired: 11 in, 1 out]
        n615 = Or Array Elements(Boolean array=w2208) -> (logical OR=w2207:bool)
        n616 = call-poly <vilib>:"DAQmx Write.vi"("task/channels in"=w2241, "data"=w2184) -> ("task out"=w2245:refnum<k21>, "error out"=w2231:errorcluster)  [unwired: 11 in, 1 out]
        n617 = Select(t=u32 9000, s=w2197, f=u32 1000 ("milliseconds to wait")) -> (s? t:f=w2198:u32)
        n618 = call-poly <vilib>:"DAQmx Write.vi"("task/channels in"=w2233, "data"=w2205) -> ("task out"=w2232:refnum<k21>, "error out"=w2228:errorcluster)  [unwired: 11 in, 1 out]
        n619 = case shown="False" w2207 {
          tunnel: w2198 -> [_ w2248]
          frame False {
          }
          frame True {
            n620 = Wait (ms)(milliseconds to wait=w2248) -> ()  [unwired: 1 out]
          }
        }
        n621 = Merge Errors(w2223) -> (w2222:errorcluster)
        n622 = Merge Errors(w2228, w2222) -> (w2229:errorcluster)
        n623 = Merge Errors(w2231, w2229) -> (w2230:errorcluster)
        n624 = Merge Errors(w2238, w2230) -> (w2237:errorcluster)
        n625 = Merge Errors(w2244, w2237) -> (w2243:errorcluster)
        "Primary_Sys_Cmd" <- w2184
        "Valve_Turbo_Sys_Cmd" <- w2202
        "Valve_Bypass_Sys_Cmd" <- w2212
        "Valve_Vent_Sys_Cmd" <- w2213
        "Chiller_Sys_Cmd" <- w2205
        "Turbo_Motor_Sys_Cmd" <- w2225
        "Turbo_Error_Acknowlege_Cmd" <- w2224
        "Valve_Gate_Sys_Cmd" <- w2195
        "Current Facility State" <- w2193
        "Target Facility State" <- w2192
        "Turbo_Standby_Sys_Cmd" <- w2188
      }
      frame #5 {
        n626 = feedback #5() -> (w2350:bool)  [unwired: 1 in]
        n627 = feedback-in #5(w2358) -> ()
        n628 = feedback #6() -> (w2352:bool)  [unwired: 1 in]
        n629 = feedback-in #6(w2347) -> ()
        n630 = feedback #7() -> (w2344:bool)  [unwired: 1 in]
        n631 = feedback-in #7(w2340) -> ()
        n632 = feedback #8() -> (w2355:bool)  [unwired: 1 in]
        n633 = feedback-in #8(w2370) -> ()
        n634 = Not Equal?(x=w2350, y=w2358) -> (x != y?=w2349:bool)
        n635 = Not Equal?(x=w2344, y=w2340) -> (x != y?=w2345:bool)
        n636 = Not Equal?(x=w2352, y=w2347) -> (x != y?=w2351:bool)
        n637 = feedback #9() -> (w2336:bool)  [unwired: 1 in]
        n638 = feedback-in #9(w2334) -> ()
        n639 = feedback #10() -> (w2331:bool)  [unwired: 1 in]
        n640 = feedback-in #10(w2328) -> ()
        n641 = feedback #11() -> (w2357:bool)  [unwired: 1 in]
        n642 = Not Equal?(x=w2357, y=w2348) -> (x != y?=w2356:bool)
        n643 = feedback-in #11(w2348) -> ()
        n644 = Wait Until Next ms Multiple(millisecond multiple=u32 100 ("milliseconds to wait")) -> ()  [unwired: 1 out]
        n645 = Not Equal?(x=w2355, y=w2370) -> (x != y?=w2354:bool)
        n646 = Not Equal?(x=w2336, y=w2334) -> (x != y?=w2335:bool)
        n647 = Not Equal?(x=w2331, y=w2328) -> (x != y?=w2332:bool)
        n648 = case shown="True" w2356 {
          tunnel: [w2455 w2463] -> w2353
          tunnel: w2348 -> [_ w2465]
          tunnel: "Opened" ("string") -> [_ w2460]
          tunnel: " Turbo Valve at " ("string") -> [_ w2459]
          tunnel: "Closed" ("f") -> [_ w2458]
          tunnel: w2346 -> [w2455 w2457]
          frame False {
          }
          frame True {
            n649 = Get Date/Time String(want seconds? (F)=TRUE) -> (time string=w2462:string)  [unwired: 2 in, 1 out]
            n650 = Select(t=w2460, s=w2465, f=w2458) -> (s? t:f=w2464:string)
            n651 = Concatenate Strings(w2457, "\r", w2464, w2459, w2462) -> (w2463:string)
          }
        }
        n652 = case shown="True" w2354 {
          tunnel: w2353 -> [w2444 w2450]
          tunnel: [w2444 w2452] -> w2360
          tunnel: w2370 -> [_ w2454]
          tunnel: "Opened" ("string") -> [_ w2448]
          tunnel: " Bypass Valve at " ("string") -> [_ w2447]
          tunnel: "Closed" ("f") -> [_ w2446]
          frame False {
          }
          frame True {
            n653 = Select(t=w2448, s=w2454, f=w2446) -> (s? t:f=w2453:string)
            n654 = Get Date/Time String(want seconds? (F)=TRUE) -> (time string=w2451:string)  [unwired: 2 in, 1 out]
            n655 = Concatenate Strings(w2450, "\r", w2453, w2447, w2451) -> (w2452:string)
          }
        }
        n656 = case shown="True" w2351 {
          tunnel: w2360 -> [w2433 w2439]
          tunnel: [w2433 w2441] -> w2359
          tunnel: w2347 -> [_ w2443]
          tunnel: "Opened" ("string") -> [_ w2437]
          tunnel: " Vent Valve at " ("string") -> [_ w2436]
          tunnel: "Closed" ("f") -> [_ w2435]
          frame False {
          }
          frame True {
            n657 = Get Date/Time String(want seconds? (F)=TRUE) -> (time string=w2440:string)  [unwired: 2 in, 1 out]
            n658 = Select(t=w2437, s=w2443, f=w2435) -> (s? t:f=w2442:string)
            n659 = Concatenate Strings(w2439, "\r", w2442, w2436, w2440) -> (w2441:string)
          }
        }
        n660 = case shown="True" w2349 {
          tunnel: w2359 -> [w2422 w2428]
          tunnel: [w2422 w2430] -> w2324
          tunnel: w2358 -> [_ w2432]
          tunnel: "Opened" ("string") -> [_ w2426]
          tunnel: " Gate Valve at " ("string") -> [_ w2425]
          tunnel: "Closed" ("f") -> [_ w2424]
          frame False {
          }
          frame True {
            n661 = Select(t=w2426, s=w2432, f=w2424) -> (s? t:f=w2431:string)
            n662 = Get Date/Time String(want seconds? (F)=TRUE) -> (time string=w2429:string)  [unwired: 2 in, 1 out]
            n663 = Concatenate Strings(w2428, "\r", w2431, w2425, w2429) -> (w2430:string)
          }
        }
        n664 = case shown="True" w2345 {
          tunnel: w2324 -> [w2411 w2413]
          tunnel: [w2411 w2419] -> w2333
          tunnel: w2340 -> [_ w2421]
          tunnel: "Started" ("string") -> [_ w2416]
          tunnel: " Primary Pump at " ("string") -> [_ w2415]
          tunnel: "Stopped" ("f") -> [_ w2414]
          frame False {
          }
          frame True {
            n665 = Select(t=w2416, s=w2421, f=w2414) -> (s? t:f=w2420:string)
            n666 = Get Date/Time String(want seconds? (F)=TRUE) -> (time string=w2418:string)  [unwired: 2 in, 1 out]
            n667 = Concatenate Strings(w2413, "\r", w2420, w2415, w2418) -> (w2419:string)
          }
        }
        n668 = case shown="True" w2335 {
          tunnel: w2333 -> [w2400 w2403]
          tunnel: [w2400 w2402] -> w2325
          tunnel: w2334 -> [_ w2410]
          tunnel: "Started" ("string") -> [_ w2406]
          tunnel: " Chiller at " ("string") -> [_ w2405]
          tunnel: "Stopped" ("f") -> [_ w2404]
          frame False {
          }
          frame True {
            n669 = Select(t=w2406, s=w2410, f=w2404) -> (s? t:f=w2409:string)
            n670 = Get Date/Time String(want seconds? (F)=TRUE) -> (time string=w2408:string)  [unwired: 2 in, 1 out]
            n671 = Concatenate Strings(w2403, "\r", w2409, w2405, w2408) -> (w2402:string)
          }
        }
        n672 = case shown="True" w2332 {
          tunnel: w2325 -> [w2389 w2391]
          tunnel: [w2389 w2397] -> w2327
          tunnel: w2328 -> [_ w2399]
          tunnel: "Started" ("string") -> [_ w2394]
          tunnel: " Turbo Pump at " ("string") -> [_ w2393]
          tunnel: "Stopped" ("f") -> [_ w2392]
          frame False {
          }
          frame True {
            n673 = Select(t=w2394, s=w2399, f=w2392) -> (s? t:f=w2398:string)
            n674 = Get Date/Time String(want seconds? (F)=TRUE) -> (time string=w2396:string)  [unwired: 2 in, 1 out]
            n675 = Concatenate Strings(w2391, "\r", w2398, w2393, w2396) -> (w2397:string)
          }
        }
        "String" <- w2327
      }
    }
    n676 = Not(x=w476) -> (.not. x?=w475:bool)
    "Running" <- w476
  }
  n677 = while {
    tunnel: w69 -> [w2476]
    shift-right: [w2503] -> w8
    shift-left: w2 -> [w2505]
    shift-right: [w2502] -> w7
    shift-left: w1 -> [w2504]
    stop <- w2532 stop-if-true
    n678 = Multiply(x=1000.0, y=w2476) -> (x*y=w2467:dbl)
    n679 = Wait Until Next ms Multiple(millisecond multiple=w2467) -> ()  [unwired: 1 out]
    n680 = local read "Primary_Pump_Read"() -> (w2531:bool)
    n681 = local read "Turbo Motor Read"() -> (w2520:bool)
    n682 = call-poly <vilib>:"DAQmx Read.vi"("task/channels in"=w2505, "error in"=w2504) -> ("task out"=w2503:refnum<k21>, "data"=w2471:waveform(dbl), "error out"=w2502:errorcluster)  [unwired: 11 in]
    n683 = local read "Wide Range Gauge Pressure (Torr)"() -> (w2501:dbl)
    n684 = local read "Bypass Valve"() -> (w2512:bool)
    n685 = local read "Turbo Valve"() -> (w2519:bool)
    n686 = local read "Gate Valve"() -> (w2511:bool)
    n687 = local read "Vent Valve"() -> (w2475:bool)
    n688 = local read "Foreline Convectron"() -> (w2497:dbl)
    n689 = local read "Turbo Convectron"() -> (w2485:dbl)
    n690 = Boolean To (0,1)(Boolean=w2531) -> (0, 1=w2530:i16)
    n691 = Boolean To (0,1)(Boolean=w2520) -> (0, 1=w2521:i16)
    n692 = Boolean To (0,1)(Boolean=w2519) -> (0, 1=w2518:i16)
    n693 = Boolean To (0,1)(Boolean=w2512) -> (0, 1=w2513:i16)
    n694 = Boolean To (0,1)(Boolean=w2511) -> (0, 1=w2510:i16)
    n695 = Boolean To (0,1)(Boolean=w2475) -> (0, 1=w2474:i16)
    n696 = To Double Precision Float(number=w2530) -> (double precision float=w2486:dbl)
    n697 = To Double Precision Float(number=w2521) -> (double precision float=w2487:dbl)
    n698 = To Double Precision Float(number=w2518) -> (double precision float=w2488:dbl)
    n699 = To Double Precision Float(number=w2513) -> (double precision float=w2489:dbl)
    n700 = To Double Precision Float(number=w2510) -> (double precision float=w2490:dbl)
    n701 = To Double Precision Float(number=w2474) -> (double precision float=w2473:dbl)
    n702 = Build Array(w2501) -> (w2500:dbl[])
    n703 = Build Array(w2497) -> (w2498:dbl[])
    n704 = Build Array(w2485) -> (w2496:dbl[])
    n705 = Build Array(w2486) -> (w2495:dbl[])
    n706 = Build Array(w2487) -> (w2494:dbl[])
    n707 = Build Array(w2488) -> (w2493:dbl[])
    n708 = Build Array(w2489) -> (w2492:dbl[])
    n709 = Build Array(w2490) -> (w2491:dbl[])
    n710 = Build Array(w2473) -> (w2472:dbl[])
    n711 = Bundle By Name(cluster=w2471, "Y"=w2500) -> (w2499:waveform(dbl))
    n712 = Bundle By Name(cluster=w2471, "Y"=w2498) -> (w2484:waveform(dbl))
    n713 = Bundle By Name(cluster=w2471, "Y"=w2496) -> (w2483:waveform(dbl))
    n714 = Bundle By Name(cluster=w2471, "Y"=w2495) -> (w2482:waveform(dbl))
    n715 = Bundle By Name(cluster=w2471, "Y"=w2494) -> (w2481:waveform(dbl))
    n716 = Bundle By Name(cluster=w2471, "Y"=w2493) -> (w2480:waveform(dbl))
    n717 = Bundle By Name(cluster=w2471, "Y"=w2492) -> (w2479:waveform(dbl))
    n718 = Bundle By Name(cluster=w2471, "Y"=w2491) -> (w2478:waveform(dbl))
    n719 = Bundle By Name(cluster=w2471, "Y"=w2472) -> (w2470:waveform(dbl))
    n720 = Build Array(w2499, w2484, w2483, w2482, w2481, w2480, w2479, w2478, w2470) -> (→"Waveform Chart 2":waveform(dbl)[])
    n721 = property on="Waveform Chart 2" class="WFChart (strict)"("Active Plot"=u32 8, "Plot.Plot Name"="Vent Valve") -> ()  [unwired: 2 in, 2 out]
    n722 = property on="Waveform Chart 2" class="WFChart (strict)"("Active Plot"=u32 0, "Plot.Plot Name"="Main Gauge") -> ()  [unwired: 2 in, 2 out]
    n723 = property on="Waveform Chart 2" class="WFChart (strict)"("Active Plot"=u32 1, "Plot.Plot Name"="Foreline Convectron") -> ()  [unwired: 2 in, 2 out]
    n724 = property on="Waveform Chart 2" class="WFChart (strict)"("Active Plot"=u32 2, "Plot.Plot Name"="Turbo Convectron") -> ()  [unwired: 2 in, 2 out]
    n725 = property on="Waveform Chart 2" class="WFChart (strict)"("Active Plot"=u32 3, "Plot.Plot Name"="Primary Pump") -> ()  [unwired: 2 in, 2 out]
    n726 = property on="Waveform Chart 2" class="WFChart (strict)"("Active Plot"=u32 4, "Plot.Plot Name"="Turbo Pump") -> ()  [unwired: 2 in, 2 out]
    n727 = property on="Waveform Chart 2" class="WFChart (strict)"("Active Plot"=u32 5, "Plot.Plot Name"="Turbo Valve") -> ()  [unwired: 2 in, 2 out]
    n728 = property on="Waveform Chart 2" class="WFChart (strict)"("Active Plot"=u32 6, "Plot.Plot Name"="Bypass Valve") -> ()  [unwired: 2 in, 2 out]
    n729 = property on="Waveform Chart 2" class="WFChart (strict)"("Active Plot"=u32 7, "Plot.Plot Name"="Gate Valve") -> ()  [unwired: 2 in, 2 out]
    n730 = local read "stop"() -> (w2532:bool)
  }
  n731 = call <vilib>:"DAQmx Stop Task.vi"("task/channels in"=w8, "error in"=w7) -> ("task out"=w10:refnum<k21>, "error out"=w9:errorcluster)  [unwired: 12 in]
  n732 = call <vilib>:"DAQmx Clear Task.vi"("task in"=w10, "error in"=w9) -> ()  [unwired: 13 in, 1 out]
  n733 = case shown="True" w66 {
    tunnel: w96 -> [w2534 w2538]
    tunnel: [w2534 w2536] -> w94
    tunnel: [errorcluster {"status"=FALSE, "code"=0, "source"=""} ("error out") w2535] -> w93
    frame False {
    }
    frame True {
      n734 = call-poly <vilib>:"DAQmx Write.vi"("task/channels in"=w2538, "data"=FALSE) -> ("task out"=w2536:refnum<k21>, "error out"=w2535:errorcluster)  [unwired: 11 in, 1 out]
    }
  }
  n735 = case shown="True" w66 {
    tunnel: w162 -> [w2540 w2544]
    tunnel: [w2540 w2543] -> w161
    tunnel: [errorcluster {"status"=FALSE, "code"=0, "source"=""} ("error out") w2542] -> w160
    frame False {
    }
    frame True {
      n736 = call-poly <vilib>:"DAQmx Write.vi"("task/channels in"=w2544, "data"=bool[] [FALSE, FALSE, FALSE, FALSE]) -> ("task out"=w2543:refnum<k21>, "error out"=w2542:errorcluster)  [unwired: 11 in, 1 out]
    }
  }
  n737 = case shown="False" w66 {
    tunnel: w159 -> [w2546 w2550]
    tunnel: [w2546 w2549] -> w158
    tunnel: [errorcluster {"status"=FALSE, "code"=0, "source"=""} ("error out") w2547] -> w157
    frame False {
    }
    frame True {
      n738 = call-poly <vilib>:"DAQmx Write.vi"("task/channels in"=w2550, "data"=FALSE) -> ("task out"=w2549:refnum<k21>, "error out"=w2547:errorcluster)  [unwired: 11 in, 1 out]
    }
  }
  n739 = case shown="True" w13 {
    tunnel: w14 -> [_ w2552]
    tunnel: w15 -> [_ w2551]
    frame False {
    }
    frame True {
      n740 = call "Close.vi"("error in (no error)"=w2552, "VISA resource name"=w2551) -> ()  [unwired: 9 in, 1 out]
    }
  }
  n741 = call <vilib>:"DAQmx Stop Task.vi"("task/channels in"=w94, "error in"=w93) -> ("task out"=w92:refnum<k21>, "error out"=w95:errorcluster)  [unwired: 12 in]
  n742 = local read "Tubro_Control_Mode"() -> (w54:T1)
  n743 = case shown="\"BigRed_Turbo_DSUB_15_Control\"" w54 {
    tunnel: w99 -> [_ _ w2614]
    tunnel: [w2567 w2595 w2613] -> w87
    tunnel: w82 -> [w2573 w2601 _]
    tunnel: w81 -> [w2570 w2598 _]
    tunnel: w44 -> [w2559 _ _]
    tunnel: w77 -> [w2556 w2592 _]
    tunnel: w66 -> [w2553 w2589 w2610]
    frame "HP700_Turbo_DSUB25_Control", Default {
      n744 = case shown="False" w2553 {
        tunnel: w2559 -> [w2579 w2587]
        tunnel: [w2579 w2586] -> w2558
        tunnel: [errorcluster {"status"=FALSE, "code"=0, "source"=""} ("error out") w2585] -> w2557
        tunnel: w2556 -> [w2576 w2583]
        tunnel: [w2576 w2582] -> w2555
        tunnel: [errorcluster {"status"=FALSE, "code"=0, "source"=""} ("error out") w2581] -> w2554
        frame False {
        }
        frame True {
          n745 = call-poly <vilib>:"DAQmx Write.vi"("task/channels in"=w2583, "data"=FALSE) -> ("task out"=w2582:refnum<k21>, "error out"=w2581:errorcluster)  [unwired: 11 in, 1 out]
          n746 = call-poly <vilib>:"DAQmx Write.vi"("task/channels in"=w2587, "data"=FALSE) -> ("task out"=w2586:refnum<k21>, "error out"=w2585:errorcluster)  [unwired: 11 in, 1 out]
        }
      }
      n747 = call <vilib>:"DAQmx Stop Task.vi"("task/channels in"=w2573) -> ("task out"=w2575:refnum<k21>, "error out"=w2574:errorcluster)  [unwired: 13 in]
      n748 = call <vilib>:"DAQmx Stop Task.vi"("task/channels in"=w2570) -> ("task out"=w2571:refnum<k21>, "error out"=w2572:errorcluster)  [unwired: 13 in]
      n749 = call <vilib>:"DAQmx Clear Task.vi"("task in"=w2575, "error in"=w2574) -> ("error out"=w2569:errorcluster)  [unwired: 13 in]
      n750 = call <vilib>:"DAQmx Clear Task.vi"("task in"=w2571, "error in"=w2572) -> ("error out"=w2568:errorcluster)  [unwired: 13 in]
      n751 = call <vilib>:"DAQmx Stop Task.vi"("task/channels in"=w2555, "error in"=w2554) -> ("task out"=w2562:refnum<k21>, "error out"=w2561:errorcluster)  [unwired: 12 in]
      n752 = call <vilib>:"DAQmx Stop Task.vi"("task/channels in"=w2558, "error in"=w2557) -> ("task out"=w2565:refnum<k21>, "error out"=w2566:errorcluster)  [unwired: 12 in]
      n753 = call <vilib>:"DAQmx Clear Task.vi"("task in"=w2562, "error in"=w2561) -> ("error out"=w2560:errorcluster)  [unwired: 13 in]
      n754 = call <vilib>:"DAQmx Clear Task.vi"("task in"=w2565, "error in"=w2566) -> ("error out"=w2564:errorcluster)  [unwired: 13 in]
      n755 = Merge Errors(w2564, w2560) -> (w2563:errorcluster)
      n756 = Merge Errors(w2569, w2568, w2563) -> (w2567:errorcluster)
    }
    frame "BigRed_Turbo_DSUB_15_Control" {
      n757 = case shown="True" w2589 {
        tunnel: w2592 -> [w2604 w2609]
        tunnel: [w2604 w2608] -> w2591
        tunnel: [errorcluster {"status"=FALSE, "code"=0, "source"=""} ("error out") w2607] -> w2590
        frame False {
        }
        frame True {
          n758 = call-poly <vilib>:"DAQmx Write.vi"("task/channels in"=w2609, "data"=FALSE) -> ("task out"=w2608:refnum<k21>, "error out"=w2607:errorcluster)  [unwired: 11 in, 1 out]
        }
      }
      n759 = call <vilib>:"DAQmx Stop Task.vi"("task/channels in"=w2601) -> ("task out"=w2603:refnum<k21>, "error out"=w2602:errorcluster)  [unwired: 13 in]
      n760 = call <vilib>:"DAQmx Stop Task.vi"("task/channels in"=w2598) -> ("task out"=w2599:refnum<k21>, "error out"=w2600:errorcluster)  [unwired: 13 in]
      n761 = call <vilib>:"DAQmx Clear Task.vi"("task in"=w2603, "error in"=w2602) -> ("error out"=w2597:errorcluster)  [unwired: 13 in]
      n762 = call <vilib>:"DAQmx Clear Task.vi"("task in"=w2599, "error in"=w2600) -> ("error out"=w2596:errorcluster)  [unwired: 13 in]
      n763 = call <vilib>:"DAQmx Stop Task.vi"("task/channels in"=w2591, "error in"=w2590) -> ("task out"=w2594:refnum<k21>, "error out"=w2593:errorcluster)  [unwired: 12 in]
      n764 = call <vilib>:"DAQmx Clear Task.vi"("task in"=w2594, "error in"=w2593) -> ("error out"=w2588:errorcluster)  [unwired: 13 in]
      n765 = Merge Errors(w2597, w2596, w2588) -> (w2595:errorcluster)
    }
    frame "HP700_Turbo_RS485_Control" {
      n766 = case shown="True" w2610 {
        tunnel: w2614 -> [w2616 w2626]
        tunnel: [w2616 w2620] -> w2612
        tunnel: [errorcluster {"status"=FALSE, "code"=0, "source"=""} ("error out") w2618] -> w2611
        frame False {
        }
        frame True {
          n767 = Bundle By Name "Turbo Motor Control"(cluster=T6 {"Parameter"=2, "Parameter\nread only<->describe"=TRUE, "off<->on"=TRUE, "Rotation speed set value\nin rot. speed setting\noperations [%]"=nan, "Preset rotation Speed\nat Standby mode (%)"=nan, "maximum power\nsetpoint [%]"=0, "Gas mode"=0} ("Turn Turbo Motor On"), "off<->on"=FALSE) -> (w2625:T6)
          n768 = local read "HP2300 RS485\nAddress"() -> (w2617:u16)
          n769 = call "PV Operating adjustment turbopump.vi"("Operating adjustment - Cluster"=w2625, "Adress of unit"=w2617, "VISA session"=w2626) -> ("error out"=w2619:errorcluster, "dup VISA session"=w2621:refnum<visa-resource-name>)  [unwired: 6 in, 1 out]
          n770 = call "PV Operating adjustment turbopump.vi"("error in (no error)"=w2619, "Operating adjustment - Cluster"=T6 {"Parameter"=1, "Parameter\nread only<->describe"=TRUE, "off<->on"=FALSE, "Rotation speed set value\nin rot. speed setting\noperations [%]"=50.0, "Preset rotation Speed\nat Standby mode (%)"=66.0, "maximum power\nsetpoint [%]"=100, "Gas mode"=0}, "Adress of unit"=w2617, "VISA session"=w2621) -> ("error out"=w2618:errorcluster, "dup VISA session"=w2620:refnum<visa-resource-name>)  [unwired: 5 in, 1 out]
        }
      }
      n771 = call "PV Close.vi"("VISA session"=w2612, "error in (no error)"=w2611) -> ("error out"=w2613:errorcluster)  [unwired: 13 in]
    }
  }
  n772 = call <vilib>:"DAQmx Stop Task.vi"("task/channels in"=w184) -> ("task out"=w186:refnum<k21>, "error out"=w187:errorcluster)  [unwired: 13 in]
  n773 = call <vilib>:"DAQmx Stop Task.vi"("task/channels in"=w161, "error in"=w160) -> ("task out"=w163:refnum<k21>, "error out"=w164:errorcluster)  [unwired: 12 in]
  n774 = call <vilib>:"DAQmx Stop Task.vi"("task/channels in"=w185) -> ("task out"=w209:refnum<k21>, "error out"=w207:errorcluster)  [unwired: 13 in]
  n775 = call <vilib>:"DAQmx Stop Task.vi"("task/channels in"=w158, "error in"=w157) -> ("task out"=w218:refnum<k21>, "error out"=w208:errorcluster)  [unwired: 12 in]
  n776 = call <vilib>:"DAQmx Stop Task.vi"("task/channels in"=w115) -> ("task out"=w116:refnum<k21>, "error out"=w117:errorcluster)  [unwired: 13 in]
  n777 = call <vilib>:"DAQmx Stop Task.vi"("task/channels in"=w132) -> ("task out"=w131:refnum<k21>, "error out"=w128:errorcluster)  [unwired: 13 in]
  n778 = call <vilib>:"DAQmx Clear Task.vi"("task in"=w92, "error in"=w95) -> ("error out"=w88:errorcluster)  [unwired: 13 in]
  n779 = call <vilib>:"DAQmx Clear Task.vi"("task in"=w186, "error in"=w187) -> ("error out"=w156:errorcluster)  [unwired: 13 in]
  n780 = call <vilib>:"DAQmx Clear Task.vi"("task in"=w163, "error in"=w164) -> ("error out"=w153:errorcluster)  [unwired: 13 in]
  n781 = call <vilib>:"DAQmx Clear Task.vi"("task in"=w209, "error in"=w207) -> ("error out"=w155:errorcluster)  [unwired: 13 in]
  n782 = call <vilib>:"DAQmx Clear Task.vi"("task in"=w218, "error in"=w208) -> ("error out"=w130:errorcluster)  [unwired: 13 in]
  n783 = call <vilib>:"DAQmx Clear Task.vi"("task in"=w116, "error in"=w117) -> ("error out"=w91:errorcluster)  [unwired: 13 in]
  n784 = call <vilib>:"DAQmx Clear Task.vi"("task in"=w131, "error in"=w128) -> ("error out"=w114:errorcluster)  [unwired: 13 in]
  n785 = Merge Errors(w87) -> (w86:errorcluster)
  n786 = Merge Errors(w88, w86) -> (w89:errorcluster)
  n787 = Merge Errors(w91, w89) -> (w90:errorcluster)
  n788 = Merge Errors(w114, w90) -> (w113:errorcluster)
  n789 = Merge Errors(w130, w113) -> (w129:errorcluster)
  n790 = Merge Errors(w155, w129) -> (w154:errorcluster)
  n791 = Merge Errors(w153, w154) -> (w152:errorcluster)
  n792 = Merge Errors(w156, w152) -> ()  [unwired: 1 out]
  "Use_real_Values?" <- "Use fake values?"
  "Tubro_Control_Mode" <- w55
